vi "BRig_RT_start_v1,13__PortC.vi"() -> ()   [LabVIEW 2014]
uses:
  myRIO_BRig_RT__Case_Exp_stateList.ctl
  myRIO_BRig_RT__Case_NonExp_stateList.ctl
  <vilib>/WebDAVClient/Advanced/SessionHandle.ctl
  <vilib>/Platform/TimedLoop/XDataNode/timing_clust.ctl
  <vilib>/Platform/TimedLoop/XDataNode/nitl_modes.ctl
  <vilib>/Platform/TimedLoop/XDataNode/wakeup.ctl
  <vilib>/myRIO/Common/Instrument Driver Framework/myRIO v1.0/UART/vis/myRIO v1.0 Close UART.vi
  <vilib>/FPGAPlugInAG/myRIO-1900/niLvFpga_Open_myRIO-1900.vi
  <vilib>/rvi/interface/common/dynamic/niFpgaDynamicAddResources.vi
  <vilib>/Utility/error.llb/Error Cluster From Error Code.vi
  <vilib>/rvi/errors/niLvFpgaAdjustHostInterfaceError.vi
  <vilib>/Utility/file.llb/Read From Spreadsheet File (I64).vi
  <vilib>/Utility/file.llb/Write To Spreadsheet File (DBL).vi
  <vilib>/FPGAPlugInAG/Dynamic/niLvFpga_Close_Dynamic.vi
  <vilib>/myRIO/Common/Instrument Driver Framework/Utilities/vis/FPGA Ref Manager.vi
  <vilib>/myRIO/Common/Instrument Driver Framework/myRIO v1.0/myRIO v1.0 Reset FPGA.vi
  <vilib>/myRIO/Common/Instrument Driver Framework/myRIO v1.0/IRQ/vis/myRIO v1.0 IRQ Info FGV.vi
  <vilib>/myRIO/Common/Instrument Driver Framework/myRIO v1.0/IRQ/vis/myRIO v1.0 Timer IRQ Info FGV.vi
  <vilib>/myRIO/Common/Instrument Driver Framework/myRIO v1.0/IRQ/vis/myRIO v1.0 ISR Agent.vi
  <vilib>/rvi/interface/nirviOpenFPGA/nirviOpenFPGA.xnode
  BRig_FPGA_v3,93__PortC__build.lvbitx
  BRig_FPGA_v3,93__PortC.vi
  <vilib>/rvi/interface/nirviReadWriteControl/nirviReadWriteControl.xnode
  <vilib>/Platform/TimedLoop/XDataNode/XDataNode.xnode
  <vilib>/rvi/interface/nirviCloseFPGA/nirviCloseFPGA.xnode
  <vilib>/Platform/TimedLoop/XDataNode/XDNodeRunTimeDep.lvlib
  <vilib>/rvi/interface/Simulation/niFpgaSimulationCallBeginRW.vi
  <vilib>/myRIO/Instrument Drivers/Utilities/Utilities.lvlib
  NiFpgaLv.dll
  <vilib>/WebDAVClient/NI_WebDAV.lvlib
panel:
  out "Solenoid R":bool
  out "Solenoid L":bool
  out "Laser2":bool
  out "Laser1":bool
  out "FreeReward_c_R":u16
  out "FreeReward_c_L":u16
  in  "Laser2_LED":bool
  in  "Laser1_LED":bool
  in  "lick_Rising(F)_or_Falling(T)":bool
  out "T_ExpRun_min":dbl
  out "stop_TimedLoop":bool
  out "BTPR_avg_R":dbl
  out "T2R_avg_R":dbl
  out "BTPR_avg_L":dbl
  out "T2R_avg_L":dbl
  out "BTPR_block":u16
  out "T2R_block":u16
  in  "comm_WebDAV_connect":bool
  in  "I_sendData":bool
  in  "comm_TCP_connect":bool
  out "nRewards_total":u16 caption="# Rewards in Current Block"
  out "BUR_target":u16 caption="Target Trials Per Block"
  in  "input_Threshold_reset":bool
  out "nTrial":u16
  out "allReward_R":bool
  out "allReward_L":bool
  out "Threshold":bool
  out "tLoop":dbl format="%#_2g"
  out "L_Power_l2":dbl
  out "comm_TCP":bool
  in  "get_countPerMS":bool
  out "SolenoidReward":bool
  out "L_Power_l1":dbl caption="LaserPower"
  in  "Recording":bool
  out "FPGA_count2ms":dbl=159.0
  out "error out":errorcluster
  out "cSpout":enum16{"Left", "Right"}(ring) caption="Left or Right Spout"
  out "A4":u32 caption="LickCounter_Right"
  out "A2":u32 caption="LickCounter_Left"
  out "nRewards_Right":u16 caption="# Rewards Total (Right)"
  out "nRewards_Left":u16 caption="# Rewards Total (Left)"
  out "nRewards_cur":u16 caption="# Rewards in Current Block"
  out "TpB_target":u16 caption="Target Trials Per Block"
  out "cState_NonExp":T1 caption="WarmUp State"
  out "iBlock":u16 caption="Current Block"
  out "cState":T2 caption="Experimental State"
  out "iTrial":u16 caption="Current Trial"
  in  "Data Set Prefix":string="Exp1_TM2"
  out "comm_WebDAV":bool
  in  "Host Password":string="sabalab"
  in  "Host UserName":string="Test2"
  in  "STOP_abort":bool caption="Stop LabView\n(Stops myRio and FPGA)"
  in  "STOP_endBlock":bool caption="Stop Experiment\n@ End of Block"
  in  "STOP_endTrial":bool caption="Stop Experiment\n@ End of Trial"
  in  "START":bool caption="Start Experiment"
  # "Experimental Run"
  # "Recording Rig"
  # "FPGA Conversion\n[counts per ms]"
  # "RealTime Cycle\nShould be <5ms"
  # "STOP experiment at"
  # "Exp Run Time"
  # "Reset"
  # "min"
  # "Communication with Host"
  # "Lick Counter"
  # "Give Water?\n(Reward)"
  # "Experimental State"
  # "Left/Right"
  # "Left           Right"
  # "Direction\n(NonSpecific Licking)"
  # "Block Target"
  # "# Blocks"
  # "L          R"
  # "# Trials"
  # "# Rewards"
  # "Bad Trials\nPost Reward"
  # "Trials 2 Reward"
  # "Block"
  # "# Trials"
  # "# Rewards"
  # "Current\nBlock"
  # "WarmUp State"
  # "avg L"
  # "Total"
  # "# Rewards"
  # "# Trials"
  # "avg R"
  # "Laser Power [V]"
  # "Left           Right"
  # "FreeRewards"
  # "Laser1"
  # "Laser2"
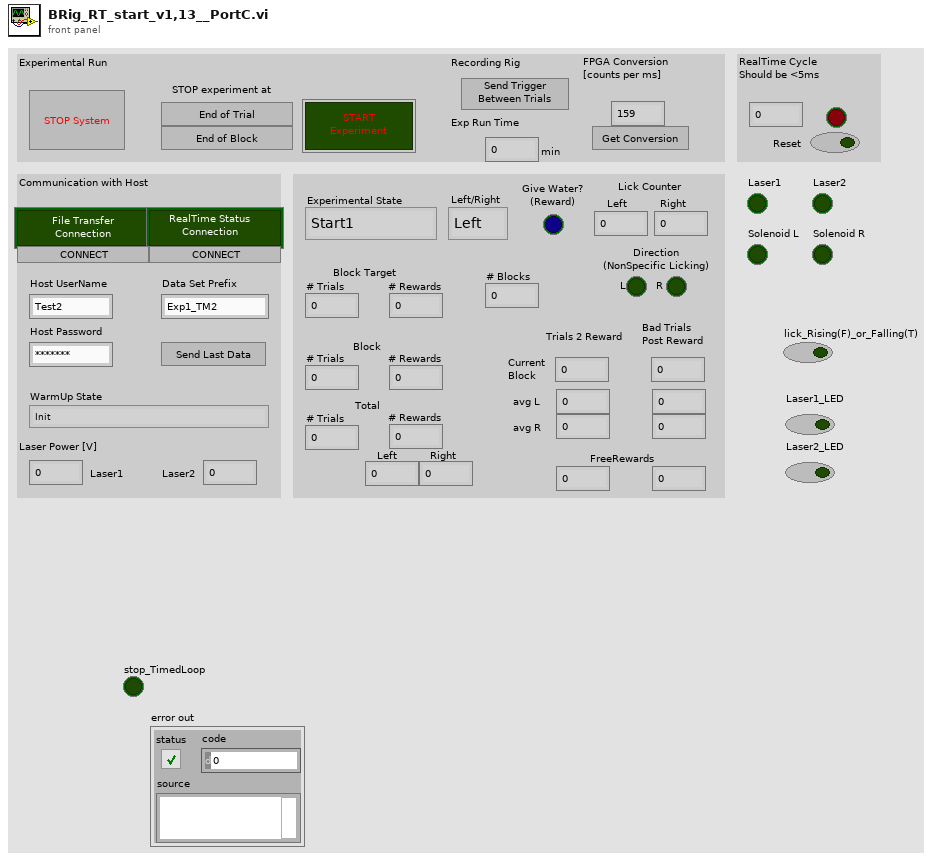
[diagram p1: front panel]
types:
  T1 = typedef "myRIO_BRig_RT__Case_NonExp_stateList.ctl" = enum16{"Init", "UploadSettings_pre", "UploadSettings_Read_dataExp", "UploadSettings_dataExp_1", "UploadSettings_dataExp_2", "UploadSettings_Read_dataLC", "UploadSettings_dataLC_1", "UploadSettings_dataLC_2", "UploadSettings_dataLC_3", "UploadSettings_dataLC_4", "UploadSettings_Read_dataMTrig", "UploadSettings_dataMTrig_1", "UploadSettings_post", "Idle_pre", "IdleEmpty", "IdleEmpty2", "IdleEmpty3", "IdleEmpty4", "Idle", "Idle_2", "Idle_3", "Idle_4", "Idle_5", "Idle_6", "Idle_post", "Cue_pre__pre", "Cue_pre", "Cue", "Cue_LED", "Cue_post", "RewardCalibration_pre", "RewardCalibration", "DispenseWater_pre__pre", "DispenseWater_pre", "DispenseWater", "DispenseWater_post", "TestConnection", "SendData", "Get_FPGA_count_per_ms", "End", "commTCP_connect"}
  T2 = typedef "myRIO_BRig_RT__Case_Exp_stateList.ctl" = enum16{"Start1", "Start2", "Start3", "saveSettings1", "saveSettings2", "saveSettings3", "saveSettings4", "saveSettings_LC_ENL_l1", "saveSettings_LC_ENL_l2", "saveSettings_LC_Cue_l1", "saveSettings_LC_Cue_l2", "saveSettings6_LC_l1_Other", "SaveSettings6_LC_l2_Other", "setSettings_Audio", "setSettings_Laser", "initBlock_pre", "initBlock", "initBlock2", "initBlock_post", "initTrial_pre", "initTrial", "initTrial2", "initTrial3", "initTrial4", "initTrial_LC_ENL1", "initTrial_LC_Cue1", "initTrial_LC_Cue1_2", "initTrial_LC_Sel", "initTrial_post", "ENL1_pre", "ENL1", "ENL1_post", "ENL1Penalty_pre", "ENL1Penalty", "ENL2_pre", "ENL2", "ENL2Penalty_pre", "ENL2Penalty", "Cue1_pre", "Cue1", "Cue1_post", "Cue1Penalty_pre", "Cue1Penalty", "Cue2_pre", "Cue2", "Cue2Penalty_pre", "Cue2Penalty", "Selection_pre", "Selection", "Select_post", "SelectReward_pre", "SelectReward", "SelectRewardPost_pre", "SelectRewardPost", "SelectWrong_pre", "SelectWrong", "SelectWrong_post", "SelectTimeout_pre", "SelectTimeout", "SelectTimeout_post", "endTrial_pre", "endTrial1", "endTrial2", "endTrial3", "endTrial_post", "endBlock_pre", "endBlock", "endBlock_post", "endExp", "commConnect", "commUpload_pre", "commUpload_dataBlock", "commUpload_dataCurrent", "commUpload_dataExp", "commUpload_dataLC", "commUpload_dataTrial", "commUpload_post", "saveData_pre", "saveData_dataBlock", "saveData_dataCurrent", "saveData_dataExp", "saveData_dataLC", "saveData_dataTrial", "saveData_post", "empty_endBlock1", "empty_endBlock2", "empty_endTrial1", "empty_endTrial2", "empty_endTrial3", "empty_endTrial4", "empty_endTrial5", "dummyState", "dummyState_endBlock", "FreeReward_pre", "FreeReward", "FreeRewardPost_pre", "FreeRewardPost"}
  T3 = enum8{"Enabled", "Disabled", "Disabled and Grayed Out"}
  T4 = typedef "NI_WebDAV.lvlib/SessionHandle.ctl" = refnum<k1>
  T5 = typedef "XDNodeRunTimeDep.lvlib/timing_clust.ctl" = cluster{"Expected End [f-1]":u64, "Actual End [f-1]":u64, "Finished Late? [f-1]":bool, "Expected End [i-1]":u64, "Actual End [i-1]":u64, "Finished Late? [i-1]":bool, "Expected Start [i]":u64, "Actual Start [i]":u64, "Expected Start [f]":u64, "Actual Start [f]":u64, "Source Name":string, "Structure Name":string, "Period":i64, "Deadline":i64, "Offset":i64, "Start":i64, "Priority":i32, "Timeout":i32, "Mode":T6, "Wakeup Reason":T7, "Error":errorcluster, "Source Type":string, "Secondary Source Type":string, "Global End Time":u64, "Global Start Time":u64, "Frame Duration":u64, "Iteration Duration":u64, "Assigned CPU":i32, "I/O Scan Engine Mode":u32}
  T6 = typedef "XDNodeRunTimeDep.lvlib/nitl_modes.ctl" = enum32{"No Change", "Process missed periods, maintain original phase", "Discard missed periods, maintain original phase", "Process missed periods, ignore original phase", "Discard missed periods, ignore original phase"}
  T7 = typedef "XDNodeRunTimeDep.lvlib/wakeup.ctl" = enum32{"Normal", "Aborted", "Asynchronous wakeup", "Timing source error", "Timed loop error", "Timeout"}
  T8 = cluster{"read mode":enum16{"polling", "blocking"}, "write mode":enum16{"polling", "blocking"}}
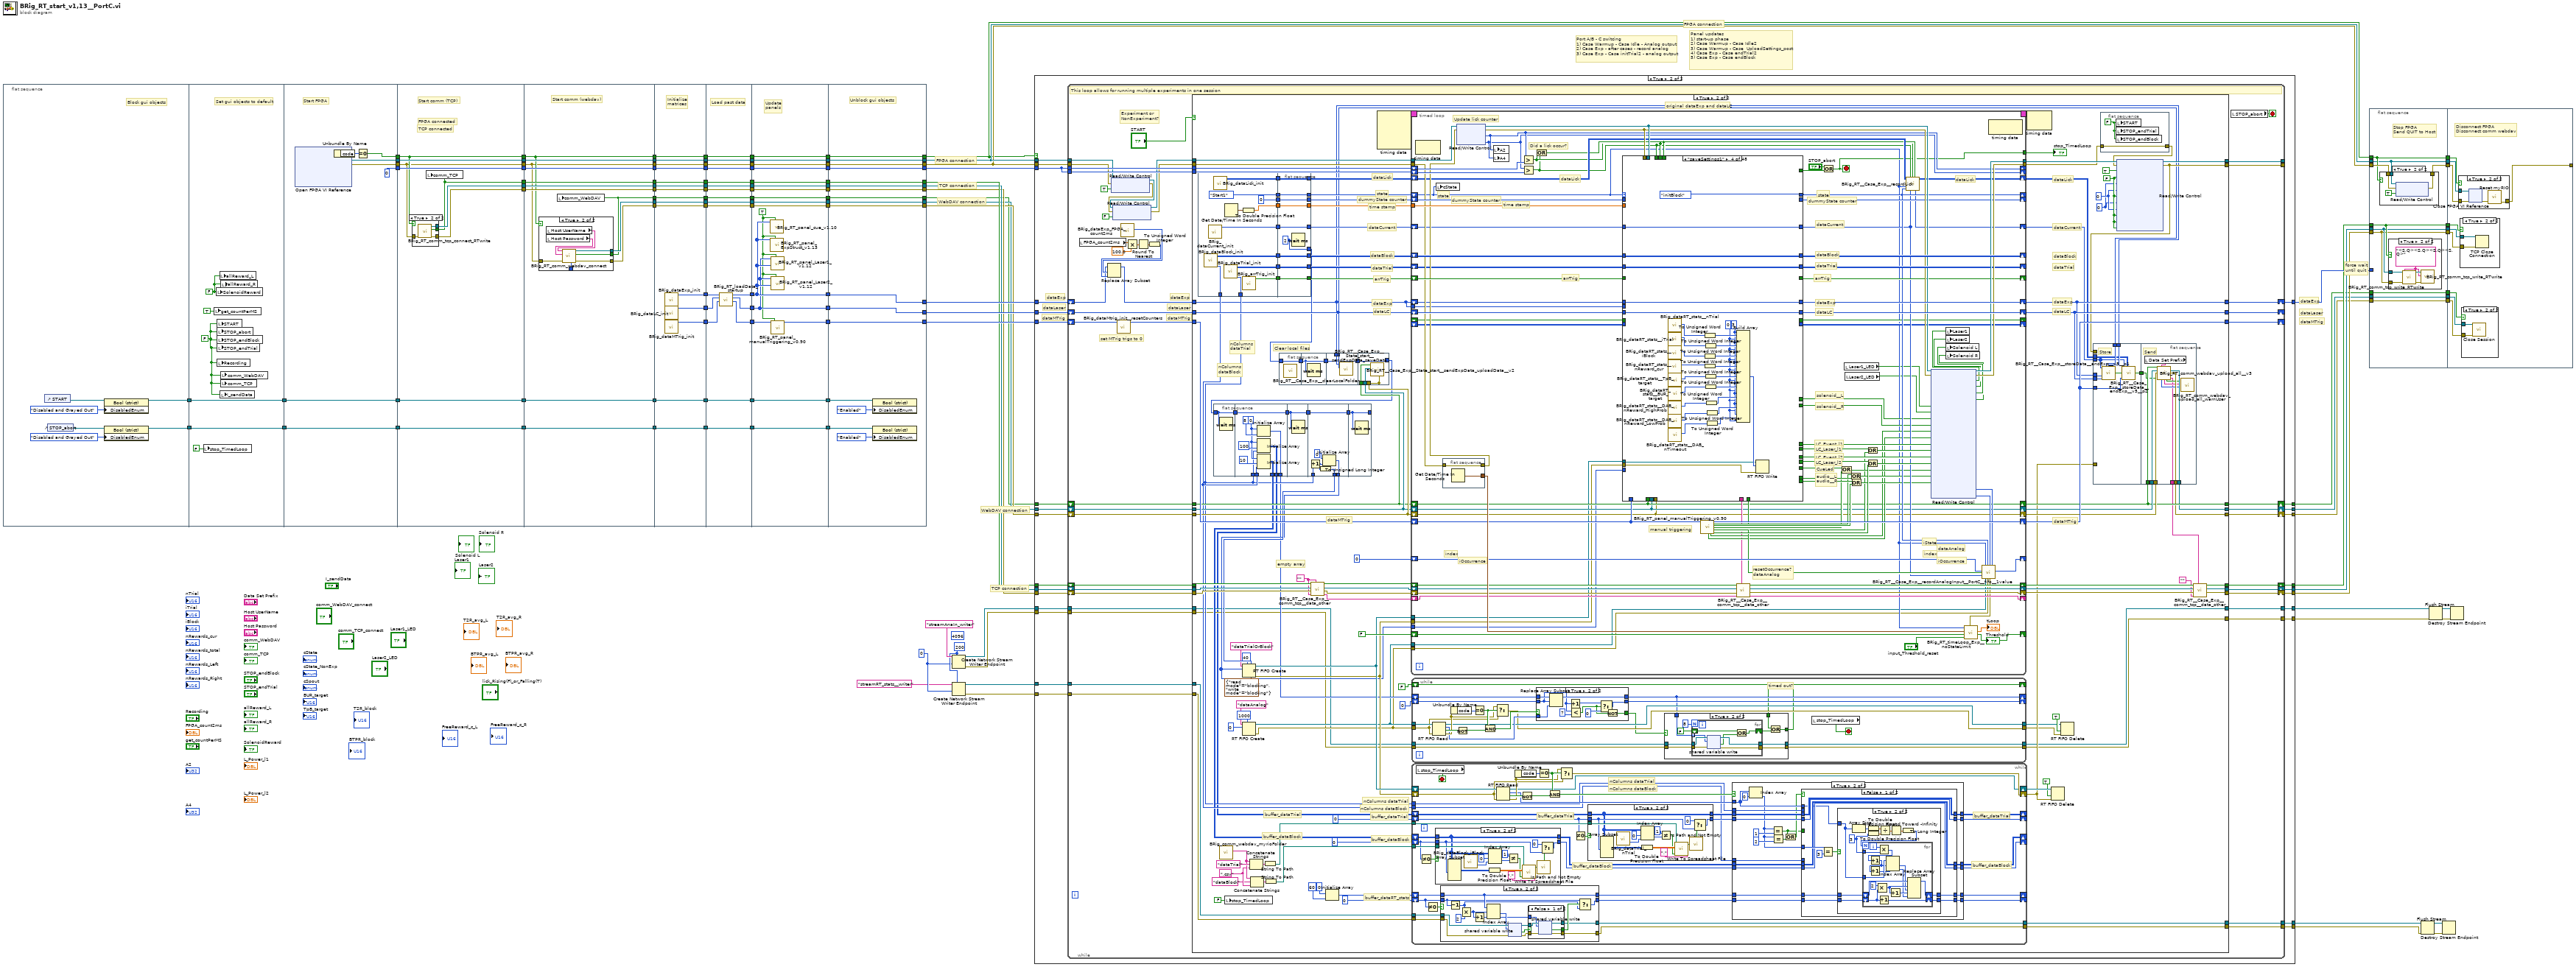
[diagram p0: block diagram]
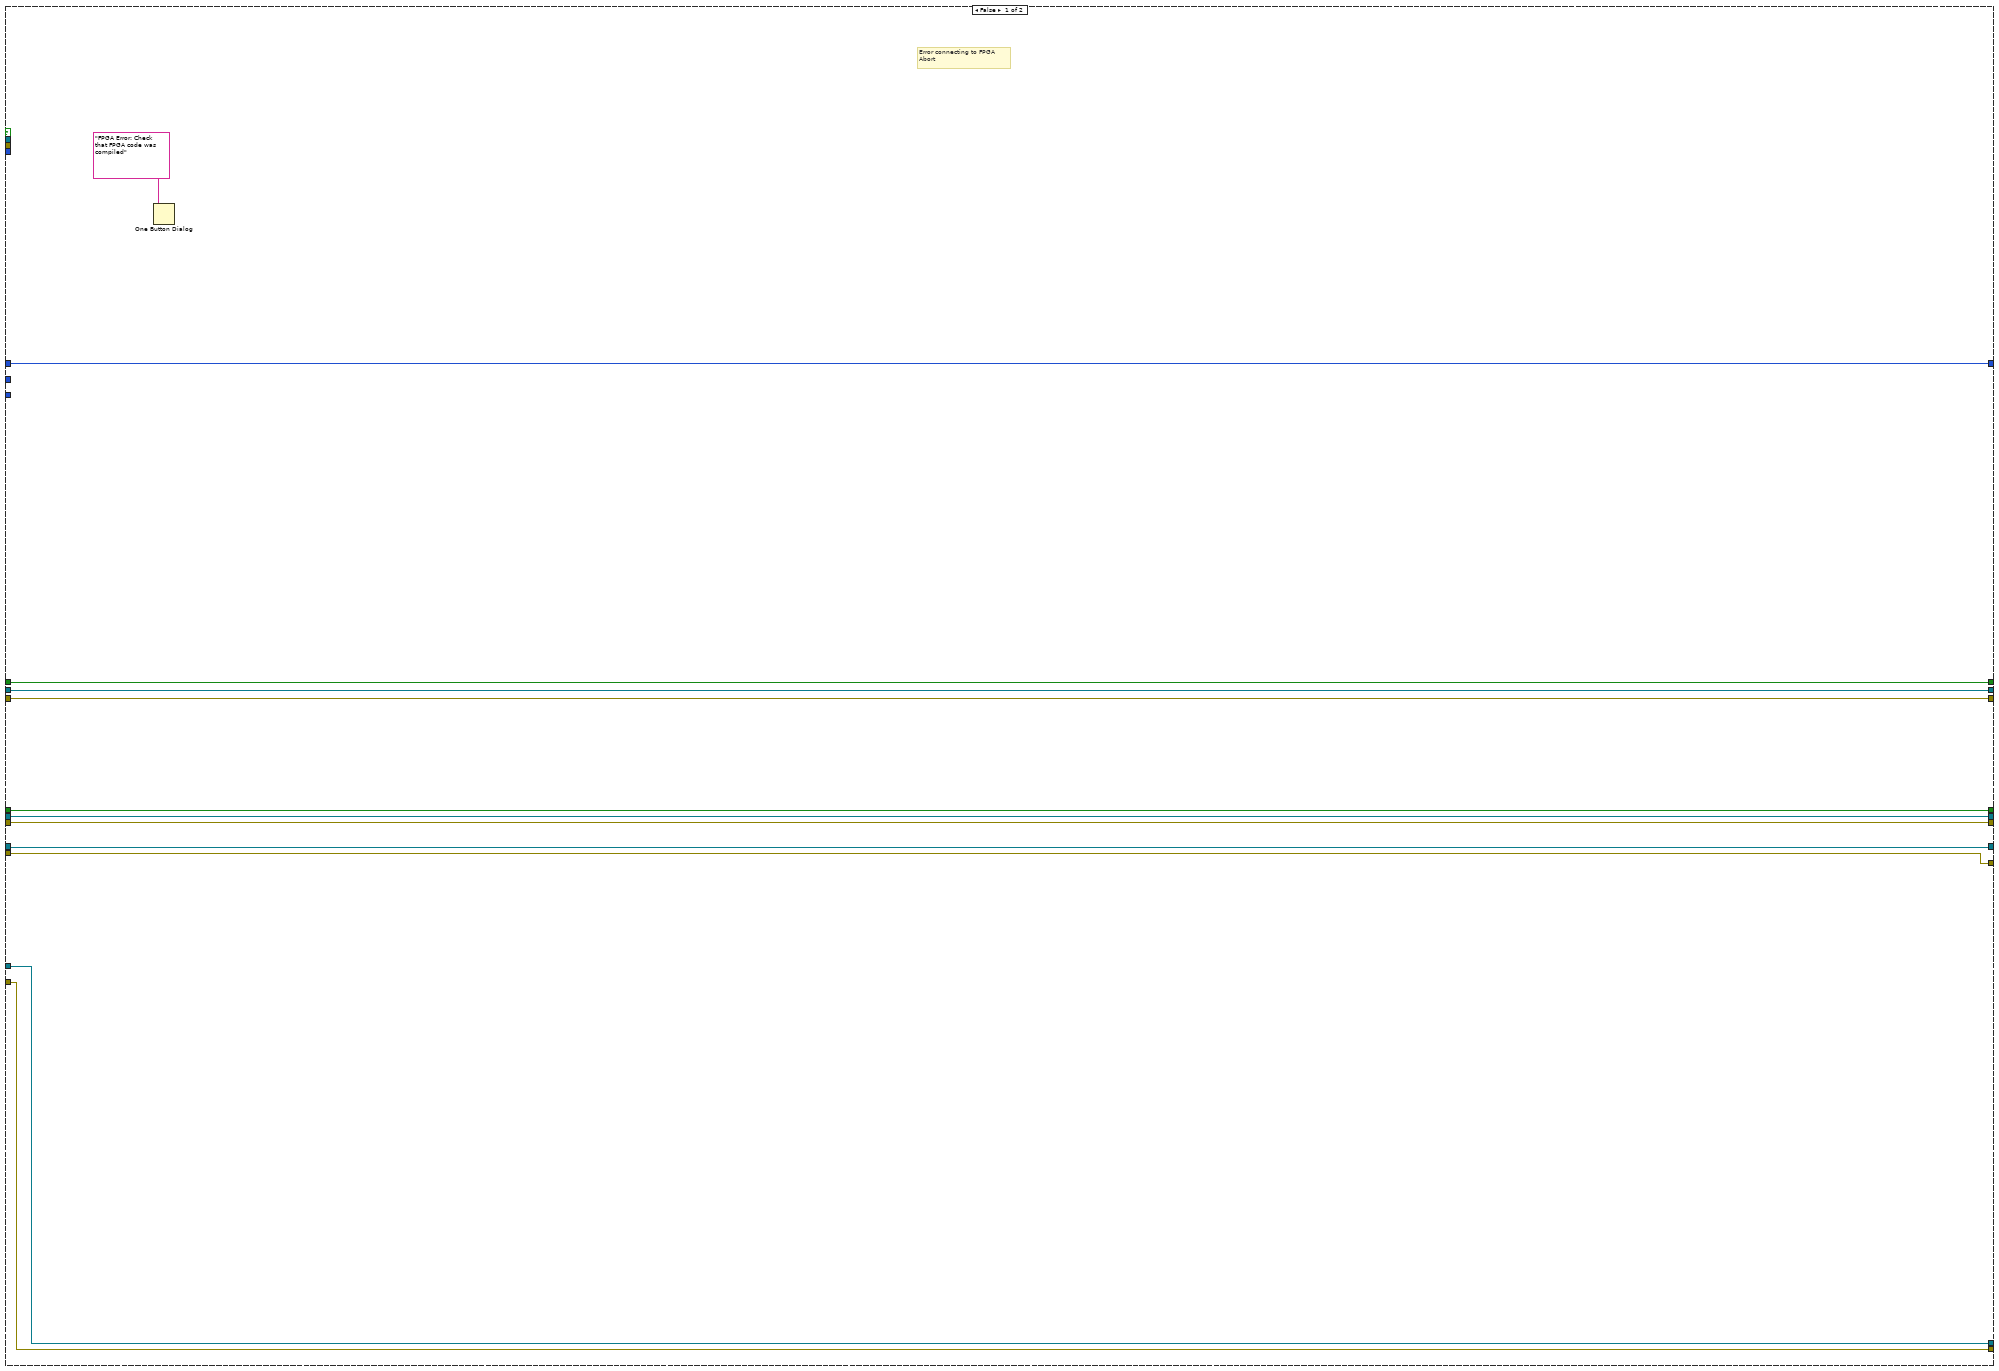
[diagram p2: hidden frame]
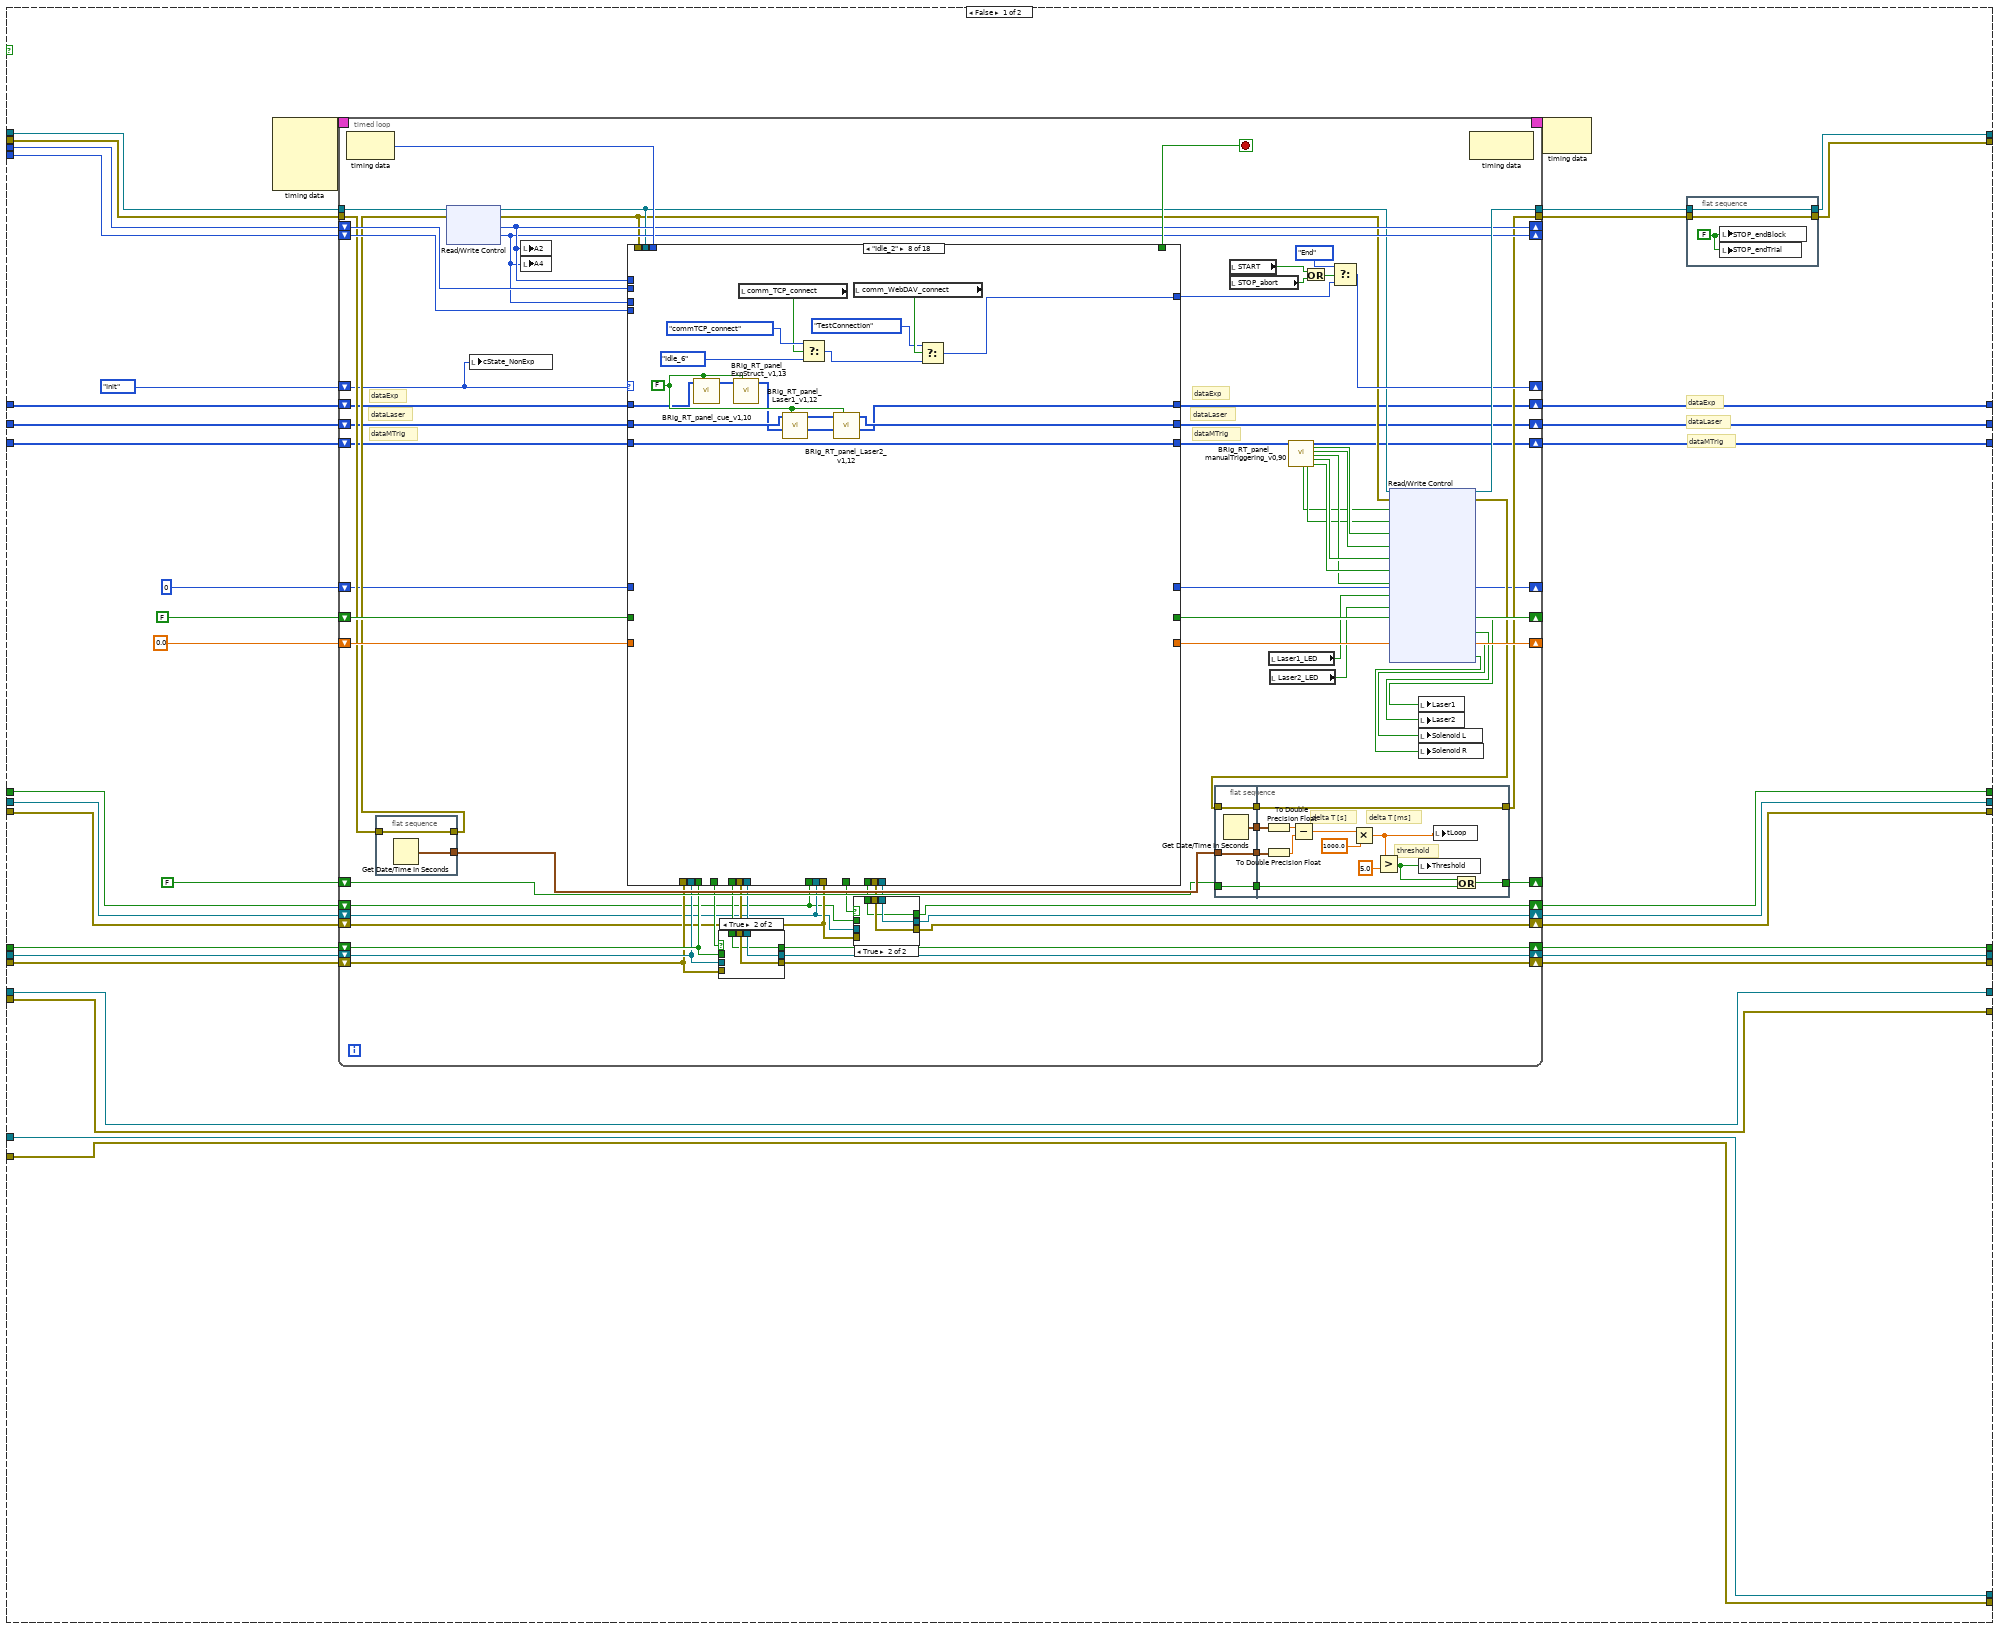
[diagram p3: hidden frame]
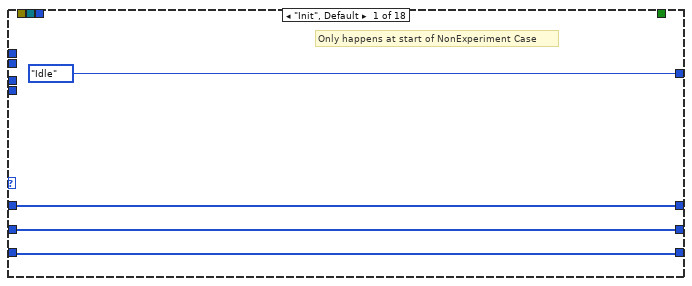
[diagram p6: hidden frame]
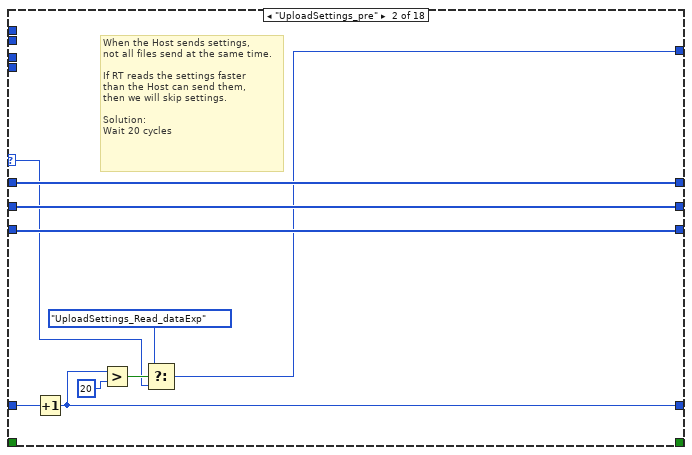
[diagram p7: hidden frame]
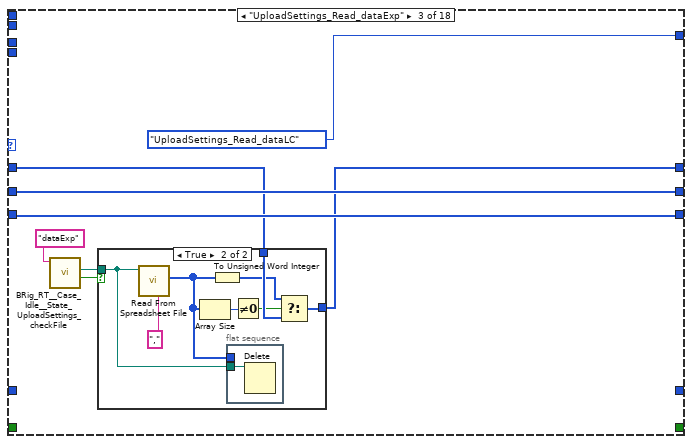
[diagram p8: hidden frame]
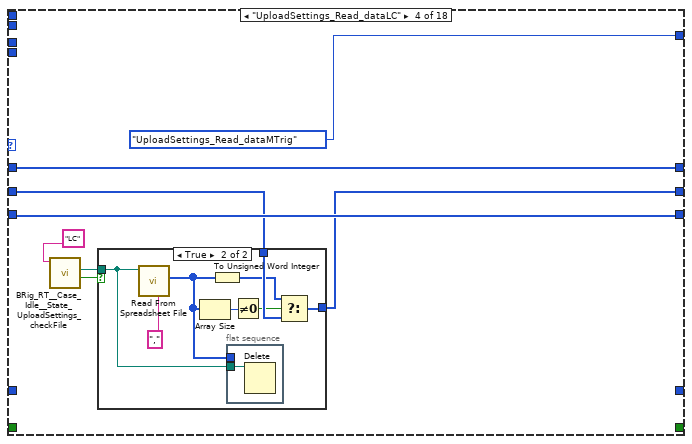
[diagram p10: hidden frame]
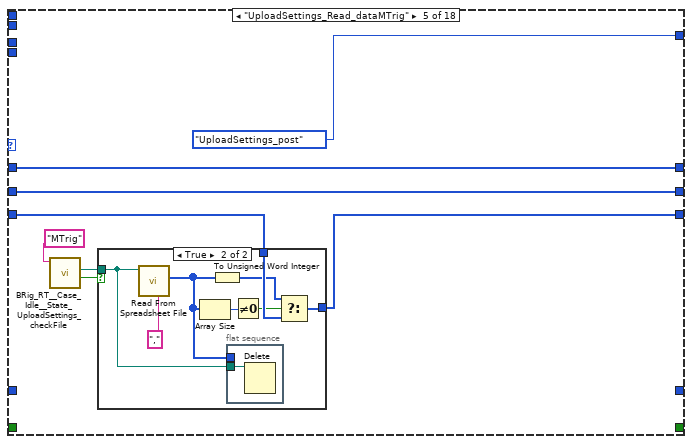
[diagram p12: hidden frame]
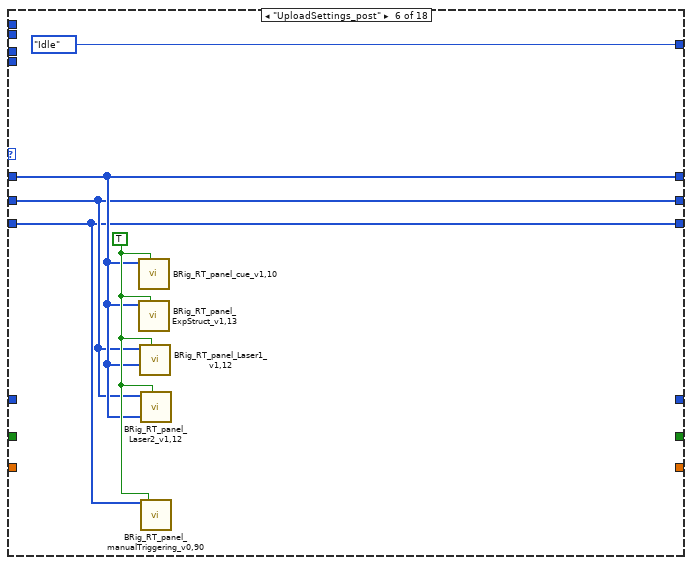
[diagram p14: hidden frame]
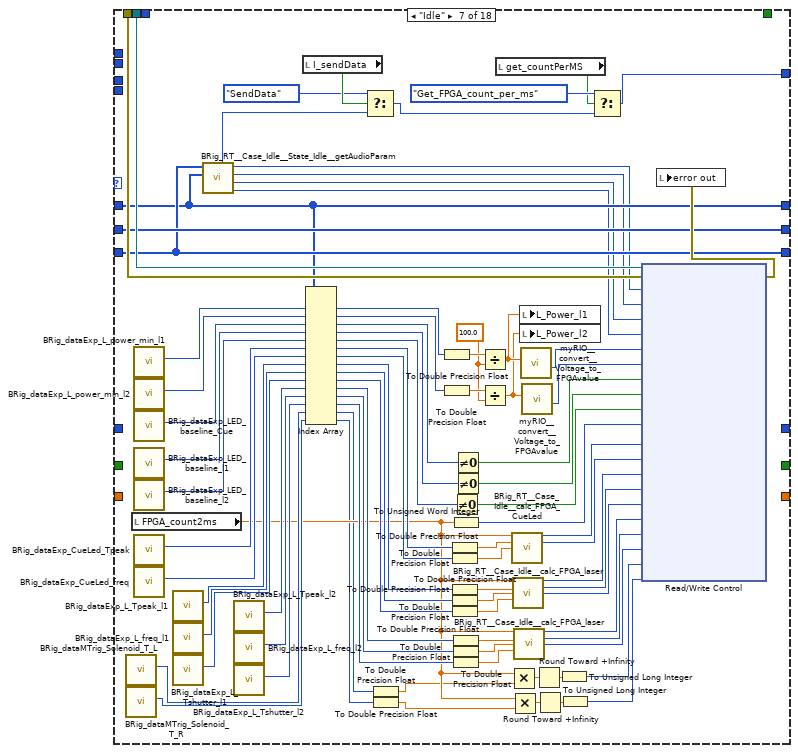
[diagram p15: hidden frame]
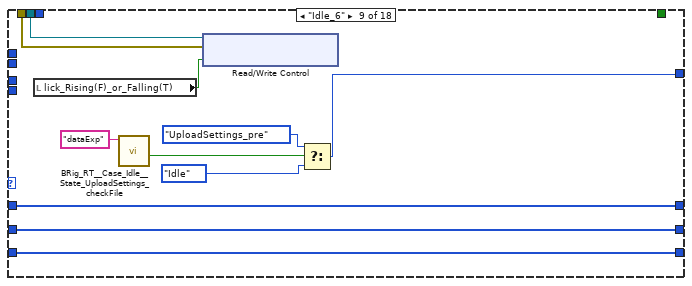
[diagram p16: hidden frame]
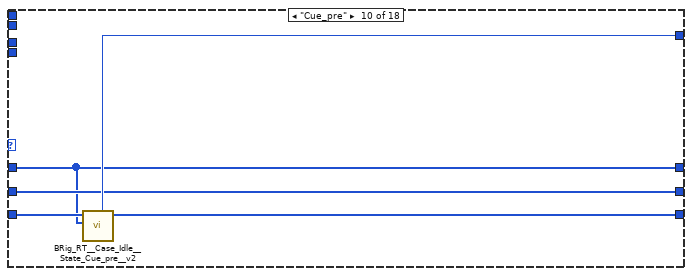
[diagram p17: hidden frame]
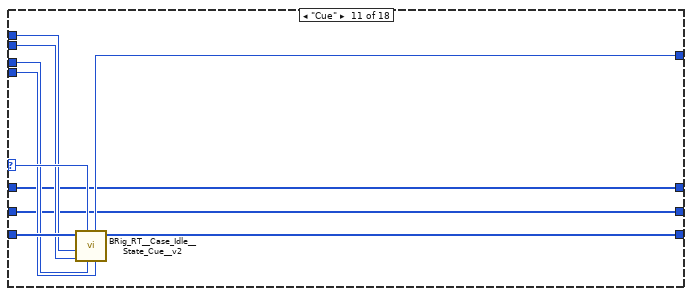
[diagram p18: hidden frame]
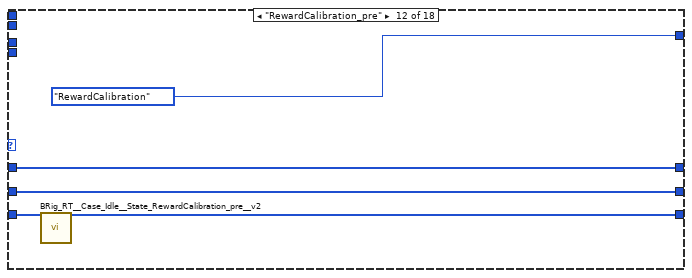
[diagram p19: hidden frame]
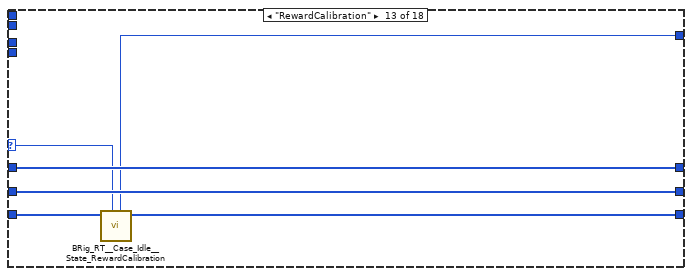
[diagram p20: hidden frame]
diagram:
  w8 = u16 0 ("element")
  (unwired) 4096 ("reader buffer size")
  w9 = 200 ("reader buffer size")
  # "Panel updates\n1) start-up phase\n2) Case Warmup - Case Idle2\n3) Case Warmup - Case  UploadSettings_post\n4) Case Exp - Case endTrial2\n5) Case Exp - Case endBlock"
  # "WebDAV connection"
  # "TCP connection"
  # "WebDAV connection"
  # "TCP connection"
  # "FPGA connection"
  # "FPGA connection"
  # "Port A/B - C switcing\n1) Case Warmup - Case Idle - Analog output\n2) Case Exp - after cases - record analog\n3) Case Exp - Case initTrial2 - analog output"
  # "force wait\nuntil quit"
  # "dataLaser"
  # "dataExp"
  # "dataMTrig"
  n1 = flat-sequence {
    tunnel: [w123] -> w106
    tunnel: [w122] -> w102
    tunnel: [w132] -> w107
    tunnel: w106 -> [w132]
    tunnel: [w131] -> w103
    tunnel: w102 -> [w131]
    tunnel: [w138] -> w120
    tunnel: [w140] -> w119
    tunnel: [u32 0] -> w118
    tunnel: [w136] -> w117
    tunnel: [w135] -> w108
    tunnel: w107 -> [w135]
    tunnel: [w134] -> w104
    tunnel: w103 -> [w134]
    tunnel: w120 -> [w146]
    tunnel: w119 -> [w149]
    tunnel: w118 -> [w148]
    tunnel: w117 -> [w147]
    tunnel: [w146] -> w116
    tunnel: [w149] -> w115
    tunnel: [w148] -> w114
    tunnel: [w147] -> w113
    tunnel: [w141] -> w112
    tunnel: [w145] -> w111
    tunnel: [w144] -> w110
    tunnel: [w143] -> w109
    tunnel: w108 -> [w143]
    tunnel: [w142] -> w105
    tunnel: w104 -> [w142]
    tunnel: w116 -> [w160]
    tunnel: w115 -> [w168]
    tunnel: w114 -> [w167]
    tunnel: w113 -> [w161]
    tunnel: w112 -> [w166]
    tunnel: w111 -> [w165]
    tunnel: w110 -> [w164]
    tunnel: [w160] -> w73
    tunnel: [w168] -> w72
    tunnel: [w167] -> w71
    tunnel: [w161] -> w70
    tunnel: [w166] -> w69
    tunnel: [w165] -> w68
    tunnel: [w164] -> w67
    tunnel: [w163] -> w66
    tunnel: w109 -> [w163]
    tunnel: [w162] -> w65
    tunnel: w105 -> [w162]
    tunnel: [w159] -> w64
    tunnel: [w157] -> w63
    tunnel: [w158] -> w62
    tunnel: w73 -> [w193]
    tunnel: [w193] -> w61
    tunnel: w72 -> [w192]
    tunnel: [w192] -> w60
    tunnel: w71 -> [w191]
    tunnel: [w191] -> w59
    tunnel: w70 -> [w190]
    tunnel: [w190] -> w58
    tunnel: w69 -> [w189]
    tunnel: [w189] -> w57
    tunnel: w68 -> [w188]
    tunnel: [w188] -> w56
    tunnel: w67 -> [w187]
    tunnel: [w187] -> w55
    tunnel: w66 -> [w186]
    tunnel: [w186] -> w54
    tunnel: w65 -> [w185]
    tunnel: [w185] -> w53
    tunnel: w64 -> [w184]
    tunnel: [w184] -> w52
    tunnel: w63 -> [w183]
    tunnel: [w183] -> w51
    tunnel: w62 -> [w182]
    tunnel: [w182] -> w50
    tunnel: [w181] -> w49
    tunnel: [w180] -> w48
    tunnel: [w179] -> w47
    tunnel: w61 -> [w211]
    tunnel: [w211] -> w46
    tunnel: w60 -> [w210]
    tunnel: [w210] -> w44
    tunnel: w59 -> [w209]
    tunnel: [w209] -> w42
    tunnel: w58 -> [w208]
    tunnel: [w208] -> w40
    tunnel: w57 -> [w207]
    tunnel: [w207] -> w38
    tunnel: w56 -> [w206]
    tunnel: [w206] -> w36
    tunnel: w55 -> [w205]
    tunnel: [w205] -> w34
    tunnel: w54 -> [w204]
    tunnel: [w204] -> w32
    tunnel: w53 -> [w203]
    tunnel: [w203] -> w30
    tunnel: w52 -> [w202]
    tunnel: [w202] -> w28
    tunnel: w51 -> [w201]
    tunnel: [w201] -> w26
    tunnel: w50 -> [w200]
    tunnel: [w200] -> w24
    tunnel: w49 -> [w195]
    tunnel: [w194] -> w22
    tunnel: w48 -> [w197]
    tunnel: [w196] -> w20
    tunnel: w47 -> [w199]
    tunnel: [w198] -> w19
    tunnel: w46 -> [w228]
    tunnel: [w228] -> w45
    tunnel: w44 -> [w227]
    tunnel: [w227] -> w43
    tunnel: w42 -> [w226]
    tunnel: [w226] -> w41
    tunnel: w40 -> [w225]
    tunnel: [w225] -> w39
    tunnel: w38 -> [w224]
    tunnel: [w224] -> w37
    tunnel: w36 -> [w223]
    tunnel: [w223] -> w35
    tunnel: w34 -> [w222]
    tunnel: [w222] -> w33
    tunnel: w32 -> [w221]
    tunnel: [w221] -> w31
    tunnel: w30 -> [w220]
    tunnel: [w220] -> w29
    tunnel: w28 -> [w219]
    tunnel: [w219] -> w27
    tunnel: w26 -> [w218]
    tunnel: [w218] -> w25
    tunnel: w24 -> [w217]
    tunnel: [w217] -> w23
    tunnel: w22 -> [w214]
    tunnel: [w213] -> w21
    tunnel: w20 -> [w215]
    tunnel: w19 -> [w216]
    tunnel: [w216] -> w18
    tunnel: [w215] -> w17
    tunnel: [w235] -> w83
    tunnel: [w236] -> w84
    tunnel: [w237] -> w85
    tunnel: [w242] -> w89
    tunnel: [w243] -> w121
    tunnel: [w244] -> w96
    tunnel: [w245] -> w95
    tunnel: w45 -> [w245]
    tunnel: w43 -> [w244]
    tunnel: w41 -> [w243]
    tunnel: w39 -> [w242]
    tunnel: w37 -> [w237]
    tunnel: w35 -> [w236]
    tunnel: w33 -> [w235]
    tunnel: w31 -> [w239]
    tunnel: w29 -> [w238]
    tunnel: w27 -> [w233]
    tunnel: w25 -> [w234]
    tunnel: w23 -> [w232]
    tunnel: [w234] -> w77
    tunnel: [w233] -> w78
    tunnel: [w232] -> w79
    tunnel: [w229] -> w92
    tunnel: [w230] -> w91
    tunnel: [w231] -> w90
    tunnel: w21 -> [w231]
    tunnel: w18 -> [w229]
    tunnel: w17 -> [w230]
    frame #0 {
      # "Block gui objects"
      n2 = control-ref of="START"() -> (w127:refnum<vi>)
      n3 = control-ref of="STOP_abort"() -> (w124:refnum<vi>)
      n4 = property class="Bool (strict)"(reference=w127, "DisabledEnum"=T3."Disabled and Grayed Out" ("Disabled")) -> (reference out=w123:refnum<vi>)  [unwired: 1 in, 1 out]
      n5 = property class="Bool (strict)"(reference=w124, "DisabledEnum"=T3."Disabled and Grayed Out" ("Disabled")) -> (reference out=w122:refnum<vi>)  [unwired: 1 in, 1 out]
    }
    frame #1 {
      w129 = FALSE ("SolenoidReward")
      w130 = FALSE
      # "Set gui objects to default"
      n6 = local write "stop_TimedLoop"(FALSE ("stop_TimedLoop")) -> ()
      n7 = local write "get_countPerMS"(TRUE ("get_countPerMS")) -> ()
      n8 = local write "SolenoidReward"(w129) -> ()
      n9 = local write "START"(w130) -> ()
      n10 = local write "STOP_abort"(w130) -> ()
      n11 = local write "STOP_endBlock"(w130) -> ()
      n12 = local write "STOP_endTrial"(w130) -> ()
      n13 = local write "Recording"(w130) -> ()
      n14 = local write "allReward_L"(w129) -> ()
      n15 = local write "I_sendData"(w130) -> ()
      n16 = local write "comm_WebDAV"(w130) -> ()
      n17 = local write "comm_TCP"(w130) -> ()
      n18 = local write "allReward_R"(w129) -> ()
    }
    frame #2 {
      # "Start FPGA"
      n19 = xnode "Open FPGA VI Reference"() -> ("FPGA VI Reference Out"=w140:refnum<k20>, "error out"=w138:errorcluster)  [unwired: 2 in]
      n20 = Unbundle By Name(w138) -> ("code"=w137:i32)
      n21 = Equal To 0?(x=w137) -> (x = 0?=w136:bool)
    }
    frame #3 {
      # "TCP connected"
      # "Start comm (TCP)"
      # "FPGA connected"
      n22 = case shown="True" w147 {
        selector: w147 -> [w150 _]
        tunnel: w146 -> [w152 w156]
        tunnel: [refnum<k5> refnum ("output_hTCP") w155] -> w145
        tunnel: [w150 w154] -> w141
        tunnel: [w152 w153] -> w144
        frame False {
        }
        frame True {
          n23 = call "BRig_RT_comm_tcp_connect_RTwrite.vi"("input_error"=w156) -> ("output_error"=w153:errorcluster, "output_connected"=w154:bool, "output_hTCP"=w155:refnum<k5>)  [unwired: 8 in]
        }
      }
      n24 = local write "comm_TCP"(w141) -> ()
    }
    frame #4 {
      # "Start comm (webdav)"
      n25 = case shown="True" w161 {
        selector: w161 -> [w170 _]
        tunnel: [w169 w176] -> w159
        tunnel: [w170 w175] -> w157
        tunnel: w160 -> [w171 w174]
        tunnel: [w171 w173] -> w158
        tunnel: [_ w172] -> _
        frame False {
          w169 = T4 refnum items=["Session NI_WebDAV"] ("output_hSession")
        }
        frame True {
          n26 = local read "Host UserName"() -> (w177:string)
          n27 = local read "Host Password"() -> (w178:string)
          n28 = call "BRig_RT_comm_webdav_connect.vi"("input_error"=w174, "input_password"=w178, "input_username"=w177) -> ("output_error"=w173:errorcluster, "output_Iconnected"=w175:bool, "output_hSession"=w176:T4, "output_code"=w172:u8)  [unwired: 5 in]
        }
      }
      n29 = local write "comm_WebDAV"(w157) -> ()
    }
    frame #5 {
      # "Initialize\nmatrices"
      n30 = call "BRig_dataExp_init.vi"() -> ("output_dataExp"=w179:u16[])  [unwired: 11 in]
      n31 = call "BRig_dataLC_init.vi"() -> ("output_dataLC"=w180:u16[])  [unwired: 11 in]
      n32 = call "BRig_dataMTrig_init.vi"() -> ("output_dataMTrig"=w181:u16[])  [unwired: 5 in]
    }
    frame #6 {
      # "Load past data"
      n33 = call "BRig_RT_loadData_startup.vi"("input_dataMTrig"=w195, "input_dataLC"=w197, "input_dataExp"=w199) -> ("output_dataMTrig"=w194:u16[], "output_dataLC"=w196:u16[], "output_dataExp"=w198:u16[])  [unwired: 6 in]
    }
    frame #7 {
      w212 = TRUE ("input_setValues")
      # "Update\npanels"
      n34 = call "BRig_RT_panel_cue_v1,10.vi"("input_setValues"=w212, "input_dataExp"=w216) -> ()  [unwired: 9 in, 1 out]
      n35 = call "BRig_RT_panel_ExpStruct_v1,13.vi"("input_setValues"=w212, "input_dataExp"=w216) -> ()  [unwired: 9 in, 1 out]
      n36 = call "BRig_RT_panel_Laser1_v1,12.vi"("input_setValues"=w212, "input_dataExp"=w216, "input_dataLC"=w215) -> ()  [unwired: 7 in, 2 out]
      n37 = call "BRig_RT_panel_Laser2_v1,12.vi"("input_setValues"=w212, "input_dataExp"=w216, "input_dataLC"=w215) -> ()  [unwired: 7 in, 2 out]
      n38 = call "BRig_RT_panel_manualTriggering_v0,90.vi"("input_dataMTrig"=w214, "input_setValues"=w212) -> ("output_dataMTrig"=w213:u16[])  [unwired: 10 in, 7 out]
    }
    frame #8 {
      # "Unblock gui objects"
      n39 = property class="Bool (strict)"(reference=w239, "DisabledEnum"=T3."Enabled" ("Disabled")) -> ()  [unwired: 1 in, 2 out]
      n40 = property class="Bool (strict)"(reference=w238, "DisabledEnum"=T3."Enabled" ("Disabled")) -> ()  [unwired: 1 in, 2 out]
    }
  }
  n41 = Create Network Stream Writer Endpoint(7:w9, 9:w8, 11:"streamAnaIn_writer" ("reader name")) -> (0:w10:errorcluster, 3:w11:refnum<k21>)  [unwired: 4 in]
  n42 = Create Network Stream Writer Endpoint(7:w9, 9:w8, 11:"streamRT_stats__writer" ("writer name")) -> (0:w5:errorcluster, 3:w6:refnum<k21>)  [unwired: 4 in]
  n43 = case shown="True" w89 {
    tunnel: w121 -> [_ w284]
    tunnel: w96 -> [_ w283]
    tunnel: w95 -> [_ w282]
    tunnel: [w257 w281] -> w93
    tunnel: w92 -> [w257 w280]
    tunnel: w91 -> [_ w279]
    tunnel: w90 -> [_ w278]
    tunnel: w85 -> [w256 w277]
    tunnel: w84 -> [w255 w276]
    tunnel: w83 -> [w254 w275]
    tunnel: [w256 w274] -> w82
    tunnel: [w255 w273] -> w81
    tunnel: [w254 w272] -> w80
    tunnel: w79 -> [w253 w271]
    tunnel: w78 -> [w252 w270]
    tunnel: w77 -> [w251 w269]
    tunnel: [w253 w268] -> w76
    tunnel: [w252 w267] -> w75
    tunnel: [w251 w266] -> w74
    tunnel: [w250 w265] -> w14
    tunnel: [w249 w264] -> w13
    tunnel: w11 -> [w250 w263]
    tunnel: w10 -> [w249 w262]
    tunnel: w6 -> [w247 w261]
    tunnel: w5 -> [w246 w260]
    tunnel: [w247 w259] -> w2
    tunnel: [w246 w258] -> w1
    frame False {
      # "Error connecting to FPGA\nAbort"
      n44 = One Button Dialog(message="FPGA Error: Check that FPGA code was compiled") -> ()  [unwired: 1 in, 1 out]
    }
    frame True {
      # "dataExp"
      # "dataLaser"
      # "dataMTrig"
      n45 = while {
        tunnel: w283 -> [w322]
        tunnel: w282 -> [w327]
        tunnel: w284 -> [w330]
        tunnel: w284 -> [w329]
        tunnel: [w320] -> _
        tunnel: [w319] -> _
        shift-right: [w318] -> _
        shift-left: w278 -> [w315]
        shift-right: [w316] -> _
        shift-left: w279 -> [w317]
        shift-right: [w286] -> w281
        shift-left: w280 -> [w295]
        shift-right: [w310] -> w274
        shift-left: w277 -> [w313]
        shift-right: [w309] -> w273
        shift-left: w276 -> [w312]
        shift-right: [w308] -> w272
        shift-left: w275 -> [w311]
        shift-right: [w304] -> w268
        shift-left: w271 -> [w307]
        shift-right: [w303] -> w267
        shift-left: w270 -> [w306]
        shift-right: [w302] -> w266
        shift-left: w269 -> [w305]
        tunnel: [w294] -> w265
        tunnel: [w293] -> w264
        tunnel: w263 -> [w292]
        tunnel: w262 -> [w291]
        tunnel: w261 -> [w290]
        tunnel: w260 -> [w289]
        tunnel: [w288] -> w259
        tunnel: [w287] -> w258
        stop <- w328 stop-if-true
        # "set MTrig trigs to 0"
        # "dataExp"
        # "dataLaser"
        # "dataMTrig"
        # "Experiment or\nNonExperiment?"
        # "This loop allows for running multiple experiments in one session"
        n46 = local read "FPGA_count2ms"() -> (w299:dbl)
        n47 = xnode "Read/Write Control"("FPGA VI Reference In"=w322, "error in"=w327, "Counts_Reset"=TRUE) -> ("FPGA VI Reference Out"=w324:refnum<k20>, "error out"=w325:errorcluster)
        n48 = xnode "Read/Write Control"("FPGA VI Reference In"=w324, "error in"=w325, "Counts_Reset"=FALSE) -> ("FPGA VI Reference Out"=w321:refnum<k20>, "error out"=w323:errorcluster)
        n49 = call "BRig_dataMtrig_init__resetCounters.vi"("input_dataMTrig"=w315) -> ("output_dataMTrig"=w314:u16[])  [unwired: 10 in]
        n50 = call "BRig_dataExp_FPGA_count2ms.vi"() -> ("output_FPGA_count2ms"=w300:i32)  [unwired: 11 in]
        n51 = Multiply(x=w299, y=100.0) -> (x*y=w297:dbl)
        n52 = Round To Nearest(number=w297) -> (nearest integer value=w296:dbl)
        n53 = To Unsigned Word Integer(number=w296) -> (unsigned 16bit integer=w301:u16)
        n54 = Replace Array Subset(array=w295, new element=w301, index=w300) -> (w285:u16[])
        n55 = case shown="True" "START" {
          tunnel: w330 -> [w366 w941]
          tunnel: w329 -> [w365 w940]
          tunnel: w323 -> [w363 w929]
          tunnel: w321 -> [w364 w930]
          tunnel: [w361 w938] -> w320
          tunnel: [w359 w907] -> w319
          tunnel: w314 -> [w355 w927]
          tunnel: [w354 w913] -> w318
          tunnel: w317 -> [w353 w877]
          tunnel: w285 -> [w333 w830]
          tunnel: [w352 w912] -> w316
          tunnel: [w351 w911] -> w286
          tunnel: w313 -> [w350 w921]
          tunnel: w312 -> [w349 w920]
          tunnel: w311 -> [w348 w919]
          tunnel: [w347 w896] -> w310
          tunnel: [w346 w895] -> w309
          tunnel: [w345 w894] -> w308
          tunnel: w307 -> [w344 w876]
          tunnel: w306 -> [w343 w875]
          tunnel: w305 -> [w342 w874]
          tunnel: [w341 w903] -> w304
          tunnel: [w340 w902] -> w303
          tunnel: [w339 w904] -> w302
          tunnel: w292 -> [w337 w835]
          tunnel: w291 -> [w336 w834]
          tunnel: [w337 w833] -> w294
          tunnel: [w336 w832] -> w293
          tunnel: w290 -> [w335 w826]
          tunnel: w289 -> [w334 w827]
          tunnel: [w335 w821] -> w288
          tunnel: [w334 w820] -> w287
          frame False {
            # "dataExp"
            # "dataLaser"
            # "dataMTrig"
            n56 = node-c288() -> (w369:T5)  [unwired: 4 in]
            n57 = timed-loop {
              timing: w369 -> [_]
              timing-out: [_] -> w368
              shift-right: [w437] -> _
              shift-left: myRIO_BRig_RT__Case_NonExp_stateList."Init" ("Enum") -> [w406]
              shift-right: [w435] -> _
              shift-left: w366 -> [w436]
              shift-right: [w433] -> _
              shift-left: w365 -> [w434]
              tunnel: [w443] -> w362
              tunnel: [w419] -> w360
              tunnel: w363 -> [w426]
              tunnel: w364 -> [w444]
              shift-right: [w429] -> _
              shift-left: FALSE -> [w430]
              shift-right: [w427] -> _
              shift-left: 0.0 -> [w428]
              shift-right: [w416] -> _
              shift-left: FALSE -> [w417]
              shift-right: [w415] -> w354
              shift-left: w355 -> [w407]
              shift-right: [w401] -> w351
              shift-left: w333 -> [w404]
              shift-right: [w402] -> w352
              shift-left: w353 -> [w403]
              shift-right: [w400] -> w347
              shift-left: w350 -> [w396]
              shift-right: [w399] -> w346
              shift-left: w349 -> [w395]
              shift-right: [w398] -> w345
              shift-left: w348 -> [w394]
              shift-right: [w384] -> w341
              shift-left: w344 -> [w390]
              shift-right: [w385] -> w340
              shift-left: w343 -> [w389]
              shift-right: [w386] -> w339
              shift-left: w342 -> [w388]
              shift-right: [w379] -> _
              shift-left: u16 0 ("y") -> [w380]
              stop <- w446 stop-if-true
              # "dataExp"
              # "dataLaser"
              # "dataExp"
              # "dataLaser"
              # "dataMTrig"
              # "dataMTrig"
              n58 = node-c288() -> (w445:i64)  [unwired: 1 in]
              n59 = flat-sequence {
                tunnel: w426 -> [w475]
                tunnel: [w476] -> w418
                tunnel: [w475] -> w425
                frame #0 {
                  n60 = Get Date/Time In Seconds() -> (seconds since 1Jan1904=w476:timestamp)
                }
              }
              n61 = xnode "Read/Write Control"("FPGA VI Reference In"=w444, "error in"=w425) -> ("FPGA VI Reference Out"=w432:refnum<k20>, "error out"=w431:errorcluster, "A2_LickL"=w435:u32, "A4_LickR"=w433:u32)
              n62 = local write "cState_NonExp"(w406) -> ()
              n63 = local write "A2"(w435) -> ()
              n64 = local write "A4"(w433) -> ()
              n65 = case shown="\"Idle_2\"" w406 {
                selector: w406 -> [_ w483 _ _ _ _ _ _ _ _ w674 _ w682 _ _ w726 w769 w775]
                tunnel: [myRIO_BRig_RT__Case_NonExp_stateList."Idle" ("Enum") w484 myRIO_BRig_RT__Case_NonExp_stateList."UploadSettings_Read_dataLC" ("t") myRIO_BRig_RT__Case_NonExp_stateList."UploadSettings_Read_dataMTrig" ("t") myRIO_BRig_RT__Case_NonExp_stateList."UploadSettings_post" ("t") myRIO_BRig_RT__Case_NonExp_stateList."Idle" ("t") w565 w637 w657 w663 w672 myRIO_BRig_RT__Case_NonExp_stateList."RewardCalibration" ("Enum") w681 myRIO_BRig_RT__Case_NonExp_stateList."Idle" ("Enum") myRIO_BRig_RT__Case_NonExp_stateList."Idle" ("Enum") w725 w769 w776] -> w438
                tunnel: [w479 w490 w498 w516 w530 w545 w577 w649 w655 w664 w673 w676 w683 w697 w709 w735 w767 w784] -> w405
                tunnel: [_ _ _ _ _ _ _ _ _ _ _ _ _ _ _ _ TRUE _] -> w446
                tunnel: w407 -> [w479 w490 w498 w516 w527 w545 w577 w649 w655 w665 w675 w677 w684 w697 w709 w735 w767 w784]
                tunnel: w445 -> [_ _ _ _ _ _ _ _ _ _ _ _ _ _ _ _ _ _]
                tunnel: w436 -> [_ _ _ _ _ _ _ _ _ _ w670 _ _ _ _ _ _ _]
                tunnel: w435 -> [_ _ _ _ _ _ _ _ _ _ w671 _ _ _ _ _ _ _]
                tunnel: w434 -> [_ _ _ _ _ _ _ _ _ _ w668 _ _ _ _ _ _ _]
                tunnel: w433 -> [_ _ _ _ _ _ _ _ _ _ w669 _ _ _ _ _ _ _]
                tunnel: w432 -> [_ _ _ _ _ _ w632 _ w652 _ _ _ _ _ _ w730 _ _]
                tunnel: w431 -> [_ _ _ _ _ _ w631 _ w651 _ _ _ _ _ _ w729 _ _]
                tunnel: w430 -> [_ _ _ _ _ _ _ _ _ _ _ _ _ _ _ w734 _ _]
                tunnel: [_ _ _ _ _ _ _ _ _ _ _ _ _ _ _ TRUE _ _] -> w429
                tunnel: w428 -> [_ _ _ _ _ _ _ _ _ _ _ _ _ _ _ w732 _ _]
                tunnel: [_ _ _ _ _ _ _ _ _ _ _ _ _ _ _ w731 _ _] -> w427
                tunnel: w404 -> [w477 w488 w493 w515 w534 w547 w576 w636 w653 w661 w666 w679 w685 w694 w706 w722 w765 w782]
                tunnel: w403 -> [w478 w489 w497 w509 w531 w546 w578 w648 w654 w662 w667 w678 w686 w695 w707 w723 w766 w783]
                tunnel: [w478 w489 w497 w512 w531 w546 w578 w644 w654 w662 w667 w678 w686 w695 w707 w723 w766 w783] -> w402
                tunnel: [w477 w488 w492 w515 w534 w547 w576 w633 w653 w661 w666 w679 w685 w694 w706 w722 w765 w782] -> w401
                tunnel: [_ _ _ _ _ _ _ _ _ _ _ _ _ _ _ _ _ TRUE] -> w397
                tunnel: w396 -> [_ _ _ _ _ _ _ _ _ _ _ _ _ _ w700 _ _ w781]
                tunnel: w395 -> [_ _ _ _ _ _ _ _ _ _ _ _ _ _ w702 _ _ w777]
                tunnel: w394 -> [_ _ _ _ _ _ _ _ _ _ _ _ _ _ w701 _ _ w780]
                tunnel: [_ _ _ _ _ _ _ _ _ _ _ _ _ _ _ _ _ w779] -> w393
                tunnel: [_ _ _ _ _ _ _ _ _ _ _ _ _ _ _ _ _ w778] -> w392
                tunnel: [_ _ _ _ _ _ _ _ _ _ _ _ _ _ _ _ _ w770] -> w391
                tunnel: w388 -> [_ _ _ _ _ _ _ _ _ _ _ _ _ _ w699 _ _ _]
                tunnel: w389 -> [_ _ _ _ _ _ _ _ _ _ _ _ _ _ w705 _ _ _]
                tunnel: w390 -> [_ _ _ _ _ _ _ _ _ _ _ _ _ w687 w704 _ _ _]
                tunnel: [_ _ _ _ _ _ _ _ _ _ _ _ _ TRUE _ _ _ _] -> w387
                tunnel: [_ _ _ _ _ _ _ _ _ _ _ _ _ w689 _ _ _ _] -> w383
                tunnel: [_ _ _ _ _ _ _ _ _ _ _ _ _ w687 _ _ _ _] -> w382
                tunnel: [_ _ _ _ _ _ _ _ _ _ _ _ _ w688 _ _ _ _] -> w381
                tunnel: w380 -> [_ w482 _ _ _ _ _ _ _ _ _ _ _ _ _ _ _ _]
                tunnel: [_ w481 _ _ _ _ _ _ _ _ _ _ _ _ _ _ _ _] -> w379
                frame "Init", Default {
                  # "Only happens at start of NonExperiment Case"
                }
                frame "UploadSettings_pre" {
                  # "When the Host sends settings,\nnot all files send at the same time.\n\nIf RT reads the settings faster\nthan the Host can send them,\nthen we will skip settings.\n\nSolution:\nWait 20 cycles"
                  n66 = Increment(x=w482) -> (x+1=w481:u16)
                  n67 = Greater?(x=w481, y=u16 20) -> (0:w486:bool)
                  n68 = Select(t=myRIO_BRig_RT__Case_NonExp_stateList."UploadSettings_Read_dataExp", s=w486, f=w483) -> (s? t:f=w484:T1)
                }
                frame "UploadSettings_Read_dataExp" {
                  n69 = call "BRig_RT__Case_Idle__State_UploadSettings_checkFile.vi"("input_dataName"="dataExp") -> ("output_Iexist"=w495:bool, "output_dataPath"=w494:path)  [unwired: 9 in]
                  n70 = case shown="True" w495 {
                    tunnel: w494 -> [_ w501]
                    tunnel: w493 -> [w499 w505]
                    tunnel: [w499 w503] -> w492
                    frame False {
                    }
                    frame True {
                      n71 = call-poly <vilib>:"Read From Spreadsheet File.vi"("delimiter (\\t)"="," ("delimiter (\\t)"), "file path (dialog if empty)"=w501) -> ("first row"=w500:i64[])  [unwired: 5 in, 4 out]
                      n72 = Array Size(array=w500) -> (size(s)=w506:i32)
                      n73 = To Unsigned Word Integer(number=w500) -> (unsigned 16bit integer=w504:u16[])
                      n74 = flat-sequence {
                        tunnel: w501 -> [w508]
                        tunnel: w500 -> [_]
                        frame #0 {
                          n75 = Delete(path (use dialog)=w508) -> ()  [unwired: 4 in, 3 out]
                        }
                      }
                      n76 = Not Equal To 0?(x=w506) -> (x != 0?=w502:bool)
                      n77 = Select(t=w504, s=w502, f=w505) -> (s? t:f=w503:u16[])
                    }
                  }
                }
                frame "UploadSettings_Read_dataLC" {
                  n78 = call "BRig_RT__Case_Idle__State_UploadSettings_checkFile.vi"("input_dataName"="LC") -> ("output_Iexist"=w510:bool, "output_dataPath"=w511:path)  [unwired: 9 in]
                  n79 = case shown="True" w510 {
                    tunnel: w511 -> [_ w519]
                    tunnel: w509 -> [w517 w523]
                    tunnel: [w517 w521] -> w512
                    frame False {
                    }
                    frame True {
                      n80 = call-poly <vilib>:"Read From Spreadsheet File.vi"("delimiter (\\t)"="," ("delimiter (\\t)"), "file path (dialog if empty)"=w519) -> ("first row"=w518:i64[])  [unwired: 5 in, 4 out]
                      n81 = Array Size(array=w518) -> (size(s)=w524:i32)
                      n82 = To Unsigned Word Integer(number=w518) -> (unsigned 16bit integer=w522:u16[])
                      n83 = flat-sequence {
                        tunnel: w519 -> [w526]
                        tunnel: w518 -> [_]
                        frame #0 {
                          n84 = Delete(path (use dialog)=w526) -> ()  [unwired: 4 in, 3 out]
                        }
                      }
                      n85 = Not Equal To 0?(x=w524) -> (x != 0?=w520:bool)
                      n86 = Select(t=w522, s=w520, f=w523) -> (s? t:f=w521:u16[])
                    }
                  }
                }
                frame "UploadSettings_Read_dataMTrig" {
                  n87 = call "BRig_RT__Case_Idle__State_UploadSettings_checkFile.vi"("input_dataName"="MTrig") -> ("output_Iexist"=w528:bool, "output_dataPath"=w529:path)  [unwired: 9 in]
                  n88 = case shown="True" w528 {
                    tunnel: w529 -> [_ w537]
                    tunnel: w527 -> [w535 w541]
                    tunnel: [w535 w539] -> w530
                    frame False {
                    }
                    frame True {
                      n89 = call-poly <vilib>:"Read From Spreadsheet File.vi"("delimiter (\\t)"="," ("delimiter (\\t)"), "file path (dialog if empty)"=w537) -> ("first row"=w536:i64[])  [unwired: 5 in, 4 out]
                      n90 = Array Size(array=w536) -> (size(s)=w542:i32)
                      n91 = To Unsigned Word Integer(number=w536) -> (unsigned 16bit integer=w540:u16[])
                      n92 = flat-sequence {
                        tunnel: w537 -> [w544]
                        tunnel: w536 -> [_]
                        frame #0 {
                          n93 = Delete(path (use dialog)=w544) -> ()  [unwired: 4 in, 3 out]
                        }
                      }
                      n94 = Not Equal To 0?(x=w542) -> (x != 0?=w538:bool)
                      n95 = Select(t=w540, s=w538, f=w541) -> (s? t:f=w539:u16[])
                    }
                  }
                }
                frame "UploadSettings_post" {
                  w548 = TRUE ("input_setValues")
                  n96 = call "BRig_RT_panel_cue_v1,10.vi"("input_setValues"=w548, "input_dataExp"=w547) -> ()  [unwired: 9 in, 1 out]
                  n97 = call "BRig_RT_panel_ExpStruct_v1,13.vi"("input_setValues"=w548, "input_dataExp"=w547) -> ()  [unwired: 9 in, 1 out]
                  n98 = call "BRig_RT_panel_Laser1_v1,12.vi"("input_setValues"=w548, "input_dataExp"=w547, "input_dataLC"=w546) -> ()  [unwired: 7 in, 2 out]
                  n99 = call "BRig_RT_panel_Laser2_v1,12.vi"("input_setValues"=w548, "input_dataExp"=w547, "input_dataLC"=w546) -> ()  [unwired: 7 in, 2 out]
                  n100 = call "BRig_RT_panel_manualTriggering_v0,90.vi"("input_dataMTrig"=w545, "input_setValues"=w548) -> ()  [unwired: 10 in, 8 out]
                }
                frame "Idle" {
                  w622 = 100.0 ("y")
                  n101 = call "BRig_dataMTrig_Solenoid_T_L.vi"() -> ("output_Solenoid_T_L"=w560:i32)  [unwired: 11 in]
                  n102 = call "BRig_dataMTrig_Solenoid_T_R.vi"() -> ("output_Solenoid_T_R"=w559:i32)  [unwired: 11 in]
                  n103 = local read "FPGA_count2ms"() -> (w558:dbl)
                  n104 = call "BRig_dataExp_L_power_min_l1.vi"() -> ("output_L_power_min_l1"=w627:i32)  [unwired: 11 in]
                  n105 = call "BRig_dataExp_L_power_min_l2.vi"() -> ("output_L_power_min_l2"=w626:i32)  [unwired: 11 in]
                  n106 = call "BRig_dataExp_LED_baseline_Cue.vi"() -> ("output_LED_baseline_Cue"=w620:i32)  [unwired: 11 in]
                  n107 = call "BRig_dataExp_LED_baseline_l1.vi"() -> ("output_LED_baseline_l1"=w619:i32)  [unwired: 11 in]
                  n108 = call "BRig_dataExp_LED_baseline_l2.vi"() -> ("output_LED_baseline_l2"=w618:i32)  [unwired: 11 in]
                  n109 = call "BRig_dataExp_CueLed_Tpeak.vi"() -> ("output_CueLed_Tpeak"=w610:i32)  [unwired: 11 in]
                  n110 = call "BRig_dataExp_CueLed_freq.vi"() -> ("output_CueLed_Freq"=w609:i32)  [unwired: 11 in]
                  n111 = call "BRig_dataExp_L_Tpeak_l1.vi"() -> ("output_L_Tpeak_l1"=w602:i32)  [unwired: 11 in]
                  n112 = call "BRig_dataExp_L_freq_l1.vi"() -> ("output_L_freq_l1"=w601:i32)  [unwired: 11 in]
                  n113 = call "BRig_dataExp_L_Tshutter_l1.vi"() -> ("output_L_Tshutter_l1"=w600:i32)  [unwired: 11 in]
                  n114 = call "BRig_RT__Case_Idle__State_Idle__getAudioParam.vi"("input_dataExp"=w576, "input_dataMTrig"=w577) -> ("output_Audio_freq_R"=w572:u8, "output_Audio_amp_R"=w573:u16, "output_Audio_freq_L"=w574:u8, "output_Audio_amp_L"=w575:u16, "output_state"=w571:T1)  [unwired: 5 in]
                  n115 = call "BRig_dataExp_L_Tpeak_l2.vi"() -> ("output_L_Tpeak_l2"=w584:i32)  [unwired: 11 in]
                  n116 = call "BRig_dataExp_L_freq_l2.vi"() -> ("output_L_freq_l2"=w583:i32)  [unwired: 11 in]
                  n117 = call "BRig_dataExp_L_Tshutter_l2.vi"() -> ("output_L_Tshutter_l2"=w582:i32)  [unwired: 11 in]
                  n118 = local read "I_sendData"() -> (w570:bool)
                  n119 = Index Array(array=w576, index #1=w627, index #2=w626, index #3=w620, index #4=w619, index #5=w618, index #6=w610, index #7=w609, index #8=w602, index #9=w601, index #10=w600, index #11=w584, index #12=w583, index #13=w582, index #14=w560, index #15=w559) -> (element #1=w625:u16, element #2=w621:u16, element #3=w617:u16, element #4=w616:u16, element #5=w615:u16, element #6=w606:u16, element #7=w605:u16, element #8=w599:u16, element #9=w598:u16, element #10=w597:u16, element #11=w587:u16, element #12=w586:u16, element #13=w585:u16, element #14=w557:u16, element #15=w556:u16)
                  n120 = Select(t=myRIO_BRig_RT__Case_NonExp_stateList."SendData" ("Enum"), s=w570, f=w571) -> (s? t:f=w567:T1)
                  n121 = To Double Precision Float(number=w557) -> (double precision float=w555:dbl)
                  n122 = To Double Precision Float(number=w556) -> (double precision float=w554:dbl)
                  n123 = To Double Precision Float(number=w625) -> (double precision float=w624:dbl)
                  n124 = To Double Precision Float(number=w621) -> (double precision float=w623:dbl)
                  n125 = To Double Precision Float(number=w606) -> (double precision float=w608:dbl)
                  n126 = To Double Precision Float(number=w605) -> (double precision float=w607:dbl)
                  n127 = To Double Precision Float(number=w599) -> (double precision float=w596:dbl)
                  n128 = To Double Precision Float(number=w598) -> (double precision float=w595:dbl)
                  n129 = To Double Precision Float(number=w597) -> (double precision float=w594:dbl)
                  n130 = To Unsigned Word Integer(number=w558) -> (unsigned 16bit integer=w611:u16)
                  n131 = To Double Precision Float(number=w587) -> (double precision float=w588:dbl)
                  n132 = To Double Precision Float(number=w586) -> (double precision float=w589:dbl)
                  n133 = To Double Precision Float(number=w585) -> (double precision float=w590:dbl)
                  n134 = Not Equal To 0?(x=w615) -> (x != 0?=w612:bool)
                  n135 = Not Equal To 0?(x=w617) -> (x != 0?=w614:bool)
                  n136 = Not Equal To 0?(x=w616) -> (x != 0?=w613:bool)
                  n137 = Divide(x=w624, y=w622) -> (x/y=w551:dbl)
                  n138 = Divide(x=w623, y=w622) -> (x/y=w550:dbl)
                  n139 = local read "get_countPerMS"() -> (w566:bool)
                  n140 = Multiply(x=w558, y=w555) -> (x*y=w564:dbl)
                  n141 = Multiply(x=w558, y=w554) -> (x*y=w562:dbl)
                  n142 = call "BRig_RT__Case_Idle__calc_FPGA_CueLed.vi"("input_FPGA_ms2count"=w558, "input_Tpeak"=w608, "input_Freq"=w607) -> ("output_laser_Npeak"=w604:u32, "output_laser_Nvalley"=w603:u32)  [unwired: 11 in]
                  n143 = call "BRig_RT__Case_Idle__calc_FPGA_laser.vi"("input_FPGA_ms2count"=w558, "input_Tpeak"=w596, "input_Freq"=w595, "input_Tshutter"=w594) -> ("output_laser_Npeak"=w593:u32, "output_laser_Nvalley"=w592:u32, "output_laser_Nshutter"=w591:u32)  [unwired: 9 in]
                  n144 = call "BRig_RT__Case_Idle__calc_FPGA_laser.vi"("input_FPGA_ms2count"=w558, "input_Tpeak"=w588, "input_Freq"=w589, "input_Tshutter"=w590) -> ("output_laser_Npeak"=w581:u32, "output_laser_Nvalley"=w580:u32, "output_laser_Nshutter"=w579:u32)  [unwired: 9 in]
                  n145 = local write "L_Power_l1"(w551) -> ()
                  n146 = local write "L_Power_l2"(w550) -> ()
                  n147 = call "myRIO__convert__Voltage_to_FPGAvalue.vi"("input_voltage"=w551) -> ("output_PortC"=w628:i16)  [unwired: 9 in, 1 out]
                  n148 = call "myRIO__convert__Voltage_to_FPGAvalue.vi"("input_voltage"=w550) -> ("output_PortC"=w629:i16)  [unwired: 9 in, 1 out]
                  n149 = Round Toward +Infinity(x=w564) -> (ceil(x): smallest int >= x=w563:dbl)
                  n150 = Round Toward +Infinity(x=w562) -> (ceil(x): smallest int >= x=w561:dbl)
                  n151 = To Unsigned Long Integer(number=w563) -> (unsigned 32bit integer=w553:u32)
                  n152 = To Unsigned Long Integer(number=w561) -> (unsigned 32bit integer=w552:u32)
                  n153 = Select(t=myRIO_BRig_RT__Case_NonExp_stateList."Get_FPGA_count_per_ms" ("Enum"), s=w566, f=w567) -> (s? t:f=w565:T1)
                  n154 = xnode "Read/Write Control"("FPGA VI Reference In"=w632, "error in"=w631, "audioAmp_L"=w575, "audioFreq_L_kHz"=w574, "audioAmp_R"=w573, "audioFreq_R_kHz"=w572, "AnaOut_0"=w628, "AnaOut_1"=w629, "CueLed_Baseline"=w614, "L1Led_Baseline"=w613, "L2Led_Baseline"=w612, "k1__counter_per_ms"=w611, "CueLed_nPeak"=w604, "CueLed_nValley"=w603, "LC_nPeak_l1"=w593, "LC_nValley_l1"=w592, "LC_nShutter_l1"=w591, "LC_nPeak_l2"=w581, "LC_nValley_l2"=w580, "LC_nShutter_l2"=w579, "Solenoid_nTotal_L"=w553, "Solenoid_nTotal_R"=w552) -> ("error out"=w630:errorcluster)  [unwired: 1 out]
                  n155 = local write "error out"(w630) -> ()
                }
                frame "Idle_2" {
                  w642 = FALSE
                  n156 = call "BRig_RT_panel_cue_v1,10.vi"("input_setValues"=w642, "input_dataExp"=w636) -> ("output_dataExp"=w635:u16[])  [unwired: 9 in]
                  n157 = call "BRig_RT_panel_ExpStruct_v1,13.vi"("input_setValues"=w642, "input_dataExp"=w635) -> ("output_dataExp"=w634:u16[])  [unwired: 9 in]
                  n158 = local read "comm_TCP_connect"() -> (w641:bool)
                  n159 = call "BRig_RT_panel_Laser1_v1,12.vi"("input_setValues"=w642, "input_dataExp"=w634, "input_dataLC"=w648) -> ("output_dataExp"=w643:u16[], "output_dataLC"=w645:u16[])  [unwired: 7 in]
                  n160 = Select(t=myRIO_BRig_RT__Case_NonExp_stateList."commTCP_connect" ("Enum"), s=w641, f=myRIO_BRig_RT__Case_NonExp_stateList."Idle_6" ("Enum")) -> (s? t:f=w639:T1)
                  n161 = call "BRig_RT_panel_Laser2_v1,12.vi"("input_setValues"=w642, "input_dataExp"=w643, "input_dataLC"=w645) -> ("output_dataExp"=w633:u16[], "output_dataLC"=w644:u16[])  [unwired: 7 in]
                  n162 = local read "comm_WebDAV_connect"() -> (w640:bool)
                  n163 = Select(t=myRIO_BRig_RT__Case_NonExp_stateList."TestConnection" ("Enum"), s=w640, f=w639) -> (s? t:f=w637:T1)
                }
                frame "Idle_6" {
                  n164 = local read "lick_Rising(F)_or_Falling(T)"() -> (w650:bool)
                  n165 = call "BRig_RT__Case_Idle__State_UploadSettings_checkFile.vi"("input_dataName"="dataExp") -> ("output_Iexist"=w659:bool)  [unwired: 9 in, 1 out]
                  n166 = xnode "Read/Write Control"("FPGA VI Reference In"=w652, "error in"=w651, "Rising(F)_or_Falling(T)"=w650) -> ()  [unwired: 2 out]
                  n167 = Select(t=myRIO_BRig_RT__Case_NonExp_stateList."UploadSettings_pre" ("Enum"), s=w659, f=myRIO_BRig_RT__Case_NonExp_stateList."Idle") -> (s? t:f=w657:T1)
                }
                frame "Cue_pre" {
                  n168 = call "BRig_RT__Case_Idle__State_Cue_pre__v2.vi"("input_dataExp"=w661, "input_dataMTrig"=w665) -> ("output_dataMTrig"=w664:u16[], "output_state"=w663:T1)  [unwired: 8 in]
                }
                frame "Cue" {
                  n169 = call "BRig_RT__Case_Idle__State_Cue__v2.vi"("input_cLick_R_prev"=w668, "input_cLick_R"=w669, "input_state"=w674, "input_cLick_L_prev"=w670, "input_cLick_L"=w671, "input_dataMTrig"=w675) -> ("output_dataMTrig"=w673:u16[], "output_state"=w672:T1)  [unwired: 4 in]
                }
                frame "RewardCalibration_pre" {
                  n170 = call "BRig_RT__Case_Idle__State_RewardCalibration_pre__v2.vi"("input_dataMTrig"=w677) -> ("output_dataMTrig"=w676:u16[])  [unwired: 26 in]
                }
                frame "RewardCalibration" {
                  n171 = call "BRig_RT__Case_Idle__State_RewardCalibration.vi"("input_state"=w682, "input_dataMTrig"=w684) -> ("output_dataMtrig"=w683:u16[], "output_state"=w681:T1)  [unwired: 8 in]
                }
                frame "TestConnection" {
                  n172 = local read "Host Password"() -> (w690:string)
                  n173 = local read "Host UserName"() -> (w691:string)
                  n174 = call "BRig_RT_comm_webdav_connect.vi"("input_password"=w690, "input_username"=w691) -> ("output_Iconnected"=w689:bool, "output_hSession"=w688:T4)  [unwired: 6 in, 2 out]
                  n175 = local write "comm_WebDAV_connect"(FALSE ("comm_WebDAV_connect")) -> ()
                  n176 = local write "comm_WebDAV"(w689) -> ()
                }
                frame "SendData" {
                  n177 = And(x=w700, y=w699) -> (x .and. y?=w698:bool)
                  n178 = case shown="True" w698 {
                    tunnel: w699 -> [_ w717]
                    tunnel: w705 -> [_ w716]
                    tunnel: w704 -> [_ w715]
                    tunnel: w702 -> [_ w713]
                    tunnel: w701 -> [_ w712]
                    frame False {
                      n179 = One Button Dialog(message="Unable to send data:\n Missing one or more\n connections") -> ()  [unwired: 1 in, 1 out]
                    }
                    frame True {
                      n180 = local read "Data Set Prefix"() -> (w718:string)
                      n181 = call "BRig_RT_comm_webdav_upload_all__v3.vi"("input_I_connected_webdav"=w717, "input_fileName_prefix"=w718, "input_hSession"=w716, "input_error"=w715, "input_True"=TRUE) -> ("output_nFilenames"=w719:i32, "output_arrFilenames"=w720:string[], "output_uploaded"=w721:bool[], "output_strCmd"=w714:string)  [unwired: 5 in, 2 out]
                      n182 = call "BRig_RT_comm_tcp_write_RTwrite.vi"("input_error"=w712, "input_packet"=w714, "input_hTCP"=w713) -> ()  [unwired: 5 in, 4 out]
                      n183 = call "BRig_RT_comm_webdav_upload_all_warnUser.vi"("input_n"=w719, "input_arrFilenames"=w720, "input_arrUploaded"=w721) -> ()  [unwired: 9 in]
                    }
                  }
                  n184 = local write "I_sendData"(FALSE ("I_sendData")) -> ()
                }
                frame "Get_FPGA_count_per_ms" {
                  # "Used to automatically determine how many FPGA cycles in 1 ms"
                  n185 = case shown="True" w734 {
                    selector: w734 -> [w736 _]
                    tunnel: w732 -> [_ w749]
                    tunnel: [w740 w749] -> w731
                    tunnel: w730 -> [w739 w747]
                    tunnel: w729 -> [w738 w746]
                    tunnel: [w737 w744] -> w724
                    tunnel: [w736 w743] -> w728
                    frame False {
                      n186 = Get Date/Time In Seconds() -> (seconds since 1Jan1904=w741:timestamp)
                      n187 = To Double Precision Float(number=w741) -> (double precision float=w740:dbl)
                      n188 = xnode "Read/Write Control"("FPGA VI Reference In"=w739, "error in"=w738, "timeTrial_trig"=TRUE ("timeTrial")) -> ("error out"=w737:errorcluster)  [unwired: 1 out]
                      n189 = local write "get_countPerMS"(w736) -> ()
                    }
                    frame True {
                      w745 = 1.0
                      n190 = Get Date/Time In Seconds() -> (seconds since 1Jan1904=w750:timestamp)
                      n191 = To Double Precision Float(number=w750) -> (double precision float=w751:dbl)
                      n192 = Subtract(x=w751, y=w749) -> (x-y=w748:dbl)
                      n193 = Less Or Equal?(x=w745, y=w748) -> (x <= y?=w743:bool)
                      n194 = case shown="True" w743 {
                        tunnel: w747 -> [_ w764]
                        tunnel: w746 -> [w752 w763]
                        tunnel: w745 -> [_ w754]
                        tunnel: [w752 w753] -> w744
                        frame False {
                        }
                        frame True {
                          n195 = xnode "Read/Write Control"("FPGA VI Reference In"=w764, "error in"=w763) -> ("FPGA VI Reference Out"=w761:refnum<k20>, "error out"=w760:errorcluster, "timeTrial_count"=w755:u32)
                          n196 = Multiply(x=w754, y=1000.0) -> (x*y=w758:dbl)
                          n197 = To Double Precision Float(number=w755) -> (double precision float=w757:dbl)
                          n198 = Divide(x=w757, y=w758) -> (x/y=w759:dbl)
                          n199 = local write "FPGA_count2ms"(w759) -> ()
                          n200 = xnode "Read/Write Control"("FPGA VI Reference In"=w761, "error in"=w760, "timeTrial_trig"=FALSE ("timeTrial")) -> ("error out"=w753:errorcluster)  [unwired: 1 out]
                        }
                      }
                    }
                  }
                  n201 = Select(t=myRIO_BRig_RT__Case_NonExp_stateList."Idle" ("Enum"), s=w728, f=w726) -> (s? t:f=w725:T1)
                  n202 = local write "error out"(w724) -> ()
                }
                frame "End" {
                }
                frame "commTCP_connect" {
                  n203 = local read "comm_TCP_connect"() -> (w774:bool)
                  n204 = case shown="True" w781 {
                    tunnel: w780 -> [w791 w800]
                    tunnel: [w790 w796] -> w778
                    tunnel: [w789 w793] -> w770
                    tunnel: [w788 w794] -> w779
                    tunnel: w777 -> [_ w801]
                    frame False {
                      n205 = call "BRig_RT_comm_tcp_connect_RTwrite.vi"("input_error"=w791) -> ("output_error"=w788:errorcluster, "output_connected"=w789:bool, "output_hTCP"=w790:refnum<k5>)  [unwired: 8 in]
                    }
                    frame True {
                      n206 = call "BRig_RT_comm_tcp_write_RTwrite.vi"("input_error"=w800, "input_packet"="<test>", "input_hTCP"=w801) -> ("output_error"=w795:errorcluster, "output_I_NotDisconnected"=w792:bool, "output_I_write"=w798:bool, "output_hTCP"=w797:refnum<k5>)  [unwired: 5 in]
                      n207 = case shown="False" w798 {
                        selector: w798 -> [_ w812]
                        tunnel: w797 -> [w807 w814]
                        tunnel: [w802 w814] -> w796
                        tunnel: w795 -> [w806 w813]
                        tunnel: [w804 w813] -> w794
                        tunnel: [w803 w812] -> w793
                        tunnel: w792 -> [w808 _]
                        frame False {
                          n208 = case shown="True" w808 {
                            tunnel: w807 -> [_ w811]
                            tunnel: w806 -> [w809 w810]
                            tunnel: [w809 w810] -> w805
                            frame False {
                            }
                            frame True {
                              n209 = TCP Close Connection(connection ID=w811, error in (no error)=w810) -> ()  [unwired: 1 in, 2 out]
                            }
                          }
                          n210 = call "BRig_RT_comm_tcp_connect_RTwrite.vi"("input_error"=w805) -> ("output_error"=w804:errorcluster, "output_connected"=w803:bool, "output_hTCP"=w802:refnum<k5>)  [unwired: 8 in]
                        }
                        frame True {
                        }
                      }
                    }
                  }
                  n211 = Not(x=w774) -> (.not. x?=w773:bool)
                  n212 = Or(x=w773, y=w770) -> (x .or. y?=w772:bool)
                  n213 = case shown="True" w772 {
                    tunnel: [w785 myRIO_BRig_RT__Case_NonExp_stateList."Idle" ("Enum")] -> w776
                    tunnel: w775 -> [w785 _]
                    frame False {
                    }
                    frame True {
                      n214 = local write "comm_TCP_connect"(FALSE) -> ()
                    }
                  }
                  n215 = local write "comm_TCP"(w770) -> ()
                }
              }
              n216 = case shown="True" w397 {
                tunnel: [w455 w456] -> w400
                tunnel: [w454 w457] -> w399
                tunnel: [w453 w458] -> w398
                tunnel: w396 -> [w455 _]
                tunnel: w395 -> [w454 _]
                tunnel: w394 -> [w453 _]
                tunnel: w393 -> [_ w458]
                tunnel: w392 -> [_ w457]
                tunnel: w391 -> [_ w456]
                frame False {
                }
                frame True {
                }
              }
              n217 = case shown="True" w387 {
                tunnel: [w449 w450] -> w386
                tunnel: [w448 w451] -> w385
                tunnel: [w447 w452] -> w384
                tunnel: w388 -> [w449 _]
                tunnel: w389 -> [w448 _]
                tunnel: w390 -> [w447 _]
                tunnel: w382 -> [_ w452]
                tunnel: w381 -> [_ w451]
                tunnel: w383 -> [_ w450]
                frame False {
                }
                frame True {
                }
              }
              n218 = flat-sequence {
                tunnel: w420 -> [w462]
                tunnel: w418 -> [w460]
                tunnel: [w462] -> w424
                tunnel: [w461] -> w423
                tunnel: [w460] -> w422
                tunnel: [w459] -> w421
                tunnel: w417 -> [w459]
                tunnel: [w474] -> w419
                tunnel: w424 -> [w474]
                tunnel: w423 -> [w473]
                tunnel: w422 -> [w471]
                tunnel: w421 -> [w466]
                tunnel: [w465] -> w416
                frame #0 {
                  n219 = Get Date/Time In Seconds() -> (seconds since 1Jan1904=w461:timestamp)
                }
                frame #1 {
                  # "threshold"
                  # "delta T [ms]"
                  # "delta T [s]"
                  n220 = To Double Precision Float(number=w473) -> (double precision float=w472:dbl)
                  n221 = To Double Precision Float(number=w471) -> (double precision float=w470:dbl)
                  n222 = Subtract(x=w472, y=w470) -> (x-y=w469:dbl)
                  n223 = Multiply(x=w469, y=1000.0) -> (x*y=w464:dbl)
                  n224 = Greater?(x=w464, y=5.0) -> (0:w463:bool)
                  n225 = local write "Threshold"(w463) -> ()
                  n226 = local write "tLoop"(w464) -> ()
                  n227 = Or(x=w463, y=w466) -> (x .or. y?=w465:bool)
                }
              }
              n228 = local read "START"() -> (w441:bool)
              n229 = local read "STOP_abort"() -> (w440:bool)
              n230 = local read "Laser1_LED"() -> (w378:bool)
              n231 = local read "Laser2_LED"() -> (w377:bool)
              n232 = call "BRig_RT_panel_manualTriggering_v0,90.vi"("input_dataMTrig"=w405) -> ("output_Solenoid_R"=w408:bool, "output_Solenoid_L"=w409:bool, "output_dataMTrig"=w415:u16[], "output_Audio_L"=w410:bool, "output_Audio_R"=w411:bool, "output_CueLed"=w412:bool, "output_Laser_l1"=w413:bool, "output_Laser_l2"=w414:bool)  [unwired: 11 in]
              n233 = Or(x=w441, y=w440) -> (x .or. y?=w439:bool)
              n234 = Select(t=myRIO_BRig_RT__Case_NonExp_stateList."End" ("Enum"), s=w439, f=w438) -> (s? t:f=w437:T1)
              n235 = xnode "Read/Write Control"("FPGA VI Reference In"=w432, "error in"=w431, "A1_SR"=w408, "A3_SL"=w409, "audioTrigger_L"=w410, "audioTrigger_R"=w411, "LC_Laser_l1"=w413, "LC_Laser_l2"=w414, "CueLed_Event"=w412, "L1Led_ON"=w378, "L2Led_ON"=w377) -> ("FPGA VI Reference Out"=w443:refnum<k20>, "error out"=w420:errorcluster, "fpga_laser1"=w373:bool, "fpga_laser2"=w374:bool, "fpga_solenoid_L"=w375:bool, "fpga_solenoid_R"=w376:bool)
              n236 = local write "Laser1"(w373) -> ()
              n237 = local write "Laser2"(w374) -> ()
              n238 = local write "Solenoid L"(w375) -> ()
              n239 = local write "Solenoid R"(w376) -> ()
              n240 = node-c288() -> ()  [unwired: 1 in, 1 out]
            }
            n241 = node-c288(w368) -> ()  [unwired: 1 out]
            n242 = flat-sequence {
              tunnel: w362 -> [w372]
              tunnel: [w372] -> w361
              tunnel: w360 -> [w371]
              tunnel: [w371] -> w359
              frame #0 {
                w370 = FALSE
                n243 = local write "STOP_endBlock"(w370) -> ()
                n244 = local write "STOP_endTrial"(w370) -> ()
              }
            }
          }
          frame True {
            w884 = ".csv" ("string")
            w914 = ""
            w923 = u8 0
            w924 = u16 0 ("AudioLeft_phase_inc")
            w925 = FALSE
            # "buffer_dataRT_stats"
            # "Clear local files"
            # "empty array"
            # "buffer_dataBlock"
            # "buffer_dataTrial"
            # "nColumns dataBlock"
            # "nColumns dataTrial"
            # "buffer_dataBlock"
            # "buffer_dataTrial"
            # "nColumns\ndataBlock"
            # "nColumns\ndataTrial"
            # "original dataExp and dataLC"
            # "dataLick"
            # "dataTrial"
            # "dataBlock"
            # "dataCurrent"
            # "arrTrig"
            # "time stamp"
            # "dummyState counter"
            # "dataTrial"
            # "dataLick"
            # "dataLC"
            # "dataLC"
            # "dataBlock"
            # "dataMTrig"
            # "dataMTrig"
            # "dataExp"
            # "dataExp"
            # "dataCurrent"
            # "state"
            n245 = flat-sequence {
              tunnel: [w1021] -> w854
              tunnel: [w1020] -> w858
              tunnel: [w1029] -> w872
              tunnel: [w1028] -> w871
              tunnel: [myRIO_BRig_RT__Case_Exp_stateList."Start1" ("Enum")] -> w870
              tunnel: [w1026] -> w869
              tunnel: [u16 0] -> w868
              tunnel: [w1024] -> w867
              tunnel: [w1023] -> w866
              tunnel: [w1022] -> w865
              tunnel: [w1031] -> w880
              tunnel: [w1032] -> w881
              tunnel: [w1033] -> w931
              tunnel: [w1034] -> w933
              tunnel: [w1035] -> w934
              tunnel: [w1036] -> w935
              tunnel: [w1037] -> w936
              tunnel: [w1038] -> w937
              tunnel: w872 -> [w1038]
              tunnel: w871 -> [w1037]
              tunnel: w870 -> [w1036]
              tunnel: w869 -> [w1035]
              tunnel: w868 -> [w1034]
              tunnel: w867 -> [w1033]
              tunnel: w866 -> [w1032]
              tunnel: w865 -> [w1031]
              tunnel: [w1030] -> w863
              frame #0 {
                n246 = call "BRig_dataBlock_init.vi"() -> ("output_nCol"=w1020:i32, "output_dataBlock"=w1022:u16[][])  [unwired: 10 in]
                n247 = call "BRig_dataCurrent_init.vi"() -> ("output_dataCurrent"=w1029:u16[])  [unwired: 11 in]
                n248 = call "BRig_dataLick_init.vi"() -> ("output_dataLick"=w1028:u16[][])  [unwired: 11 in]
                n249 = call "BRig_dataTrial_init.vi"() -> ("output_nCol"=w1021:i32, "output_dataTrial"=w1023:u16[][])  [unwired: 10 in]
                n250 = Get Date/Time In Seconds() -> (seconds since 1Jan1904=w1019:timestamp)
                n251 = To Double Precision Float(number=w1019) -> (double precision float=w1026:dbl)
                n252 = call "BRig_arrTrig_init.vi"() -> ("output_arrTrig"=w1024:bool[])  [unwired: 11 in]
              }
              frame #1 {
                w1030 = u32 2 ("milliseconds to wait")
                n253 = Wait (ms)(milliseconds to wait=w1030) -> ()  [unwired: 1 out]
              }
            }
            n254 = flat-sequence {
              tunnel: w860 -> [w1000]
              tunnel: [w1000] -> w859
              tunnel: w859 -> [w1009]
              tunnel: [w1007] -> w842
              tunnel: [w1006] -> w829
              tunnel: [w1003] -> w857
              tunnel: w858 -> [w1002]
              tunnel: w854 -> [w1001]
              tunnel: [w1009] -> w856
              tunnel: w856 -> [w1011]
              tunnel: [w1011] -> w855
              tunnel: w855 -> [w1017]
              tunnel: w854 -> [w1016]
              tunnel: [w1014] -> w849
              tunnel: [w1012] -> w852
              tunnel: [w1017] -> w853
              tunnel: [w1018] -> _
              tunnel: w853 -> [w1018]
              frame #0 {
                n255 = Wait (ms)(milliseconds to wait=w1000) -> ()  [unwired: 1 out]
              }
              frame #1 {
                w1004 = u16 0 ("element")
                n256 = Initialize Array(w1004, 8 ("dimension size")) -> (w1007:u16[])
                n257 = Initialize Array(w1004, 100 ("dimension size"), w1001) -> (w1006:u16[][])
                n258 = Initialize Array(w1004, 10 ("dimension size"), w1002) -> (w1003:u16[][])
              }
              frame #2 {
                n259 = Wait (ms)(milliseconds to wait=w1011) -> ()  [unwired: 1 out]
              }
              frame #3 {
                n260 = Increment(x=w1016) -> (x+1=w1013:i32)
                n261 = To Unsigned Long Integer(number=w1013) -> (unsigned 32bit integer=w1012:u32)
                n262 = Initialize Array(u16 0 ("element"), w1013) -> (w1014:u16[])
              }
              frame #4 {
                n263 = Wait (ms)(milliseconds to wait=w1018) -> ()  [unwired: 1 out]
              }
            }
            n264 = call "BRig_comm_webdav_myrioFolder.vi"() -> ("output_myrioFolder"=w885:string)  [unwired: 11 in]
            n265 = local write "stop_TimedLoop"(FALSE ("stop_TimedLoop")) -> ()
            n266 = RT FIFO Create(0:"dataTrialOrBlock" ("name (unnamed)"), 1:w849, 4:u32 40 ("size (10)"), 6:w852, 7:T8 {"read mode"=enum."blocking", "write mode"=enum."blocking"} ("r/w modes (polling,polling)")) -> (8:w851:refnum<k33>, 11:w850:errorcluster)  [unwired: 3 in, 1 out]
            n267 = RT FIFO Create(0:"dataAnalog" ("name (unnamed)"), 1:u16 0 ("element"), 4:u32 1000 ("size (10)")) -> (8:w837:refnum<k33>, 11:w836:errorcluster)  [unwired: 5 in, 1 out]
            n268 = Concatenate Strings(w885, "dataTrial" ("input_filename"), w884) -> (w886:string)
            n269 = Concatenate Strings(w885, "dataBlock" ("input_filename"), w884) -> (w887:string)
            n270 = String To Path(string=w886) -> (path=w890:path)
            n271 = String To Path(string=w887) -> (path=w882:path)
            n272 = flat-sequence {
              tunnel: [w1039] -> w864
              tunnel: w863 -> [w1039]
              tunnel: w864 -> [w1040]
              tunnel: [w1040] -> w861
              tunnel: w877 -> [w1043]
              tunnel: w830 -> [w1042]
              tunnel: [w1041] -> w862
              tunnel: w861 -> [w1041]
              tunnel: [w1047] -> _
              tunnel: w876 -> [w1047]
              tunnel: w875 -> [w1046]
              tunnel: w874 -> [w1045]
              tunnel: [w1044] -> w860
              tunnel: w862 -> [w1044]
              frame #0 {
                n273 = call "BRig_RT__Case_Exp__clearLocalFolder.vi"() -> ()  [unwired: 12 in]
              }
              frame #1 {
                n274 = Wait (ms)(milliseconds to wait=w1040) -> ()  [unwired: 1 out]
              }
              frame #2 {
                n275 = call "BRig_RT__Case_Exp__State_start__sendExpData_saveData.vi"("input_dataLC"=w1043, "input_dataExp"=w1042) -> ()  [unwired: 10 in]
              }
              frame #3 {
                n276 = call "BRig_RT__Case_Exp__State_start__sendExpData_uploadData__v2.vi"("input_error"=w1047, "input_hSession"=w1046, "input_connected"=w1045) -> ()  [unwired: 8 in, 1 out]
              }
            }
            n277 = call "BRig_RT__Case_Exp__comm_tcp__data_other.vi"("input_strState"=w914, "input_strAccum"=w914, "input_error"=w919, "input_hTCP"=w920, "input_I_connected_TCP"=w921) -> ("output_strAccum"=w915:string, "output_error"=w916:errorcluster, "output_hTCP"=w917:refnum<k5>, "output_I_connect_TCP"=w918:bool)  [unwired: 3 in]
            n278 = Initialize Array(u16 0 ("element"), 60 ("dimension size")) -> (w824:u16[])
            n279 = node-c288() -> (w943:T5)  [unwired: 4 in]
            n280 = timed-loop {
              timing: w943 -> [_]
              timing-out: [_] -> w942
              shift-right: [w1333] -> _
              shift-left: w935 -> [w1288]
              tunnel: w930 -> [w1377]
              tunnel: w929 -> [w1357]
              shift-right: [w1321] -> _
              shift-left: w941 -> [w1376]
              shift-right: [w1320] -> _
              shift-left: w940 -> [w1375]
              tunnel: [w1368] -> w922
              tunnel: [w1369] -> w939
              shift-right: [w1331] -> w910
              shift-left: w937 -> [w1305]
              shift-right: [w1374] -> w911
              shift-left: w830 -> [w1307]
              shift-right: [w1351] -> w913
              shift-left: w927 -> [w1308]
              shift-right: [w1372] -> _
              shift-left: w880 -> [w1373]
              shift-right: [w1370] -> w912
              shift-left: w877 -> [w1371]
              shift-right: [w1327] -> w909
              shift-left: w936 -> [w1334]
              shift-right: [w1367] -> _
              shift-left: w881 -> [w1306]
              tunnel: w934 -> [w1366]
              shift-right: [w1340] -> _
              shift-left: u16 0 -> [w1339]
              shift-right: [w1360] -> _
              shift-left: w933 -> [w1361]
              shift-right: [w1358] -> _
              shift-left: w931 -> [w1359]
              shift-right: [w1352] -> _
              shift-left: FALSE -> [w1354]
              shift-right: [w1296] -> w901
              shift-left: w918 -> [w1315]
              shift-right: [w1295] -> w900
              shift-left: w917 -> [w1314]
              shift-right: [w1293] -> w899
              shift-left: w916 -> [w1313]
              shift-right: [w1294] -> _
              shift-left: w915 -> [w1312]
              shift-right: [w1302] -> w906
              shift-left: w876 -> [w1302]
              shift-right: [w1304] -> w904
              shift-left: w874 -> [w1304]
              shift-right: [w1303] -> w905
              shift-left: w875 -> [w1303]
              shift-right: [w1301] -> _
              shift-left: _ -> [w1299]
              shift-right: [w1300] -> _
              shift-left: _ -> [w1298]
              tunnel: [w1297] -> w893
              tunnel: w851 -> [w1291]
              tunnel: w850 -> [w1290]
              tunnel: w849 -> [w1289]
              tunnel: w837 -> [w1287]
              tunnel: w836 -> [w1286]
              tunnel: w830 -> [w1285]
              stop <- w1297 stop-if-true
              # "iOccurrence"
              # "index"
              # "resetOccurrence?\ndataAnalog"
              # "dataLick"
              # "dataLick"
              # "dummyState counter"
              # "dummyState counter"
              # "iOccurrence"
              # "arrTrig"
              # "arrTrig"
              # "CueLed"
              # "LC_Laser_l2"
              # "LC_Event_l2"
              # "LC_Laser_l1"
              # "LC_Event_l1"
              # "iState"
              # "dataAnalog"
              # "index"
              # "manual triggering"
              # "dataTrial"
              # "dataBlock"
              # "dataExp"
              # "dataCurrent"
              # "time stamp"
              # "audio__L\naudio__R"
              # "dataLC"
              # "solenoid__R"
              # "solenoid__L"
              # "Did a lick occur?"
              # "Update lick counter"
              # "state"
              # "state"
              n281 = node-c288() -> ()  [unwired: 1 in, 1 out]
              n282 = local write "cState"(w1288) -> ()
              n283 = flat-sequence {
                tunnel: w1357 -> [w1378]
                tunnel: [w1379] -> w1355
                tunnel: [w1378] -> w1356
                frame #0 {
                  n284 = Get Date/Time In Seconds() -> (seconds since 1Jan1904=w1379:timestamp)
                }
              }
              n285 = xnode "Read/Write Control"("FPGA VI Reference In"=w1377, "error in"=w1356) -> ("FPGA VI Reference Out"=w1363:refnum<k20>, "error out"=w1362:errorcluster, "A2_LickL"=w1321:u32, "A4_LickR"=w1320:u32)
              n286 = local write "A2"(w1321) -> ()
              n287 = local write "A4"(w1320) -> ()
              n288 = Greater?(x=w1321, y=w1376) -> (0:w1329:bool)
              n289 = Greater?(x=w1320, y=w1375) -> (0:w1328:bool)
              n290 = Or(x=w1329, y=w1328) -> (x .or. y?=w1330:bool)
              n291 = case shown="\"saveSettings1\"" w1288 {
                selector: w1288 -> [_ _ _ _ _ _ _ _ _ _ _ _ _ _ w1683 w1699 _ w1728 _ _ w1775 w1802 _ w1828 _ w1872 _ w1954 _ w1974 _ _ w2126 w2136 _ _ _ _ w2254 _ w2278 w2309 w2330 w2355 _ w2420 w2430 _]
                tunnel: [myRIO_BRig_RT__Case_Exp_stateList."Start2" ("Enum") myRIO_BRig_RT__Case_Exp_stateList."Start3" ("Enum") myRIO_BRig_RT__Case_Exp_stateList."saveSettings1" ("Enum") myRIO_BRig_RT__Case_Exp_stateList."initBlock" ("Enum") myRIO_BRig_RT__Case_Exp_stateList."initTrial_LC_ENL1" ("Enum") myRIO_BRig_RT__Case_Exp_stateList."initTrial" ("Enum") myRIO_BRig_RT__Case_Exp_stateList."initTrial2" ("Enum") myRIO_BRig_RT__Case_Exp_stateList."setSettings_Laser" ("Enum") myRIO_BRig_RT__Case_Exp_stateList."ENL1_pre" ("Enum") myRIO_BRig_RT__Case_Exp_stateList."initTrial_LC_Cue1" ("Enum") myRIO_BRig_RT__Case_Exp_stateList."initTrial_LC_Sel" ("Enum") myRIO_BRig_RT__Case_Exp_stateList."initTrial4" ("Enum") w1661 w1673 w1681 w1697 myRIO_BRig_RT__Case_Exp_stateList."ENL1Penalty" ("Enum") w1726 w1741 w1753 w1774 w1801 myRIO_BRig_RT__Case_Exp_stateList."Cue1Penalty" ("Enum") w1829 w1845 w1867 myRIO_BRig_RT__Case_Exp_stateList."SelectReward" ("Enum") w1953 myRIO_BRig_RT__Case_Exp_stateList."SelectRewardPost" ("Enum") w1973 myRIO_BRig_RT__Case_Exp_stateList."SelectWrong" ("Enum") myRIO_BRig_RT__Case_Exp_stateList."SelectTimeout" ("Enum") w2125 w2135 myRIO_BRig_RT__Case_Exp_stateList."saveData_dataTrial" ("Enum") w2170 w2205 w2243 w2254 myRIO_BRig_RT__Case_Exp_stateList."initBlock" ("Enum") w2276 w2310 w2329 w2354 myRIO_BRig_RT__Case_Exp_stateList."FreeReward" ("Enum") w2418 w2428 myRIO_BRig_RT__Case_Exp_stateList."FreeRewardPost" ("Enum")] -> w1333
                tunnel: w1330 -> [_ _ _ _ _ _ _ _ _ _ _ _ w1662 w1674 w1682 w1698 _ _ w1742 w1754 w1776 w1803 _ _ _ _ _ _ _ _ _ _ _ _ _ _ _ _ _ _ _ _ _ _ _ _ _ _]
                tunnel: w1329 -> [_ _ _ _ _ _ _ _ _ _ _ _ _ _ _ _ _ _ _ _ _ _ _ _ w1838 w1868 _ _ _ _ _ _ _ _ _ _ _ _ _ _ _ _ _ _ _ _ _ _]
                tunnel: w1328 -> [_ _ _ _ _ _ _ _ _ _ _ _ _ _ _ _ _ _ _ _ _ _ _ _ w1837 w1869 _ _ _ _ _ _ _ _ _ _ _ _ _ _ _ _ _ _ _ _ _ _]
                tunnel: w1305 -> [w1389 w1395 w1437 w1464 w1485 w1539 w1553 w1566 w1596 w1621 w1631 w1648 w1660 w1672 w1690 w1706 w1717 w1725 w1743 w1755 w1777 w1804 w1821 w1827 w1848 w1865 w1906 w1950 w1962 w1972 w2001 w2072 w2124 w2134 w2150 w2176 w2214 w2233 w2253 w2260 w2279 w2312 w2328 w2345 w2390 w2416 w2427 w2438]
                tunnel: w1307 -> [w1380 w1394 w1427 w1462 w1473 w1538 w1541 w1565 w1590 w1620 w1630 w1640 w1654 w1668 w1693 w1709 w1716 w1733 w1740 w1752 w1780 w1807 w1814 w1835 w1836 w1864 w1888 w1952 w1960 w1979 w1984 w2055 w2131 w2141 w2142 w2168 w2212 w2216 w2244 w2257 w2281 w2314 w2340 w2360 w2373 w2421 w2431 w2437]
                tunnel: [w1389 w1395 w1437 w1464 w1485 w1537 w1552 w1568 w1596 w1624 w1638 w1647 w1663 w1675 w1689 w1705 w1718 w1724 w1737 w1749 w1760 w1787 w1820 w1826 w1844 w1866 w1903 w1955 w1961 w1970 w1995 w2066 w2122 w2133 w2152 w2176 w2214 w2233 w2253 w2260 w2279 w2312 w2328 w2345 w2396 w2417 w2426 w2436] -> w1332
                tunnel: [w1380 w1394 w1426 w1462 w1473 w1538 w1541 w1565 w1590 w1620 w1630 w1640 w1654 w1668 w1693 w1709 w1716 w1733 w1740 w1752 w1780 w1807 w1814 w1835 w1836 w1864 w1888 w1952 w1960 w1979 w1984 w2055 w2131 w2141 w2142 w2165 w2212 w2219 w2244 w2257 w2281 w2314 w2340 w2360 w2374 w2421 w2431 w2437] -> w1374
                tunnel: [_ _ _ _ _ _ _ _ _ _ _ _ _ _ _ _ _ _ _ _ _ _ _ _ _ _ _ w1944 _ _ _ _ _ _ _ _ _ _ _ _ _ _ _ _ _ w2410 _ _] -> w1317
                tunnel: [_ _ _ _ _ _ _ _ _ _ _ _ _ _ _ _ _ _ _ _ _ _ _ _ _ _ _ w1943 _ _ _ _ _ _ _ _ _ _ _ _ _ _ _ _ _ w2411 _ _] -> w1316
                tunnel: w1373 -> [w1388 w1392 w1435 w1466 w1498 w1535 w1557 w1582 w1607 w1626 w1637 w1645 w1665 w1677 w1692 w1708 w1713 w1731 w1745 w1757 w1779 w1806 w1819 w1832 w1854 w1876 w1905 w1957 w1966 w1977 w1999 w2070 w2129 w2140 w2146 w2177 w2203 w2235 w2251 w2259 w2261 w2315 w2338 w2358 w2399 w2423 w2433 w2445]
                tunnel: [w1388 w1392 w1435 w1466 w1498 w1534 w1556 w1582 w1607 w1626 w1637 w1645 w1665 w1677 w1692 w1708 w1713 w1731 w1745 w1757 w1779 w1806 w1819 w1832 w1854 w1876 w1904 w1957 w1966 w1977 w1998 w2069 w2129 w2140 w2146 w2177 w2203 w2235 w2251 w2259 w2261 w2315 w2338 w2358 w2399 w2423 w2433 w2445] -> w1372
                tunnel: w1371 -> [w1381 w1393 w1436 w1465 w1493 w1540 w1564 w1583 w1608 w1625 w1632 w1646 w1664 w1676 w1691 w1707 w1714 w1732 w1744 w1756 w1778 w1805 w1818 w1834 w1853 w1877 w1907 w1956 w1969 w1978 w2003 w2074 w2130 w2139 w2159 w2167 w2215 w2237 w2252 w2256 w2280 w2313 w2339 w2359 w2400 w2424 w2434 w2446]
                tunnel: [w1381 w1393 w1436 w1465 w1493 w1540 w1564 w1583 w1608 w1625 w1632 w1646 w1664 w1676 w1691 w1707 w1714 w1732 w1744 w1756 w1778 w1805 w1818 w1834 w1853 w1877 w1907 w1956 w1969 w1978 w2003 w2074 w2130 w2139 w2159 w2166 w2215 w2237 w2252 w2256 w2280 w2313 w2339 w2359 w2400 w2424 w2434 w2446] -> w1370
                tunnel: [_ _ _ _ _ _ _ _ _ _ _ _ _ _ _ _ _ _ _ _ _ _ _ _ _ _ _ _ _ _ _ _ _ _ _ _ _ _ TRUE _ _ _ _ _ _ _ _ _] -> w1335
                tunnel: [_ _ _ _ _ _ _ _ _ _ _ _ _ _ _ _ _ _ _ _ w1762 w1789 _ _ _ _ _ _ _ _ _ _ _ _ _ _ _ _ _ _ _ _ _ _ _ _ _ _] -> w1365
                tunnel: [_ _ _ _ _ _ _ _ _ _ _ _ _ _ _ _ _ _ _ _ w1761 w1788 _ _ _ _ _ _ _ _ _ _ _ _ _ _ _ _ _ _ _ _ _ _ _ _ _ _] -> w1364
                tunnel: w1306 -> [w1386 w1391 w1433 w1463 w1497 w1533 w1560 w1584 w1600 w1627 w1636 w1644 w1659 w1671 w1680 w1696 w1710 w1730 w1739 w1751 w1765 w1792 w1816 w1831 w1852 w1856 w1900 w1951 w1967 w1976 w1997 w2068 w2128 w2138 w2158 w2175 w2213 w2234 w2249 w2258 w2265 w2292 w2337 w2357 w2394 w2422 w2432 w2444]
                tunnel: [w1386 w1391 w1433 w1463 w1497 w1532 w1555 w1567 w1594 w1623 w1635 w1643 w1658 w1670 w1679 w1695 w1710 w1730 w1738 w1750 w1764 w1791 w1816 w1831 w1852 w1855 w1899 w1951 w1967 w1976 w1994 w2065 w2128 w2138 w2157 w2175 w2213 w2234 w2249 w2258 w2265 w2292 w2337 w2357 w2394 w2422 w2432 w2444] -> w1367
                tunnel: w1366 -> [_ _ _ _ _ _ _ _ _ _ _ _ _ _ _ _ _ _ _ _ _ _ _ _ _ _ _ _ _ _ _ _ _ _ w2151 _ _ _ _ _ _ _ _ _ _ _ _ _]
                tunnel: w1363 -> [w1385 _ _ _ w1494 w1527 w1563 w1588 w1605 _ _ w1651 _ _ _ _ _ _ _ _ w1766 w1793 _ _ w1850 w1875 w1898 _ _ _ _ _ _ _ w2154 _ _ _ w2247 _ _ _ _ _ w2380 _ _ _]
                tunnel: w1362 -> [w1384 _ _ _ w1495 w1526 w1554 w1587 w1604 _ _ w1650 _ _ _ _ _ _ _ _ w1767 w1794 _ _ w1851 w1874 w1897 _ _ _ _ _ _ _ w2153 _ _ _ w2246 _ _ _ _ _ w2379 _ _ _]
                tunnel: [_ _ _ _ _ _ _ _ _ _ _ _ _ _ w1688 w1704 _ _ _ _ w1772 w1799 _ _ w1843 w1862 _ _ _ _ _ _ _ _ _ _ _ _ _ _ _ _ _ _ _ _ _ _] -> w1341
                tunnel: [_ _ _ _ _ _ _ _ _ _ _ _ _ _ w1687 w1703 _ _ _ _ w1771 w1798 _ _ w1842 w1861 _ _ _ _ _ _ _ _ _ _ _ _ _ _ _ _ _ _ _ _ _ _] -> w1322
                tunnel: [_ _ _ _ _ _ _ _ TRUE ("Recording") _ _ _ _ _ _ _ _ _ _ _ _ _ _ _ _ _ _ _ _ _ _ _ _ _ _ _ _ _ _ _ _ _ _ _ _ _ _ _] -> w1338
                tunnel: w1361 -> [_ _ _ _ _ _ _ _ _ _ _ _ _ _ _ _ _ _ _ _ _ _ _ _ _ _ _ _ _ _ _ _ _ _ _ _ _ _ _ _ w2277 w2308 w2335 w2342 _ _ _ _]
                tunnel: [_ _ _ _ _ _ _ _ _ _ _ _ _ _ _ _ _ _ _ _ _ _ _ _ _ _ _ _ _ _ _ _ _ _ _ _ _ _ _ _ w2275 w2307 w2333 w2343 _ _ _ _] -> w1360
                tunnel: w1359 -> [_ _ _ _ w1467 _ _ _ w1601 w1628 w1634 w1642 w1656 w1667 w1684 w1700 w1711 w1729 w1736 w1748 w1773 w1800 w1815 w1830 w1839 w1863 _ _ _ _ _ _ _ _ _ _ _ _ _ _ _ _ _ _ _ _ _ _]
                tunnel: [_ _ _ _ w1467 _ _ w1569 w1601 w1622 w1633 w1641 w1655 w1666 w1684 w1700 w1711 w1729 w1735 w1747 w1773 w1800 w1815 w1830 w1839 w1863 _ _ _ _ _ _ _ _ _ _ _ _ _ _ _ _ _ _ _ _ _ _] -> w1358
                tunnel: [_ _ _ _ _ _ _ _ _ _ _ _ _ _ w1686 w1702 _ _ _ _ w1770 w1797 _ _ w1841 w1860 _ _ _ _ _ _ _ _ _ _ _ _ _ _ _ _ _ _ _ _ _ _] -> w1345
                tunnel: [_ _ _ _ _ _ _ _ _ _ _ _ _ _ w1685 w1701 _ _ _ _ w1769 w1796 _ _ w1840 w1859 _ _ _ _ _ _ _ _ _ _ _ _ _ _ _ _ _ _ _ _ _ _] -> w1346
                tunnel: [_ _ _ _ _ _ _ _ _ _ _ _ _ _ _ _ _ _ _ _ w1763 w1790 _ _ _ _ _ _ _ _ _ _ _ _ _ _ _ _ _ _ _ _ _ _ _ _ _ _] -> w1348
                tunnel: [_ _ "<S,S>" ("string") _ _ _ _ _ w1595 _ _ _ _ _ _ _ _ _ _ _ _ _ _ _ _ _ w1901 _ _ _ w1986 w2057 _ _ w2149 _ _ w2229 _ _ _ _ _ _ _ _ _ _] -> w1311
                tunnel: w1308 -> [_ _ _ _ _ _ _ _ _ _ _ _ _ _ _ _ _ _ _ _ _ _ _ _ _ _ _ _ _ _ _ _ _ _ _ _ _ _ _ _ _ _ _ _ w2385 _ _ _]
                tunnel: w1304 -> [_ _ _ _ _ _ _ _ _ _ _ _ _ _ _ _ _ _ _ _ _ _ _ _ _ _ _ _ _ _ _ _ _ _ _ _ _ w2228 _ _ _ _ _ _ _ _ _ _]
                tunnel: w1303 -> [_ _ _ _ _ _ _ _ _ _ _ _ _ _ _ _ _ _ _ _ _ _ _ _ _ _ _ _ _ _ _ _ _ _ _ _ _ _ _ _ _ _ _ _ _ _ _ _]
                tunnel: w1302 -> [_ _ _ _ _ _ _ _ _ _ _ _ _ _ _ _ _ _ _ _ _ _ _ _ _ _ _ _ _ _ _ _ _ _ _ _ _ _ _ _ _ _ _ _ _ _ _ _]
                tunnel: [_ _ _ _ _ _ _ _ _ _ _ _ _ _ _ _ _ _ _ _ _ _ _ _ _ _ _ _ _ _ _ _ _ _ _ w2169 _ _ _ _ _ _ _ _ _ _ _ _] -> w1301
                tunnel: [_ _ _ _ _ _ _ _ _ _ _ _ _ _ _ _ _ _ _ _ _ _ _ _ _ _ _ _ _ _ _ _ _ _ _ w2174 _ _ _ _ _ _ _ _ _ _ _ _] -> w1300
                tunnel: w1299 -> [_ _ _ _ _ _ _ _ _ _ _ _ _ _ _ _ _ _ _ _ _ _ _ _ _ _ _ _ _ _ _ _ _ _ _ w2173 _ _ _ _ _ _ _ _ _ _ _ _]
                tunnel: w1298 -> [_ _ _ _ _ _ _ _ _ _ _ _ _ _ _ _ _ _ _ _ _ _ _ _ _ _ _ _ _ _ _ _ _ _ _ w2164 _ _ _ _ _ _ _ _ _ _ _ _]
                tunnel: w1291 -> [_ _ w1410 w1448 _ w1516 w1548 _ _ _ _ _ _ _ _ _ _ _ _ _ _ _ _ _ _ _ w1886 _ _ _ w1989 w2060 _ _ _ _ _ _ _ _ w2272 w2295 _ _ w2365 _ _ _]
                tunnel: w1290 -> [_ _ w1409 w1447 _ w1517 w1547 _ _ _ _ _ _ _ _ _ _ _ _ _ _ _ _ _ _ _ w1885 _ _ _ w1987 w2058 _ _ _ _ _ _ _ _ w2271 w2294 _ _ w2364 _ _ _]
                tunnel: w1289 -> [_ _ _ _ _ _ _ _ _ _ _ _ _ _ _ _ _ _ _ _ _ _ _ _ _ _ _ _ _ _ _ _ _ _ _ _ _ _ _ _ w2269 w2293 _ _ _ _ _ _]
                tunnel: w1285 -> [_ _ _ _ _ _ _ _ _ _ _ _ _ _ _ _ _ _ _ _ w1759 w1786 _ _ _ _ _ _ _ _ _ _ _ _ _ _ _ _ _ _ _ _ _ _ _ _ _ _]
                frame "Start1", Default {
                  w1383 = FALSE ("SelectionState")
                  n292 = xnode "Read/Write Control"("FPGA VI Reference In"=w1385, "error in"=w1384, "SelectionState"=w1383, "LR_reward_Laser_l1"=w1383, "LR_wrong_Laser_l1"=w1383, "LR_reward_Event_l1"=w1383, "LR_wrong_Event_l1"=w1383, "Left(F)_or_Right(T)"=w1383, "SelectionState"=w1383, "LR_reward_Laser_l2"=w1383, "LR_wrong_laser_l2"=w1383, "LR_reward_Event_l2"=w1383, "LR_wrong_Event_l2"=w1383, "LC_Event_l1"=w1383, "LC_Laser_l1"=w1383, "LC_Laser_l2"=w1383, "LC_Event_l2"=w1383, "CueLed_Event"=w1383) -> ("error out"=w1382:errorcluster)  [unwired: 1 out]
                  n293 = local write "error out"(w1382) -> ()
                }
                frame "Start2" {
                }
                frame "Start3" {
                  w1398 = u16 3 ("element")
                  w1396 = u16 0 ("element")
                  w1423 = u16 0 ("new element/subarray")
                  w1428 = 0.0 ("BTPR_avg_L")
                  w1431 = FALSE ("SolenoidReward")
                  w1429 = u16 0 ("BTPR_block")
                  w1432 = u16 0 ("nRewards_cur")
                  # "Goal:\nPrepare dataCurrent"
                  n294 = call "BRig_dataExp_FreeReward_c_L.vi"() -> ("output_FreeReward_c_L"=w1425:i32)  [unwired: 11 in]
                  n295 = call "BRig_dataExp_FreeReward_c_R.vi"() -> ("output_FreeReward_c_R"=w1424:i32)  [unwired: 11 in]
                  n296 = local write "nRewards_cur"(w1432) -> ()
                  n297 = local write "nRewards_total"(w1432) -> ()
                  n298 = local write "nRewards_Left"(w1432) -> ()
                  n299 = local write "nRewards_Right"(w1432) -> ()
                  n300 = local write "BUR_target"(w1432) -> ()
                  n301 = local write "TpB_target"(w1432) -> ()
                  n302 = local write "iBlock"(w1432) -> ()
                  n303 = local write "iTrial"(w1432) -> ()
                  n304 = local write "nTrial"(w1432) -> ()
                  n305 = local write "SolenoidReward"(w1431) -> ()
                  n306 = local write "allReward_L"(w1431) -> ()
                  n307 = local write "allReward_R"(w1431) -> ()
                  n308 = local write "BTPR_avg_L"(w1428) -> ()
                  n309 = local write "BTPR_avg_R"(w1428) -> ()
                  n310 = local write "T2R_avg_L"(w1428) -> ()
                  n311 = local write "T2R_avg_R"(w1428) -> ()
                  n312 = Replace Array Subset(array=w1427, new element #1=w1423, index #1=w1425, new element #2=w1423, index #2=w1424) -> (w1426:u16[])
                  n313 = call "BRig_dataRT_stats__T2R_cur.vi"() -> ("output_T2R_cur"=w1422:i32)  [unwired: 11 in]
                  n314 = call "BRig_dataRT_stats__BTPR_cur.vi"() -> ("output_BTPR_cur"=w1421:i32)  [unwired: 11 in]
                  n315 = call "BRig_dataRT_stats__T2R_avg_L.vi"() -> ("output_T2R_avg_L__x100"=w1416:i32)  [unwired: 11 in]
                  n316 = call "BRig_dataRT_stats__T2R_avg_R.vi"() -> ("output_T2R_avg_R__x100"=w1415:i32)  [unwired: 11 in]
                  n317 = call "BRig_dataRT_stats__BTPR_avg_L.vi"() -> ("output_BTPR_avg_L__x100"=w1420:i32)  [unwired: 11 in]
                  n318 = call "BRig_dataRT_stats__BTPR_avg_R.vi"() -> ("output_BTPR_avg_R__x100"=w1412:i32)  [unwired: 11 in]
                  n319 = call "BRig_dataRT_stats__nReward.vi"() -> ("output_nReward"=w1407:i32)  [unwired: 11 in]
                  n320 = call "BRig_dataRT_stats__nReward_left.vi"() -> ("output_nReward_left"=w1406:i32)  [unwired: 11 in]
                  n321 = call "BRig_dataRT_stats__nReward_right.vi"() -> ("output_nReward_right"=w1405:i32)  [unwired: 11 in]
                  n322 = local write "FreeReward_c_L"(w1423) -> ()
                  n323 = local write "FreeReward_c_R"(w1423) -> ()
                  n324 = local write "BTPR_block"(w1429) -> ()
                  n325 = local write "T2R_block"(w1429) -> ()
                  n326 = call "BRig_dataRT_stats__FreeReward_c_L.vi"() -> ("output_FreeReward_c_L"=w1401:i32)  [unwired: 11 in]
                  n327 = call "BRig_dataRT_stats__FreeReward_c_R.vi"() -> ("output_FreeReward_c_R"=w1400:i32)  [unwired: 11 in]
                  n328 = To Unsigned Word Integer(number=w1416) -> (unsigned 16bit integer=w1417:u16)
                  n329 = To Unsigned Word Integer(number=w1422) -> (unsigned 16bit integer=w1419:u16)
                  n330 = To Unsigned Word Integer(number=w1415) -> (unsigned 16bit integer=w1414:u16)
                  n331 = To Unsigned Word Integer(number=w1421) -> (unsigned 16bit integer=w1418:u16)
                  n332 = To Unsigned Word Integer(number=w1420) -> (unsigned 16bit integer=w1413:u16)
                  n333 = To Unsigned Word Integer(number=w1412) -> (unsigned 16bit integer=w1411:u16)
                  n334 = To Unsigned Word Integer(number=w1407) -> (unsigned 16bit integer=w1404:u16)
                  n335 = To Unsigned Word Integer(number=w1406) -> (unsigned 16bit integer=w1403:u16)
                  n336 = To Unsigned Word Integer(number=w1405) -> (unsigned 16bit integer=w1402:u16)
                  n337 = To Unsigned Word Integer(number=w1401) -> (unsigned 16bit integer=w1399:u16)
                  n338 = To Unsigned Word Integer(number=w1400) -> (unsigned 16bit integer=w1397:u16)
                  n339 = Build Array(w1398, w1419, w1396, w1398, w1418, w1396, w1398, w1417, w1396, w1398, w1414, w1396, w1398, w1413, w1396, w1398, w1411, w1396, w1398, w1404, w1396, w1398, w1403, w1396, w1398, w1402, w1396, w1398, w1399, w1396, w1398, w1397, w1396) -> (w1408:u16[])
                  n340 = RT FIFO Write(0:w1410, 1:w1408, 3:w1409) -> ()  [unwired: 2 in, 4 out]
                }
                frame "saveSettings1" {
                  w1450 = u16 3 ("element")
                  w1449 = u16 0 ("element")
                  n341 = call "BRig_dataRT_stats__nTrial.vi"() -> ("output_nTrial"=w1446:i32)  [unwired: 11 in]
                  n342 = call "BRig_dataRT_stats__iTrial.vi"() -> ("output_iTrial"=w1445:i32)  [unwired: 11 in]
                  n343 = call "BRig_dataRT_stats__iBlock.vi"() -> ("output_iBlock"=w1444:i32)  [unwired: 11 in]
                  n344 = call "BRig_dataRT_stats__nReward_cur.vi"() -> ("output_nReward_cur"=w1443:i32)  [unwired: 11 in]
                  n345 = call "BRig_dataRT_stats__TpB_target.vi"() -> ("output_TpB_target"=w1442:i32)  [unwired: 11 in]
                  n346 = call "BRig_dataRT_stats__BUR_target.vi"() -> ("output_BUR_target"=w1441:i32)  [unwired: 11 in]
                  n347 = call "BRig_dataRT_stats__DAB_nReward_HighProb.vi"() -> ("output_DAB_nReward_HighProb"=w1440:i32)  [unwired: 11 in]
                  n348 = call "BRig_dataRT_stats__DAB_nReward_LowProb.vi"() -> ("output_DAB_nReward_LowProb"=w1439:i32)  [unwired: 11 in]
                  n349 = call "BRig_dataRT_stats__DAB_nTimeout.vi"() -> ("output_DAB_nTimeout"=w1438:i32)  [unwired: 11 in]
                  n350 = To Unsigned Word Integer(number=w1444) -> (unsigned 16bit integer=w1458:u16)
                  n351 = To Unsigned Word Integer(number=w1446) -> (unsigned 16bit integer=w1460:u16)
                  n352 = To Unsigned Word Integer(number=w1443) -> (unsigned 16bit integer=w1457:u16)
                  n353 = To Unsigned Word Integer(number=w1445) -> (unsigned 16bit integer=w1459:u16)
                  n354 = To Unsigned Word Integer(number=w1442) -> (unsigned 16bit integer=w1456:u16)
                  n355 = To Unsigned Word Integer(number=w1441) -> (unsigned 16bit integer=w1455:u16)
                  n356 = To Unsigned Word Integer(number=w1440) -> (unsigned 16bit integer=w1453:u16)
                  n357 = To Unsigned Word Integer(number=w1439) -> (unsigned 16bit integer=w1452:u16)
                  n358 = To Unsigned Word Integer(number=w1438) -> (unsigned 16bit integer=w1451:u16)
                  n359 = Build Array(w1450, w1460, w1449, w1450, w1459, w1449, w1450, w1458, w1449, w1450, w1457, w1449, w1450, w1456, w1449, w1450, w1455, w1449, w1450, w1453, w1449, w1450, w1452, w1449, w1450, w1451, w1449) -> (w1454:u16[])
                  n360 = RT FIFO Write(0:w1448, 1:w1454, 3:w1447) -> ()  [unwired: 2 in, 4 out]
                }
                frame "setSettings_Laser" {
                  n361 = call "BRig_dataExp_LED_baseline_Cue.vi"() -> ("output_LED_baseline_Cue"=w1482:i32)  [unwired: 11 in]
                  n362 = call "BRig_dataExp_LED_baseline_l1.vi"() -> ("output_LED_baseline_l1"=w1483:i32)  [unwired: 11 in]
                  n363 = call "BRig_dataExp_LED_baseline_l2.vi"() -> ("output_LED_baseline_l2"=w1481:i32)  [unwired: 11 in]
                  n364 = call "BRig_dataExp_I_anySelect.vi"() -> ("output_I_anySelect"=w1475:i32)  [unwired: 11 in]
                  n365 = call "BRig_dataExp_I_trialUntilReward.vi"() -> ("output_I_trialUntilReward"=w1474:i32)  [unwired: 11 in]
                  n366 = local read "FPGA_count2ms"() -> (w1492:dbl)
                  n367 = call "BRig_RT__Case_Exp__State_setLaserSettings.vi"("input_FPGA_count2ms"=w1492, "input_dataExp"=w1473, "input_dataLC"=w1493) -> ("output_LR_nTotal_l1"=w1491:u32, "output_LR_nTotal_l2"=w1490:u32, "output_LR_reward_nDelay_l1"=w1489:u32, "output_LR_wrong_nDelay_l1"=w1488:u32, "output_LR_reward_nDelay_l2"=w1487:u32, "output_LR_wrong_nDelay_l2"=w1486:u32)  [unwired: 11 in]
                  n368 = Index Array(array=w1473, index #1=w1482, index #2=w1483, index #3=w1481, index #4=w1475, index #5=w1474) -> (element #1=w1480:u16, element #2=w1479:u16, element #3=w1478:u16, element #4=w1477:u16, element #5=w1476:u16)
                  n369 = Not Equal To 0?(x=w1479) -> (x != 0?=w1471:bool)
                  n370 = Not Equal To 0?(x=w1477) -> (x != 0?=w1469:bool)
                  n371 = Not Equal To 0?(x=w1480) -> (x != 0?=w1472:bool)
                  n372 = Not Equal To 0?(x=w1478) -> (x != 0?=w1470:bool)
                  n373 = Not Equal To 0?(x=w1476) -> (x != 0?=w1468:bool)
                  n374 = xnode "Read/Write Control"("FPGA VI Reference In"=w1494, "error in"=w1495, "LR_reward_nTotal_l1"=w1491, "LR_wrong_nTotal_l1"=w1491, "LR_reward_nTotal_l2"=w1490, "LR_wrong_nTotal_l2"=w1490, "LR_reward_nDelay_l1"=w1489, "LR_wrong_nDelay_l1"=w1488, "LR_reward_nDelay_l2"=w1487, "LR_wrong_nDelay_l2"=w1486, "CueLed_Baseline"=w1472, "L1Led_Baseline"=w1471, "L2Led_Baseline"=w1470, "I_allReward"=w1469, "ignoreWrong"=w1468) -> ("error out"=→"error out":errorcluster)  [unwired: 1 out]
                }
                frame "initBlock" {
                  w1499 = u16 0 ("element")
                  w1502 = u16 3
                  w1519 = u16 0 ("BTPR_block")
                  n375 = local write "nRewards_cur"(u16 0 ("nRewards_cur")) -> ()
                  n376 = local write "BTPR_block"(w1519) -> ()
                  n377 = local write "T2R_block"(w1519) -> ()
                  n378 = call "BRig_RT__Case_Exp__State_initBlock__v10.vi"("input_dataCurrent"=w1539, "input_dataExp"=w1538, "input_dataBlock"=w1535, "input_dataTrial"=w1533) -> ("output_iSpout"=w1524:u16, "output_speaker_amp_R"=w1528:u16, "output_iBlock"=w1508:u16, "output_speaker_freq_R"=w1529:u8, "output_BUR_target"=w1509:u16, "output_speaker_amp_L"=w1530:u16, "output_TpB_target"=w1510:u16, "output_speaker_freq_L"=w1531:u8, "output_dataCurrent"=w1537:u16[], "output_dataBlock"=w1534:u16[][], "output_dataTrial"=w1532:u16[][])  [unwired: 5 in]
                  n379 = Type Cast(type=enum16{"Left", "Right"}."Left", x=w1524) -> (*(type *) &x=w1521:enum16{"Left", "Right"})
                  n380 = Not Equal To 0?(x=w1524) -> (x != 0?=w1520:bool)
                  n381 = call "BRig_dataRT_stats__TpB_target.vi"() -> ("output_TpB_target"=w1511:i32)  [unwired: 11 in]
                  n382 = call "BRig_dataRT_stats__BUR_target.vi"() -> ("output_BUR_target"=w1512:i32)  [unwired: 11 in]
                  n383 = call "BRig_dataRT_stats__iBlock.vi"() -> ("output_iBlock"=w1513:i32)  [unwired: 11 in]
                  n384 = call "BRig_dataRT_stats__T2R_cur.vi"() -> ("output_T2R_cur"=w1506:i32)  [unwired: 11 in]
                  n385 = call "BRig_dataRT_stats__BTPR_cur.vi"() -> ("output_BTPR_cur"=w1505:i32)  [unwired: 11 in]
                  n386 = call "BRig_dataRT_stats__nReward_cur.vi"() -> ("output_nReward_cur"=w1501:i32)  [unwired: 11 in]
                  n387 = local write "cSpout"(w1521) -> ()
                  n388 = xnode "Read/Write Control"("FPGA VI Reference In"=w1527, "error in"=w1526, "Left(F)_or_Right(T)"=w1520, "audioFreq_L_kHz"=w1531, "audioAmp_L"=w1530, "audioFreq_R_kHz"=w1529, "audioAmp_R"=w1528) -> ("error out"=w1525:errorcluster)  [unwired: 1 out]
                  n389 = To Unsigned Word Integer(number=w1506) -> (unsigned 16bit integer=w1504:u16)
                  n390 = To Unsigned Word Integer(number=w1501) -> (unsigned 16bit integer=w1500:u16)
                  n391 = To Unsigned Word Integer(number=w1511) -> (unsigned 16bit integer=w1518:u16)
                  n392 = To Unsigned Word Integer(number=w1512) -> (unsigned 16bit integer=w1515:u16)
                  n393 = To Unsigned Word Integer(number=w1513) -> (unsigned 16bit integer=w1514:u16)
                  n394 = To Unsigned Word Integer(number=w1505) -> (unsigned 16bit integer=w1503:u16)
                  n395 = local write "error out"(w1525) -> ()
                  n396 = local write "iBlock"(w1508) -> ()
                  n397 = local write "BUR_target"(w1509) -> ()
                  n398 = local write "TpB_target"(w1510) -> ()
                  n399 = Build Array(w1502, w1518, w1510, w1502, w1515, w1509, w1502, w1514, w1508, w1502, w1504, w1499, w1502, w1503, w1499, w1502, w1500, w1499) -> (w1507:u16[])
                  n400 = RT FIFO Write(0:w1516, 1:w1507, 3:w1517) -> ()  [unwired: 2 in, 4 out]
                }
                frame "initTrial" {
                  w1544 = u16 3
                  n401 = xnode "Read/Write Control"("FPGA VI Reference In"=w1563, "error in"=w1554, "SelectionState"=FALSE) -> ("error out"=w1562:errorcluster)  [unwired: 1 out]
                  n402 = call "BRig_RT__Case_Exp__State_initTrial__v10.vi"("input_dataCurrent"=w1553, "input_dataBlock"=w1557, "input_dataTrial"=w1560, "input_dataExp"=w1541) -> ("output_iTrial"=w1542:u16, "output_nTrial"=w1543:u16, "output_SolenoidReward"=w1559:bool, "output_dataCurrent"=w1552:u16[], "output_dataBlock"=w1556:u16[][], "output_dataTrial"=w1555:u16[][])  [unwired: 6 in]
                  n403 = call "BRig_dataRT_stats__nTrial.vi"() -> ("output_nTrial"=w1546:i32)  [unwired: 11 in]
                  n404 = call "BRig_dataRT_stats__iTrial.vi"() -> ("output_iTrial"=w1545:i32)  [unwired: 11 in]
                  n405 = local write "iTrial"(w1542) -> ()
                  n406 = local write "nTrial"(w1543) -> ()
                  n407 = local write "SolenoidReward"(w1559) -> ()
                  n408 = To Unsigned Word Integer(number=w1546) -> (unsigned 16bit integer=w1551:u16)
                  n409 = To Unsigned Word Integer(number=w1545) -> (unsigned 16bit integer=w1549:u16)
                  n410 = local write "error out"(w1562) -> ()
                  n411 = Build Array(w1544, w1551, w1543, w1544, w1549, w1542) -> (w1550:u16[])
                  n412 = RT FIFO Write(0:w1548, 1:w1550, 3:w1547) -> ()  [unwired: 2 in, 4 out]
                }
                frame "initTrial2" {
                  n413 = call "BRig_RT__Case_Exp__State_initTrial2__v10.vi"("input_dataCurrent"=w1566, "input_dataTrial"=w1584, "input_dataExp"=w1565, "input_dataBlock"=w1582, "input_dataLC"=w1583) -> ("output_L_Wrong_Laser_l2"=w1574:bool, "output_L_Wrong_Event_l2"=w1575:bool, "output_L_Power_l1"=w1573:dbl, "output_L_Reward_Laser_l2"=w1576:bool, "output_L_Power_l2"=w1572:dbl, "output_L_Reward_Event_l2"=w1577:bool, "output_dataCurrent"=w1568:u16[], "output_dataTrial"=w1567:u16[][], "output_L_Reward_Event_l1"=w1581:bool, "output_L_Reward_Laser_l1"=w1580:bool, "output_L_Wrong_Event_l1"=w1579:bool, "output_L_Wrong_Laser_l1"=w1578:bool)  [unwired: 3 in]
                  n414 = local write "L_Power_l1"(w1573) -> ()
                  n415 = call "myRIO__convert__Voltage_to_FPGAvalue.vi"("input_voltage"=w1573) -> ("output_PortC"=w1570:i16)  [unwired: 9 in, 1 out]
                  n416 = local write "L_Power_l2"(w1572) -> ()
                  n417 = call "myRIO__convert__Voltage_to_FPGAvalue.vi"("input_voltage"=w1572) -> ("output_PortC"=w1571:i16)  [unwired: 9 in, 1 out]
                  n418 = xnode "Read/Write Control"("FPGA VI Reference In"=w1588, "error in"=w1587, "AnaOut_0"=w1570, "AnaOut_1"=w1571, "LR_reward_Event_l1"=w1581, "LR_reward_Laser_l1"=w1580, "LR_wrong_Event_l1"=w1579, "LR_wrong_Laser_l1"=w1578, "LR_reward_Event_l2"=w1577, "LR_reward_Laser_l2"=w1576, "LR_wrong_Event_l2"=w1575, "LR_wrong_laser_l2"=w1574) -> ("error out"=w1585:errorcluster)  [unwired: 1 out]
                  n419 = local write "error out"(w1585) -> ()
                  n420 = call "BRig_arrTrig_init.vi"() -> ("output_arrTrig"=w1569:bool[])  [unwired: 11 in]
                }
                frame "initTrial4" {
                  # "Dual Armed Bandit?"
                  # "resetOccurrence?\ndataAnalog"
                  n421 = local read "FPGA_count2ms"() -> (w1597:dbl)
                  n422 = local read "lick_Rising(F)_or_Falling(T)"() -> (w1593:bool)
                  n423 = call "BRig_dataExp_I_anySelect.vi"() -> ("output_I_anySelect"=w1592:i32)  [unwired: 11 in]
                  n424 = Index Array(array=w1590, index=w1592) -> (element=w1591:u16)
                  n425 = local read "Recording"() -> (w1599:bool)
                  n426 = call "BRig_RT_comm_tcp_write_RTwrite__RunState_Trial_start.vi"("input_dataCurrent"=w1596) -> ("output_strCmd"=w1595:string)  [unwired: 10 in]
                  n427 = Not Equal To 0?(x=w1591) -> (x != 0?=w1589:bool)
                  n428 = call "BRig_RT__Case_Exp__State_initTrial4.vi"("input_Recording"=w1599, "input_FPGA_count2ms"=w1597, "input_dataTrial"=w1600) -> ("output_Solenoid_nTotal"=w1598:u32, "output_dataTrial"=w1594:u16[][])  [unwired: 7 in]
                  n429 = case shown="False" w1589 {
                    tunnel: w1605 -> [w1614 w1619]
                    tunnel: w1604 -> [w1613 w1618]
                    tunnel: [w1612 w1617] -> w1603
                    tunnel: w1599 -> [w1611 w1616]
                    tunnel: w1598 -> [w1610 _]
                    tunnel: w1593 -> [w1609 w1615]
                    frame False {
                      n430 = xnode "Read/Write Control"("FPGA VI Reference In"=w1614, "error in"=w1613, "Solenoid_nTotal_L"=w1610, "Solenoid_nTotal_R"=w1610, "A6_Act"=w1611, "Rising(F)_or_Falling(T)"=w1609) -> ("error out"=w1612:errorcluster)  [unwired: 1 out]
                    }
                    frame True {
                      n431 = xnode "Read/Write Control"("FPGA VI Reference In"=w1619, "error in"=w1618, "A6_Act"=w1616, "Rising(F)_or_Falling(T)"=w1615) -> ("error out"=w1617:errorcluster)  [unwired: 1 out]
                    }
                  }
                  n432 = local write "error out"(w1603) -> ()
                }
                frame "initTrial_LC_ENL1" {
                  n433 = call "BRig_RT__Case_Exp__State_initTrial__LC_ENL__v10.vi"("input_arrTrig"=w1628, "input_dataTrial"=w1627, "input_dataExp"=w1620, "input_dataLC"=w1625, "input_dataCurrent"=w1621) -> ("output_dataTrial"=w1623:u16[][], "output_dataCurrent"=w1624:u16[], "output_arrTrig"=w1622:bool[])  [unwired: 4 in]
                }
                frame "initTrial_LC_Cue1" {
                  n434 = call "BRig_RT__Case_Exp__State_initTrial__LC_Cue__v10.vi"("input_arrTrig"=w1634, "input_dataTrial"=w1636, "input_dataExp"=w1630, "input_dataLC"=w1632, "input_dataCurrent"=w1631) -> ("output_dataTrial"=w1635:u16[][], "output_dataCurrent"=w1638:u16[], "output_arrTrig"=w1633:bool[])  [unwired: 4 in]
                }
                frame "initTrial_LC_Sel" {
                  n435 = call "BRig_RT__Case_Exp__State_initTrial__LC_Select__v10.vi"("input_arrTrig"=w1642, "input_dataTrial"=w1644, "input_dataExp"=w1640, "input_dataLC"=w1646, "input_dataCurrent"=w1648) -> ("output_dataTrial"=w1643:u16[][], "output_dataCurrent"=w1647:u16[], "output_arrTrig"=w1641:bool[])  [unwired: 4 in]
                  n436 = xnode "Read/Write Control"("FPGA VI Reference In"=w1651, "error in"=w1650, "A6_Act"=FALSE) -> ("error out"=w1652:errorcluster)  [unwired: 1 out]
                  n437 = local write "error out"(w1652) -> ()
                }
                frame "ENL1_pre" {
                  n438 = call "BRig_RT__Case_Exp__State_ENLPre__v4.vi"("input_arrTrig"=w1656, "input_ENL2"=FALSE, "input_I_lick"=w1662, "input_dataExp"=w1654, "input_dataTrial"=w1659, "input_dataCurrent"=w1660) -> ("output_arrTrig"=w1655:bool[], "output_dataTrial"=w1658:u16[][], "output_dataCurrent"=w1663:u16[], "output_state"=w1661:T2)  [unwired: 2 in]
                }
                frame "ENL2_pre" {
                  n439 = call "BRig_RT__Case_Exp__State_ENLPre__v4.vi"("input_arrTrig"=w1667, "input_ENL2"=TRUE, "input_I_lick"=w1674, "input_dataExp"=w1668, "input_dataTrial"=w1671, "input_dataCurrent"=w1672) -> ("output_arrTrig"=w1666:bool[], "output_dataTrial"=w1670:u16[][], "output_dataCurrent"=w1675:u16[], "output_state"=w1673:T2)  [unwired: 2 in]
                }
                frame "ENL1" {
                  n440 = call "BRig_RT__Case_Exp__State_ENL__v3.vi"("input_dataCurrent"=w1690, "input_dataTrial"=w1680, "input_ENL2"=FALSE, "input_arrTrig"=w1684, "input_state"=w1683, "I_lick"=w1682) -> ("output_l2_laserOn"=w1685:bool, "output_l2_laserEvent"=w1686:bool, "output_l1_laserOn"=w1687:bool, "output_state"=w1681:T2, "output_l1_laserEvent"=w1688:bool, "output_dataCurrent"=w1689:u16[], "output_dataTrial"=w1679:u16[][])  [unwired: 7 in]
                }
                frame "ENL2" {
                  n441 = call "BRig_RT__Case_Exp__State_ENL__v3.vi"("input_dataCurrent"=w1706, "input_dataTrial"=w1696, "input_ENL2"=TRUE, "input_arrTrig"=w1700, "input_state"=w1699, "I_lick"=w1698) -> ("output_l2_laserOn"=w1701:bool, "output_l2_laserEvent"=w1702:bool, "output_l1_laserOn"=w1703:bool, "output_state"=w1697:T2, "output_l1_laserEvent"=w1704:bool, "output_dataCurrent"=w1705:u16[], "output_dataTrial"=w1695:u16[][])  [unwired: 7 in]
                }
                frame "ENL1Penalty_pre" {
                  n442 = call "BRig_dataCurrent_c_generic.vi"() -> ("output_count_generic"=w1722:i32)  [unwired: 11 in]
                  n443 = call "BRig_dataCurrent_T_generic.vi"() -> ("output_T_generic"=w1720:i32)  [unwired: 11 in]
                  n444 = call "BRig_dataExp_T_ENLPenalty.vi"() -> ("output_ENL_penalty"=w1715:i32)  [unwired: 11 in]
                  n445 = Index Array(array=w1716, index=w1715) -> (element=w1719:u16)
                  n446 = Replace Array Subset(array=w1717, new element #1=u16 0 ("new element/subarray"), index #1=w1722, new element #2=w1719, index #2=w1720) -> (w1718:u16[])
                }
                frame "ENL1Penalty" {
                  n447 = call "BRig_RT__Case_Exp__generic__incrementCountTilThreshold.vi"("input_dataCurrent"=w1725) -> ("output_dataCurrent"=w1724:u16[], "output_underThreshold"=w1723:bool)  [unwired: 9 in]
                  n448 = Select(t=w1728, s=w1723, f=myRIO_BRig_RT__Case_Exp_stateList."ENL1_pre" ("Enum")) -> (s? t:f=w1726:T2)
                }
                frame "Cue1_pre" {
                  n449 = call "BRig_RT__Case_Exp__State_CuePre__v3.vi"("input_dataCurrent"=w1743, "input_dataTrial"=w1739, "input_Cue2"=FALSE ("input_ENL2"), "input_I_lick"=w1742, "input_dataExp"=w1740, "input_arrTrig"=w1736) -> ("output_state"=w1741:T2, "output_arrTrig"=w1735:bool[], "output_dataCurrent"=w1737:u16[], "output_dataTrial"=w1738:u16[][])  [unwired: 10 in]
                }
                frame "Cue2_pre" {
                  n450 = call "BRig_RT__Case_Exp__State_CuePre__v3.vi"("input_dataCurrent"=w1755, "input_dataTrial"=w1751, "input_Cue2"=TRUE ("input_ENL2"), "input_I_lick"=w1754, "input_dataExp"=w1752, "input_arrTrig"=w1748) -> ("output_state"=w1753:T2, "output_arrTrig"=w1747:bool[], "output_dataCurrent"=w1749:u16[], "output_dataTrial"=w1750:u16[][])  [unwired: 10 in]
                }
                frame "Cue1" {
                  n451 = call "BRig_RT__Case_Exp__State_Cue__v3.vi"("input_dataCurrent"=w1777, "input_dataTrial"=w1765, "input_dataExp"=w1759, "input_Cue2"=FALSE, "input_arrTrig"=w1773, "input_state"=w1775, "I_lick"=w1776) -> ("output_l2_laserOn"=w1769:bool, "output_l2_laserEvent"=w1770:bool, "output_SelectionState"=w1768:bool, "output_l1_laserOn"=w1771:bool, "output_state"=w1774:T2, "output_l1_laserEvent"=w1772:bool, "output_dataCurrent"=w1760:u16[], "output_dataTrial"=w1764:u16[][], "output_CueLed"=w1763:bool, "output_Audio_L"=w1762:bool, "output_Audio_R"=w1761:bool)  [unwired: 2 in]
                  n452 = case shown="True" w1768 {
                    selector: w1768 -> [_ w1783]
                    tunnel: w1767 -> [_ w1782]
                    tunnel: w1766 -> [_ w1781]
                    frame False {
                    }
                    frame True {
                      n453 = xnode "Read/Write Control"("FPGA VI Reference In"=w1781, "error in"=w1782, "SelectionState"=w1783) -> ("error out"=w1784:errorcluster)  [unwired: 1 out]
                      n454 = local write "error out"(w1784) -> ()
                    }
                  }
                }
                frame "Cue2" {
                  n455 = call "BRig_RT__Case_Exp__State_Cue__v3.vi"("input_dataCurrent"=w1804, "input_dataTrial"=w1792, "input_dataExp"=w1786, "input_Cue2"=TRUE, "input_arrTrig"=w1800, "input_state"=w1802, "I_lick"=w1803) -> ("output_l2_laserOn"=w1796:bool, "output_l2_laserEvent"=w1797:bool, "output_SelectionState"=w1795:bool, "output_l1_laserOn"=w1798:bool, "output_state"=w1801:T2, "output_l1_laserEvent"=w1799:bool, "output_dataCurrent"=w1787:u16[], "output_dataTrial"=w1791:u16[][], "output_CueLed"=w1790:bool, "output_Audio_L"=w1789:bool, "output_Audio_R"=w1788:bool)  [unwired: 2 in]
                  n456 = case shown="True" w1795 {
                    selector: w1795 -> [_ w1810]
                    tunnel: w1794 -> [_ w1809]
                    tunnel: w1793 -> [_ w1808]
                    frame False {
                    }
                    frame True {
                      n457 = xnode "Read/Write Control"("FPGA VI Reference In"=w1808, "error in"=w1809, "SelectionState"=w1810) -> ("error out"=w1811:errorcluster)  [unwired: 1 out]
                      n458 = local write "error out"(w1811) -> ()
                    }
                  }
                }
                frame "Cue1Penalty_pre" {
                  n459 = call "BRig_dataCurrent_c_generic.vi"() -> ("output_count_generic"=w1824:i32)  [unwired: 11 in]
                  n460 = call "BRig_dataCurrent_T_generic.vi"() -> ("output_T_generic"=w1822:i32)  [unwired: 11 in]
                  n461 = call "BRig_dataExp_T_CuePenalty.vi"() -> ("output_T_CuePenalty"=w1813:i32)  [unwired: 11 in]
                  n462 = Index Array(array=w1814, index=w1813) -> (element=w1812:u16)
                  n463 = Replace Array Subset(array=w1821, new element #1=u16 0 ("new element/subarray"), index #1=w1824, new element #2=w1812, index #2=w1822) -> (w1820:u16[])
                }
                frame "Cue1Penalty" {
                  n464 = call "BRig_RT__Case_Exp__generic__incrementCountTilThreshold.vi"("input_dataCurrent"=w1827) -> ("output_dataCurrent"=w1826:u16[], "output_underThreshold"=w1825:bool)  [unwired: 9 in]
                  n465 = Select(t=w1828, s=w1825, f=myRIO_BRig_RT__Case_Exp_stateList."ENL1_pre" ("Enum")) -> (s? t:f=w1829:T2)
                }
                frame "Selection_pre" {
                  n466 = xnode "Read/Write Control"("FPGA VI Reference In"=w1850, "error in"=w1851) -> ("error out"=w1849:errorcluster, "SelectReward"=w1846:bool, "SelectWrong"=w1847:bool)  [unwired: 1 out]
                  n467 = call "BRig_RT__Case_Exp__State_SelectPre.vi"("input_dataCurrent"=w1848, "input_SelectWrong"=w1847, "input_SelectReward"=w1846, "input_dataExp"=w1836, "input_LickL"=w1838, "input_LickR"=w1837, "input_arrTrig"=w1839) -> ("output_state"=w1845:T2, "output_dataCurrent"=w1844:u16[], "output_l1_laserEvent"=w1843:bool, "output_l1_laserOn"=w1842:bool, "output_l2_laserOn"=w1840:bool, "output_l2_laserEvent"=w1841:bool)  [unwired: 3 in]
                  n468 = local write "error out"(w1849) -> ()
                }
                frame "Selection" {
                  n469 = xnode "Read/Write Control"("FPGA VI Reference In"=w1875, "error in"=w1874) -> ("error out"=w1873:errorcluster, "SelectReward"=w1870:bool, "SelectWrong"=w1871:bool)  [unwired: 1 out]
                  n470 = call "BRig_RT__Case_Exp__State_Selection.vi"("input_state"=w1872, "input_dataCurrent"=w1865, "input_dataTrial"=w1856, "input_dataExp"=w1864, "input_arrTrig"=w1863, "input_FPGA_SelectWrong"=w1871, "input_FPGA_SelectReward"=w1870, "input_LickR"=w1869, "input_LickL"=w1868) -> ("output_LC_Laser_l2"=w1859:bool, "output_LC_Event_l2"=w1860:bool, "output_LC_Laser_l1"=w1861:bool, "output_LC_Event_l1"=w1862:bool, "output_state"=w1867:T2, "output_dataCurrent"=w1866:u16[], "output_dataTrial"=w1855:u16[][], "output_anySelect_L"=w1857:bool, "output_anySelect_R"=w1858:bool)  [unwired: 2 in]
                  n471 = local write "allReward_L"(w1857) -> ()
                  n472 = local write "allReward_R"(w1858) -> ()
                  n473 = local write "error out"(w1873) -> ()
                }
                frame "SelectReward_pre" {
                  # "Dual Armed\nBandit?"
                  n474 = call "BRig_dataExp_I_anySelect.vi"() -> ("output_I_anySelect"=w1890:i32)  [unwired: 11 in]
                  n475 = Index Array(array=w1888, index=w1890) -> (element=w1889:u16)
                  n476 = call "BRig_RT__Case_Exp__State_RewardPre__v10.vi"("input_dataCurrent"=w1906, "input_dataExp"=w1888, "input_dataBlock"=w1905, "input_dataTrial"=w1900) -> ("output_T_Reward"=w1896:u16, "output_c_nReward_total_R"=w1881:u16, "output_c_nReward_total_L"=w1880:u16, "output_dataCurrent"=w1903:u16[], "output_DAB_L=L"=w1878:bool, "output_DAB_R=HighPorb"=w1879:bool, "output_dataBlock"=w1904:u16[][], "output_c_nReward_total"=w1883:u16, "output_nReward"=w1882:u16, "output_dataTrial"=w1899:u16[][])  [unwired: 2 in]
                  n477 = local read "FPGA_count2ms"() -> (w1895:dbl)
                  n478 = Not Equal To 0?(x=w1889) -> (x != 0?=w1887:bool)
                  n479 = case shown="True" w1887 {
                    tunnel: [w1913 w1935] -> w1884
                    tunnel: w1883 -> [w1912 w1932]
                    tunnel: w1882 -> [w1911 w1931]
                    tunnel: w1881 -> [w1910 w1934]
                    tunnel: w1880 -> [w1909 w1933]
                    tunnel: w1879 -> [_ w1925]
                    tunnel: w1878 -> [_ w1926]
                    frame False {
                      w1917 = u16 3
                      n480 = call "BRig_dataRT_stats__nReward_left.vi"() -> ("output_nReward_left"=w1914:i32)  [unwired: 11 in]
                      n481 = call "BRig_dataRT_stats__nReward_right.vi"() -> ("output_nReward_right"=w1915:i32)  [unwired: 11 in]
                      n482 = call "BRig_dataRT_stats__nReward_cur.vi"() -> ("output_nReward_cur"=w1916:i32)  [unwired: 11 in]
                      n483 = call "BRig_dataRT_stats__nReward.vi"() -> ("output_nReward"=w1919:i32)  [unwired: 11 in]
                      n484 = To Unsigned Word Integer(number=w1914) -> (unsigned 16bit integer=w1922:u16)
                      n485 = To Unsigned Word Integer(number=w1915) -> (unsigned 16bit integer=w1921:u16)
                      n486 = To Unsigned Word Integer(number=w1916) -> (unsigned 16bit integer=w1920:u16)
                      n487 = To Unsigned Word Integer(number=w1919) -> (unsigned 16bit integer=w1918:u16)
                      n488 = local write "nRewards_Right"(w1910) -> ()
                      n489 = local write "nRewards_Left"(w1909) -> ()
                      n490 = local write "nRewards_cur"(w1911) -> ()
                      n491 = local write "nRewards_total"(w1912) -> ()
                      n492 = Build Array(w1917, w1922, w1909, w1917, w1921, w1910, w1917, w1920, w1911, w1917, w1918, w1912) -> (w1913:u16[])
                    }
                    frame True {
                      w1937 = u16 3
                      n493 = call "BRig_dataRT_stats__nReward_left.vi"() -> ("output_nReward_left"=w1930:i32)  [unwired: 11 in]
                      n494 = call "BRig_dataRT_stats__nReward_right.vi"() -> ("output_nReward_right"=w1929:i32)  [unwired: 11 in]
                      n495 = call "BRig_dataRT_stats__DAB_nReward_HighProb.vi"() -> ("output_DAB_nReward_HighProb"=w1928:i32)  [unwired: 11 in]
                      n496 = call "BRig_dataRT_stats__DAB_nReward_LowProb.vi"() -> ("output_DAB_nReward_LowProb"=w1927:i32)  [unwired: 11 in]
                      n497 = call "BRig_dataRT_stats__nReward_cur.vi"() -> ("output_nReward_cur"=w1936:i32)  [unwired: 11 in]
                      n498 = call "BRig_dataRT_stats__nReward.vi"() -> ("output_nReward"=w1939:i32)  [unwired: 11 in]
                      n499 = Select(t=w1930, s=w1926, f=w1929) -> (s? t:f=w1923:i32)
                      n500 = Select(t=w1928, s=w1925, f=w1927) -> (s? t:f=w1924:i32)
                      n501 = To Unsigned Word Integer(number=w1923) -> (unsigned 16bit integer=w1942:u16)
                      n502 = To Unsigned Word Integer(number=w1924) -> (unsigned 16bit integer=w1941:u16)
                      n503 = To Unsigned Word Integer(number=w1936) -> (unsigned 16bit integer=w1940:u16)
                      n504 = To Unsigned Word Integer(number=w1939) -> (unsigned 16bit integer=w1938:u16)
                      n505 = local write "nRewards_cur"(w1931) -> ()
                      n506 = local write "nRewards_total"(w1932) -> ()
                      n507 = Build Array(w1937, w1942, w1933, w1937, w1941, w1934, w1937, w1940, w1931, w1937, w1938, w1932) -> (w1935:u16[])
                    }
                  }
                  n508 = To Double Precision Float(number=w1896) -> (double precision float=w1894:dbl)
                  n509 = Multiply(x=w1895, y=w1894) -> (x*y=w1892:dbl)
                  n510 = Round Toward +Infinity(x=w1892) -> (ceil(x): smallest int >= x=w1893:dbl)
                  n511 = To Unsigned Long Integer(number=w1893) -> (unsigned 32bit integer=w1891:u32)
                  n512 = RT FIFO Write(0:w1886, 1:w1884, 3:w1885) -> ()  [unwired: 2 in, 4 out]
                  n513 = call "BRig_RT_comm_tcp_write_RTwrite__RunState_Trial_selResult__v2.vi"("input_dataTrial"=w1899, "iReward_or_iError"=TRUE, "input_dataCurrent"=w1903) -> ("output_strCmd"=w1901:string)  [unwired: 8 in]
                  n514 = xnode "Read/Write Control"("FPGA VI Reference In"=w1898, "error in"=w1897, "Solenoid_nTotal_L"=w1891, "Solenoid_nTotal_R"=w1891) -> ()  [unwired: 2 out]
                }
                frame "SelectReward" {
                  n515 = call "BRig_dataCurrent_c_generic.vi"() -> ("output_count_generic"=w1949:i32)  [unwired: 11 in]
                  n516 = call "BRig_RT__Case_Exp__State_Reward.vi"("input_dataCurrent"=w1950, "input_state"=w1954, "input_dataExp"=w1952) -> ("output_state"=w1953:T2, "output_dataCurrent"=w1955:u16[], "output__L"=w1947:bool, "output__R"=w1946:bool)  [unwired: 9 in]
                  n517 = Index Array(array=w1950, index=w1949) -> (element=w1948:u16)
                  n518 = Equal To 0?(x=w1948) -> (x = 0?=w1945:bool)
                  n519 = And(x=w1947, y=w1945) -> (x .and. y?=w1944:bool)
                  n520 = And(x=w1946, y=w1945) -> (x .and. y?=w1943:bool)
                }
                frame "SelectRewardPost_pre" {
                  n521 = call "BRig_dataExp_T_RewardPost.vi"() -> ("output_T_RewardPost"=w1959:i32)  [unwired: 11 in]
                  n522 = call "BRig_dataCurrent_c_generic.vi"() -> ("output_count_generic"=w1965:i32)  [unwired: 11 in]
                  n523 = call "BRig_dataCurrent_T_generic.vi"() -> ("output_T_generic"=w1964:i32)  [unwired: 11 in]
                  n524 = Index Array(array=w1960, index=w1959) -> (element=w1958:u16)
                  n525 = Replace Array Subset(array=w1962, new element #1=u16 0 ("new element/subarray"), index #1=w1965, new element #2=w1958, index #2=w1964) -> (w1961:u16[])
                }
                frame "SelectRewardPost" {
                  n526 = call "BRig_RT__Case_Exp__generic__incrementCountTilThreshold.vi"("input_dataCurrent"=w1972) -> ("output_dataCurrent"=w1970:u16[], "output_underThreshold"=w1971:bool)  [unwired: 9 in]
                  n527 = Select(t=w1974, s=w1971, f=myRIO_BRig_RT__Case_Exp_stateList."endTrial1" ("Enum")) -> (s? t:f=w1973:T2)
                }
                frame "SelectWrong_pre" {
                  # "Dual Armed\nBandit?"
                  n528 = call "BRig_dataExp_I_anySelect.vi"() -> ("output_I_anySelect"=w1983:i32)  [unwired: 11 in]
                  n529 = Index Array(array=w1984, index=w1983) -> (element=w1985:u16)
                  n530 = call "BRig_RT__Case_Exp__State_WrongOrTimeout_Pre__v10.vi"("input_dataCurrent"=w2001, "input_WorTO"=FALSE, "input_dataBlock"=w1999, "input_dataTrial"=w1997, "input_dataExp"=w1984) -> ("output_T2R"=w1980:bool, "output_T2R_or_BTPR"=w1981:u16, "output_dataCurrent"=w1995:u16[], "output_dataBlock"=w1998:u16[][], "output_dataTrial"=w1994:u16[][], "output_BTPRavg"=w1990:dbl, "output_T2Ravg"=w1991:dbl, "output_R(F)_or_L(T)"=w1992:bool, "output_haveNewAvg"=w1993:bool)  [unwired: 1 in, 1 out]
                  n531 = Not Equal To 0?(x=w1985) -> (x != 0?=w1982:bool)
                  n532 = case shown="False" w1982 {
                    tunnel: w1993 -> [_ w2018]
                    tunnel: w1992 -> [_ w2017]
                    tunnel: w1991 -> [_ w2016]
                    tunnel: w1990 -> [_ w2015]
                    tunnel: [w2007 w2013] -> w1988
                    tunnel: w1981 -> [w2005 w2009]
                    tunnel: w1980 -> [_ w2011]
                    frame True {
                      n533 = call "BRig_dataRT_stats__DAB_nTimeout.vi"() -> ("output_DAB_nTimeout"=w2004:i32)  [unwired: 11 in]
                      n534 = To Unsigned Word Integer(number=w2004) -> (unsigned 16bit integer=w2006:u16)
                      n535 = Build Array(u16 3, w2006, w2005) -> (w2007:u16[])
                    }
                    frame False {
                      n536 = case shown="False" w2011 {
                        tunnel: w2009 -> [w2020 w2022]
                        tunnel: [w2019 w2021] -> w2012
                        frame False {
                          n537 = call "BRig_dataRT_stats__BTPR_cur.vi"() -> ("output_BTPR_cur"=w2019:i32)  [unwired: 11 in]
                          n538 = local write "BTPR_block"(w2020) -> ()
                        }
                        frame True {
                          n539 = call "BRig_dataRT_stats__T2R_cur.vi"() -> ("output_T2R_cur"=w2021:i32)  [unwired: 11 in]
                          n540 = local write "T2R_block"(w2022) -> ()
                        }
                      }
                      n541 = To Unsigned Word Integer(number=w2012) -> (unsigned 16bit integer=w2010:u16)
                      n542 = case shown="True" w2018 {
                        tunnel: w2017 -> [_ w2042]
                        tunnel: w2016 -> [_ w2032]
                        tunnel: w2015 -> [_ w2028]
                        tunnel: u16 3 -> [w2026 w2035]
                        tunnel: w2010 -> [w2025 w2031]
                        tunnel: w2009 -> [w2024 w2034]
                        tunnel: [w2023 w2033] -> w2013
                        frame False {
                          n543 = Build Array(w2026, w2025, w2024) -> (w2023:u16[])
                        }
                        frame True {
                          w2027 = 100.0 ("y")
                          n544 = case shown="False" w2042 {
                            tunnel: w2032 -> [w2045 w2050]
                            tunnel: w2028 -> [w2046 w2049]
                            tunnel: [w2043 w2048] -> w2041
                            tunnel: [w2044 w2047] -> w2040
                            frame False {
                              n545 = local write "BTPR_avg_R"(w2046) -> ()
                              n546 = call "BRig_dataRT_stats__BTPR_avg_R.vi"() -> ("output_BTPR_avg_R__x100"=w2044:i32)  [unwired: 11 in]
                              n547 = local write "T2R_avg_R"(w2045) -> ()
                              n548 = call "BRig_dataRT_stats__T2R_avg_R.vi"() -> ("output_T2R_avg_R__x100"=w2043:i32)  [unwired: 11 in]
                            }
                            frame True {
                              n549 = call "BRig_dataRT_stats__BTPR_avg_L.vi"() -> ("output_BTPR_avg_L__x100"=w2047:i32)  [unwired: 11 in]
                              n550 = local write "BTPR_avg_L"(w2049) -> ()
                              n551 = local write "T2R_avg_L"(w2050) -> ()
                              n552 = call "BRig_dataRT_stats__T2R_avg_L.vi"() -> ("output_T2R_avg_L__x100"=w2048:i32)  [unwired: 11 in]
                            }
                          }
                          n553 = Multiply(x=w2032, y=w2027) -> (x*y=w2029:dbl)
                          n554 = Multiply(x=w2028, y=w2027) -> (x*y=w2030:dbl)
                          n555 = To Unsigned Word Integer(number=w2029) -> (unsigned 16bit integer=w2036:u16)
                          n556 = To Unsigned Word Integer(number=w2030) -> (unsigned 16bit integer=w2037:u16)
                          n557 = To Unsigned Word Integer(number=w2040) -> (unsigned 16bit integer=w2038:u16)
                          n558 = To Unsigned Word Integer(number=w2041) -> (unsigned 16bit integer=w2039:u16)
                          n559 = Build Array(w2035, w2039, w2036, w2035, w2038, w2037, w2035, w2031, w2034) -> (w2033:u16[])
                        }
                      }
                    }
                  }
                  n560 = RT FIFO Write(0:w1989, 1:w1988, 3:w1987) -> ()  [unwired: 2 in, 4 out]
                  n561 = call "BRig_RT_comm_tcp_write_RTwrite__RunState_Trial_selResult__v2.vi"("input_dataTrial"=w1994, "iReward_or_iError"=FALSE, "input_dataCurrent"=w1995) -> ("output_strCmd"=w1986:string)  [unwired: 8 in]
                }
                frame "SelectTimeout_pre" {
                  # "Dual Armed\nBandit?"
                  n562 = call "BRig_dataExp_I_anySelect.vi"() -> ("output_I_anySelect"=w2054:i32)  [unwired: 11 in]
                  n563 = Index Array(array=w2055, index=w2054) -> (element=w2056:u16)
                  n564 = call "BRig_RT__Case_Exp__State_WrongOrTimeout_Pre__v10.vi"("input_dataCurrent"=w2072, "input_WorTO"=TRUE, "input_dataBlock"=w2070, "input_dataTrial"=w2068, "input_dataExp"=w2055) -> ("output_T2R"=w2051:bool, "output_T2R_or_BTPR"=w2052:u16, "output_dataCurrent"=w2066:u16[], "output_dataBlock"=w2069:u16[][], "output_dataTrial"=w2065:u16[][], "output_BTPRavg"=w2061:dbl, "output_T2Ravg"=w2062:dbl, "output_R(F)_or_L(T)"=w2063:bool, "output_haveNewAvg"=w2064:bool)  [unwired: 1 in, 1 out]
                  n565 = Not Equal To 0?(x=w2056) -> (x != 0?=w2053:bool)
                  n566 = case shown="False" w2053 {
                    tunnel: w2064 -> [_ w2089]
                    tunnel: w2063 -> [_ w2088]
                    tunnel: w2062 -> [_ w2087]
                    tunnel: w2061 -> [_ w2086]
                    tunnel: [w2078 w2084] -> w2059
                    tunnel: w2052 -> [w2076 w2080]
                    tunnel: w2051 -> [_ w2082]
                    frame True {
                      n567 = call "BRig_dataRT_stats__DAB_nTimeout.vi"() -> ("output_DAB_nTimeout"=w2075:i32)  [unwired: 11 in]
                      n568 = To Unsigned Word Integer(number=w2075) -> (unsigned 16bit integer=w2077:u16)
                      n569 = Build Array(u16 3, w2077, w2076) -> (w2078:u16[])
                    }
                    frame False {
                      n570 = case shown="False" w2082 {
                        tunnel: w2080 -> [w2091 w2093]
                        tunnel: [w2090 w2092] -> w2083
                        frame False {
                          n571 = call "BRig_dataRT_stats__BTPR_cur.vi"() -> ("output_BTPR_cur"=w2090:i32)  [unwired: 11 in]
                          n572 = local write "BTPR_block"(w2091) -> ()
                        }
                        frame True {
                          n573 = call "BRig_dataRT_stats__T2R_cur.vi"() -> ("output_T2R_cur"=w2092:i32)  [unwired: 11 in]
                          n574 = local write "T2R_block"(w2093) -> ()
                        }
                      }
                      n575 = To Unsigned Word Integer(number=w2083) -> (unsigned 16bit integer=w2081:u16)
                      n576 = case shown="True" w2089 {
                        tunnel: w2088 -> [_ w2113]
                        tunnel: w2087 -> [_ w2103]
                        tunnel: w2086 -> [_ w2099]
                        tunnel: u16 3 -> [w2097 w2106]
                        tunnel: w2081 -> [w2096 w2102]
                        tunnel: w2080 -> [w2095 w2105]
                        tunnel: [w2094 w2104] -> w2084
                        frame False {
                          n577 = Build Array(w2097, w2096, w2095) -> (w2094:u16[])
                        }
                        frame True {
                          w2098 = 100.0 ("y")
                          n578 = case shown="False" w2113 {
                            tunnel: w2103 -> [w2116 w2121]
                            tunnel: w2099 -> [w2117 w2120]
                            tunnel: [w2114 w2119] -> w2112
                            tunnel: [w2115 w2118] -> w2111
                            frame False {
                              n579 = local write "BTPR_avg_R"(w2117) -> ()
                              n580 = call "BRig_dataRT_stats__BTPR_avg_R.vi"() -> ("output_BTPR_avg_R__x100"=w2115:i32)  [unwired: 11 in]
                              n581 = local write "T2R_avg_R"(w2116) -> ()
                              n582 = call "BRig_dataRT_stats__T2R_avg_R.vi"() -> ("output_T2R_avg_R__x100"=w2114:i32)  [unwired: 11 in]
                            }
                            frame True {
                              n583 = call "BRig_dataRT_stats__BTPR_avg_L.vi"() -> ("output_BTPR_avg_L__x100"=w2118:i32)  [unwired: 11 in]
                              n584 = local write "BTPR_avg_L"(w2120) -> ()
                              n585 = local write "T2R_avg_L"(w2121) -> ()
                              n586 = call "BRig_dataRT_stats__T2R_avg_L.vi"() -> ("output_T2R_avg_L__x100"=w2119:i32)  [unwired: 11 in]
                            }
                          }
                          n587 = Multiply(x=w2103, y=w2098) -> (x*y=w2100:dbl)
                          n588 = Multiply(x=w2099, y=w2098) -> (x*y=w2101:dbl)
                          n589 = To Unsigned Word Integer(number=w2100) -> (unsigned 16bit integer=w2107:u16)
                          n590 = To Unsigned Word Integer(number=w2101) -> (unsigned 16bit integer=w2108:u16)
                          n591 = To Unsigned Word Integer(number=w2111) -> (unsigned 16bit integer=w2109:u16)
                          n592 = To Unsigned Word Integer(number=w2112) -> (unsigned 16bit integer=w2110:u16)
                          n593 = Build Array(w2106, w2110, w2107, w2106, w2109, w2108, w2106, w2102, w2105) -> (w2104:u16[])
                        }
                      }
                    }
                  }
                  n594 = RT FIFO Write(0:w2060, 1:w2059, 3:w2058) -> ()  [unwired: 2 in, 4 out]
                  n595 = call "BRig_RT_comm_tcp_write_RTwrite__RunState_Trial_selResult__v2.vi"("input_dataTrial"=w2065, "iReward_or_iError"=FALSE, "input_dataCurrent"=w2066) -> ("output_strCmd"=w2057:string)  [unwired: 8 in]
                }
                frame "SelectWrong" {
                  n596 = call "BRig_RT__Case_Exp__generic__incrementCountTilThreshold.vi"("input_dataCurrent"=w2124) -> ("output_dataCurrent"=w2122:u16[], "output_underThreshold"=w2123:bool)  [unwired: 9 in]
                  n597 = Select(t=w2126, s=w2123, f=myRIO_BRig_RT__Case_Exp_stateList."endTrial1" ("Enum")) -> (s? t:f=w2125:T2)
                }
                frame "SelectTimeout" {
                  n598 = call "BRig_RT__Case_Exp__generic__incrementCountTilThreshold.vi"("input_dataCurrent"=w2134) -> ("output_dataCurrent"=w2133:u16[], "output_underThreshold"=w2132:bool)  [unwired: 9 in]
                  n599 = Select(t=w2136, s=w2132, f=myRIO_BRig_RT__Case_Exp_stateList."endTrial1" ("Enum")) -> (s? t:f=w2135:T2)
                }
                frame "endTrial1" {
                  n600 = call "BRig_RT_comm_tcp_write_RTwrite__RunState_Trial_end.vi"("input_dataCurrent"=w2150) -> ("output_strCmd"=w2149:string)  [unwired: 10 in]
                  n601 = call "BRig_RT__Case_Exp__State_endTrial__v10.vi"("input_dataBlock"=w2146, "input_timeStamp_start"=w2151, "input_dataTrial"=w2158, "input_dataCurrent"=w2150) -> ("output_BTPRavg"=w2143:dbl, "output_T2Ravg"=w2144:dbl, "output_dataTrial"=w2157:u16[][], "output_dataCurrent"=w2152:u16[], "output_R(F)_or_L(T)"=w2145:bool, "output_runTime"=→"T_ExpRun_min":dbl)  [unwired: 2 in]
                  n602 = xnode "Read/Write Control"("FPGA VI Reference In"=w2154, "error in"=w2153, "SelectionState"=FALSE) -> ("error out"=w2155:errorcluster)  [unwired: 1 out]
                  n603 = case shown="False" w2145 {
                    tunnel: w2144 -> [w2160 w2163]
                    tunnel: w2143 -> [w2161 w2162]
                    frame False {
                      n604 = local write "BTPR_avg_R"(w2161) -> ()
                      n605 = local write "T2R_avg_R"(w2160) -> ()
                    }
                    frame True {
                      n606 = local write "BTPR_avg_L"(w2162) -> ()
                      n607 = local write "T2R_avg_L"(w2163) -> ()
                    }
                  }
                  n608 = local write "error out"(w2155) -> ()
                }
                frame "endTrial2" {
                  n609 = case shown="True" w2173 {
                    tunnel: [w2181 _] -> w2174
                    tunnel: [w2180 w2183] -> w2169
                    tunnel: w2168 -> [w2178 w2191]
                    tunnel: w2167 -> [w2179 w2189]
                    tunnel: [w2179 w2188] -> w2166
                    tunnel: [w2178 w2190] -> w2165
                    tunnel: w2164 -> [_ w2182]
                    frame False {
                      # "Receive commands"
                      n610 = call "BRig_RT__Case_Exp__UploadClosedLoop__v3.vi"() -> ("all rows"=w2181:i64[][], "output_haveCmd"=w2180:bool)  [unwired: 10 in]
                    }
                    frame True {
                      # "Parse commands and update"
                      n611 = Array Size(array=w2182) -> (size(s)=w2187:i32[])
                      n612 = Index Array(array=w2187, index=0) -> (element=w2185:i32)
                      n613 = Not Equal To 0?(x=w2185) -> (x != 0?=w2184:bool)
                      n614 = case shown="False" w2184 {
                        selector: w2184 -> [w2195 w2197]
                        tunnel: w2191 -> [w2193 w2201]
                        tunnel: [w2193 w2200] -> w2190
                        tunnel: w2189 -> [w2192 w2199]
                        tunnel: [w2192 w2198] -> w2188
                        tunnel: [w2195 w2197] -> w2183
                        tunnel: w2182 -> [_ w2196]
                        frame False {
                          w2194 = TRUE ("input_setValues")
                          # "Update"
                          n615 = call "BRig_RT_panel_cue_v1,10.vi"("input_setValues"=w2194, "input_dataExp"=w2193) -> ()  [unwired: 9 in, 1 out]
                          n616 = call "BRig_RT_panel_ExpStruct_v1,13.vi"("input_setValues"=w2194, "input_dataExp"=w2193) -> ()  [unwired: 9 in, 1 out]
                          n617 = call "BRig_RT_panel_Laser1_v1,12.vi"("input_setValues"=w2194, "input_dataExp"=w2193, "input_dataLC"=w2192) -> ()  [unwired: 7 in, 2 out]
                          n618 = call "BRig_RT_panel_Laser2_v1,12.vi"("input_setValues"=w2194, "input_dataExp"=w2193, "input_dataLC"=w2192) -> ()  [unwired: 7 in, 2 out]
                        }
                        frame True {
                          # "Parse"
                          n619 = call "BRig_RT__Case_Exp__UploadClosedLoop__updateSettings.vi"("input_newSettings"=w2196, "input_dataLC"=w2199, "input_dataExp"=w2201) -> ("output_dataLC"=w2198:u16[], "output_dataExp"=w2200:u16[])  [unwired: 7 in]
                        }
                      }
                    }
                  }
                  n620 = Select(t=myRIO_BRig_RT__Case_Exp_stateList."endTrial2", s=w2169, f=myRIO_BRig_RT__Case_Exp_stateList."endTrial3" ("Enum")) -> (s? t:f=w2170:T2)
                }
                frame "endTrial3" {
                  n621 = call "BRig_RT__Case_Exp__endTrial_checkFreeReward__v10.vi"("input_dataBlock"=w2203, "input_dataExp"=w2212, "input_dataTrial"=w2213, "input_dataCurrent"=w2214) -> ("output_state"=w2204:T2, "output_endBlock"=w2202:bool)  [unwired: 6 in]
                  n622 = local read "STOP_endTrial"() -> (w2211:bool)
                  n623 = local read "STOP_abort"() -> (w2210:bool)
                  n624 = local read "START"() -> (w2208:bool)
                  n625 = Not(x=w2208) -> (.not. x?=w2209:bool)
                  n626 = Compound Arithmetic op=OR(w2211, w2209, w2210, w2202) -> (w2207:bool)
                  n627 = Select(t=myRIO_BRig_RT__Case_Exp_stateList."saveData_dataBlock" ("Enum"), s=w2207, f=w2204) -> (s? t:f=w2205:T2)
                }
                frame "endBlock" {
                  # "Get latest\nlaserSwitch"
                  n628 = call "BRig_dataExp_Loop_c_ExpStruct.vi"() -> ("output_Loop_c_ExpStruct"=w2223:i32)  [unwired: 11 in]
                  n629 = call "BRig_dataExp_LaserSwitch.vi"() -> ("output_LaserSwitch"=w2218:i32)  [unwired: 11 in]
                  n630 = local read "START"() -> (w2242:bool)
                  n631 = local read "STOP_endBlock"() -> (w2238:bool)
                  n632 = local read "STOP_endTrial"() -> (w2240:bool)
                  n633 = local read "STOP_abort"() -> (w2239:bool)
                  n634 = Replace Array Subset(array=w2216, new element=u16 2 ("new element/subarray"), index=w2223) -> (w2221:u16[])
                  n635 = call "BRig_RT_panel_ExpStruct_v1,13.vi"("input_setValues"=FALSE, "input_dataExp"=w2221) -> ("output_dataExp"=w2220:u16[])  [unwired: 9 in]
                  n636 = Index Array(array=w2220, index=w2218) -> (element=w2217:u16)
                  n637 = Not(x=w2242) -> (.not. x?=w2241:bool)
                  n638 = Select(t=myRIO_BRig_RT__Case_Exp_stateList."commUpload_dataTrial" ("Enum"), s=w2228, f=myRIO_BRig_RT__Case_Exp_stateList."initBlock" ("Enum")) -> (s? t:f=w2225:T2)
                  n639 = Replace Array Subset(array=w2216, new element=w2217, index=w2218) -> (w2219:u16[])
                  n640 = Compound Arithmetic op=OR(w2241, w2238, w2240, w2239) -> (w2232:bool)
                  n641 = Select(t=myRIO_BRig_RT__Case_Exp_stateList."endExp" ("Enum"), s=w2232, f=w2225) -> (s? t:f=w2243:T2)
                  n642 = Select(t="<S,E>" ("string"), s=w2232, f="") -> (s? t:f=w2229:string)
                }
                frame "endExp" {
                  n643 = xnode "Read/Write Control"("FPGA VI Reference In"=w2247, "error in"=w2246, "A6_Act"=FALSE) -> ("error out"=w2248:errorcluster)  [unwired: 1 out]
                  n644 = local write "error out"(w2248) -> ()
                }
                frame "commUpload_dataTrial" {
                }
                frame "saveData_dataBlock" {
                  n645 = Increment(x=w2277) -> (x+1=w2275:u16)
                  n646 = Replace Array Subset(array=w2269, new element=u16 2 ("new element/subarray"), index=0) -> (w2263:u16[])
                  n647 = Index Array(array=w2261, index (row)=0) -> (element=w2264:u16[])  [unwired: 1 in]
                  n648 = for {
                    tunnel: w2264 -> [w2287] mode=indexing
                    shift-right: [w2286] -> w2262
                    shift-left: w2263 -> [w2290]
                    i -> [w2289]
                    n649 = Increment(x=w2289) -> (x+1=w2288:i32)
                    n650 = Replace Array Subset(array=w2290, new element=w2287, index=w2288) -> (w2286:u16[])
                  }
                  n651 = RT FIFO Write(0:w2272, 1:w2262, 3:w2271) -> (11:w2274:errorcluster)  [unwired: 2 in, 3 out]
                  n652 = Unbundle By Name(w2274) -> ("code"=w2273:i32)
                  n653 = Greater?(x=w2275, y=u16 3) -> (0:w2283:bool)
                  n654 = Equal To 0?(x=w2273) -> (x = 0?=w2270:bool)
                  n655 = Or(x=w2283, y=w2270) -> (x .or. y?=w2282:bool)
                  n656 = Select(t=myRIO_BRig_RT__Case_Exp_stateList."endBlock" ("Enum"), s=w2282, f=w2278) -> (s? t:f=w2276:T2)
                }
                frame "saveData_dataTrial" {
                  n657 = Increment(x=w2308) -> (x+1=w2307:u16)
                  n658 = Replace Array Subset(array=w2293, new element=u16 1 ("new element/subarray"), index=0) -> (w2297:u16[])
                  n659 = Index Array(array=w2292, index (row)=0) -> (element=w2298:u16[])  [unwired: 1 in]
                  n660 = for {
                    tunnel: w2298 -> [w2317] mode=indexing
                    shift-right: [w2316] -> w2296
                    shift-left: w2297 -> [w2320]
                    i -> [w2319]
                    n661 = Increment(x=w2319) -> (x+1=w2318:i32)
                    n662 = Replace Array Subset(array=w2320, new element=w2317, index=w2318) -> (w2316:u16[])
                  }
                  n663 = RT FIFO Write(0:w2295, 1:w2296, 3:w2294) -> (11:w2303:errorcluster)  [unwired: 2 in, 3 out]
                  n664 = Unbundle By Name(w2303) -> ("code"=w2302:i32)
                  n665 = Equal To 0?(x=w2302) -> (x = 0?=w2291:bool)
                  n666 = Greater?(x=w2307, y=u16 3) -> (0:w2305:bool)
                  n667 = Or(x=w2305, y=w2291) -> (x .or. y?=w2304:bool)
                  n668 = Select(t=myRIO_BRig_RT__Case_Exp_stateList."endTrial2" ("Enum"), s=w2304, f=w2309) -> (s? t:f=w2310:T2)
                }
                frame "dummyState" {
                  n669 = call "BRig_dataCurrent_iTrial.vi"() -> ("output_iTrial"=w2327:i32)  [unwired: 11 in]
                  n670 = Index Array(array=w2328, index=w2327) -> (element=w2326:u16)
                  n671 = Equal?(x=w2326, y=u16 1) -> (x = y?=w2324:bool)
                  n672 = Equal To 0?(x=w2335) -> (x = 0?=w2336:bool)
                  n673 = Select(t=u16 13, s=w2324, f=u16 15) -> (s? t:f=w2321:u16)
                  n674 = Select(t=w2321, s=w2336, f=w2335) -> (s? t:f=w2334:u16)
                  n675 = Decrement(x=w2334) -> (x-1=w2333:u16)
                  n676 = Equal To 0?(x=w2333) -> (x = 0?=w2332:bool)
                  n677 = Select(t=myRIO_BRig_RT__Case_Exp_stateList."initTrial" ("Enum"), s=w2332, f=w2330) -> (s? t:f=w2329:T2)
                }
                frame "dummyState_endBlock" {
                  n678 = call "BRig_dataCurrent_iTrial.vi"() -> ("output_iTrial"=w2351:i32)  [unwired: 11 in]
                  n679 = Index Array(array=w2345, index=w2351) -> (element=w2341:u16)
                  n680 = Equal?(x=w2341, y=u16 1) -> (x = y?=w2349:bool)
                  n681 = Equal To 0?(x=w2342) -> (x = 0?=w2353:bool)
                  n682 = Select(t=u16 1, s=w2349, f=u16 3) -> (s? t:f=w2346:u16)
                  n683 = Select(t=w2346, s=w2353, f=w2342) -> (s? t:f=w2352:u16)
                  n684 = Decrement(x=w2352) -> (x-1=w2343:u16)
                  n685 = Equal To 0?(x=w2343) -> (x = 0?=w2344:bool)
                  n686 = Select(t=myRIO_BRig_RT__Case_Exp_stateList."initBlock" ("Enum"), s=w2344, f=w2355) -> (s? t:f=w2354:T2)
                }
                frame "FreeReward_pre" {
                  w2391 = u16 0 ("new element/subarray")
                  # "Duration = MTrig duration"
                  # "Duration = Reward Time"
                  n687 = call "BRig_dataCurrent_FreeReward_c.vi"() -> ("output_FreeReward_c"=w2392:i32)  [unwired: 11 in]
                  n688 = call "BRig_dataCurrent_iSpout.vi"() -> ("output_iSpout"=w2389:i32)  [unwired: 11 in]
                  n689 = call "BRig_dataCurrent_c_generic.vi"() -> ("output_count_generic"=w2398:i32)  [unwired: 11 in]
                  n690 = call "BRig_dataCurrent_T_generic.vi"() -> ("output_T_generic"=w2397:i32)  [unwired: 11 in]
                  n691 = Index Array(array=w2390, index=w2389) -> (element=w2388:u16)
                  n692 = call "BRig_dataMTrig_Solenoid_T_L.vi"() -> ("output_Solenoid_T_L"=w2387:i32)  [unwired: 11 in]
                  n693 = call "BRig_dataMTrig_Solenoid_T_R.vi"() -> ("output_Solenoid_T_R"=w2386:i32)  [unwired: 11 in]
                  n694 = local read "FPGA_count2ms"() -> (w2368:dbl)
                  n695 = call "BRig_dataTrial_T_Reward.vi"() -> ("output_T_Reward"=w2393:i32)  [unwired: 11 in]
                  n696 = Equal To 0?(x=w2388) -> (x = 0?=w2370:bool)
                  n697 = Select(t=w2387, s=w2370, f=w2386) -> (s? t:f=w2384:i32)
                  n698 = Index Array(array=w2394, index (row)=0 ("disabled index (row)"), index (col)=w2393) -> ()  [unwired: 1 out]
                  n699 = Index Array(array=w2385, index=w2384) -> (element=w2381:u16)
                  n700 = Replace Array Subset(array=w2390, new element #1=w2391, index #1=w2392, new element #2=w2391, index #2=w2398, new element #3=w2381, index #3=w2397) -> (w2396:u16[])
                  n701 = To Double Precision Float(number=w2381) -> (double precision float=w2369:dbl)
                  n702 = Multiply(x=w2369, y=w2368) -> (x*y=w2382:dbl)
                  n703 = call "BRig_dataExp_FreeReward_c_L.vi"() -> ("output_FreeReward_c_L"=w2375:i32)  [unwired: 11 in]
                  n704 = call "BRig_dataExp_FreeReward_c_R.vi"() -> ("output_FreeReward_c_R"=w2376:i32)  [unwired: 11 in]
                  n705 = Round Toward +Infinity(x=w2382) -> (ceil(x): smallest int >= x=w2383:dbl)
                  n706 = Select(t=w2375, s=w2370, f=w2376) -> (s? t:f=w2372:i32)
                  n707 = To Unsigned Long Integer(number=w2383) -> (unsigned 32bit integer=w2378:u32)
                  n708 = xnode "Read/Write Control"("FPGA VI Reference In"=w2380, "error in"=w2379, "Solenoid_nTotal_L"=w2378, "Solenoid_nTotal_R"=w2378) -> ()  [unwired: 2 out]
                  n709 = Index Array(array=w2373, index=w2372) -> (element=w2371:u16)
                  n710 = Increment(x=w2371) -> (x+1=w2361:u16)
                  n711 = case shown="True" w2370 {
                    tunnel: w2361 -> [w2402 w2404]
                    tunnel: [w2401 w2403] -> w2363
                    frame True {
                      n712 = local write "FreeReward_c_L"(w2402) -> ()
                      n713 = call "BRig_dataRT_stats__FreeReward_c_L.vi"() -> ("output_FreeReward_c_L"=w2401:i32)  [unwired: 11 in]
                    }
                    frame False {
                      n714 = local write "FreeReward_c_R"(w2404) -> ()
                      n715 = call "BRig_dataRT_stats__FreeReward_c_R.vi"() -> ("output_FreeReward_c_R"=w2403:i32)  [unwired: 11 in]
                    }
                  }
                  n716 = To Unsigned Word Integer(number=w2363) -> (unsigned 16bit integer=w2362:u16)
                  n717 = Build Array(u16 3, w2362, w2361) -> (w2367:u16[])
                  n718 = Replace Array Subset(array=w2373, new element=w2361, index=w2372) -> (w2374:u16[])
                  n719 = RT FIFO Write(0:w2365, 1:w2367, 3:w2364) -> ()  [unwired: 2 in, 4 out]
                }
                frame "FreeReward" {
                  n720 = call "BRig_dataCurrent_iSpout.vi"() -> ("output_iSpout"=w2415:i32)  [unwired: 11 in]
                  n721 = call "BRig_dataCurrent_c_generic.vi"() -> ("output_count_generic"=w2409:i32)  [unwired: 11 in]
                  n722 = Index Array(array=w2416, index #1=w2415, index #2=w2409) -> (element #1=w2414:u16, element #2=w2408:u16)
                  n723 = Equal To 0?(x=w2414) -> (x = 0?=w2412:bool)
                  n724 = Equal To 0?(x=w2408) -> (x = 0?=w2407:bool)
                  n725 = Not(x=w2412) -> (.not. x?=w2413:bool)
                  n726 = call "BRig_RT__Case_Exp__generic__incrementCountTilThreshold.vi"("input_dataCurrent"=w2416) -> ("output_dataCurrent"=w2417:u16[], "output_underThreshold"=w2406:bool)  [unwired: 9 in]
                  n727 = Select(t=w2420, s=w2406, f=myRIO_BRig_RT__Case_Exp_stateList."FreeRewardPost_pre" ("Enum")) -> (s? t:f=w2418:T2)
                  n728 = And(x=w2406, y=w2407) -> (x .and. y?=w2405:bool)
                  n729 = And(x=w2405, y=w2412) -> (x .and. y?=w2410:bool)
                  n730 = And(x=w2405, y=w2413) -> (x .and. y?=w2411:bool)
                }
                frame "FreeRewardPost" {
                  n731 = call "BRig_RT__Case_Exp__generic__incrementCountTilThreshold.vi"("input_dataCurrent"=w2427) -> ("output_dataCurrent"=w2426:u16[], "output_underThreshold"=w2425:bool)  [unwired: 9 in]
                  n732 = Select(t=w2430, s=w2425, f=myRIO_BRig_RT__Case_Exp_stateList."initTrial" ("Enum")) -> (s? t:f=w2428:T2)
                }
                frame "FreeRewardPost_pre" {
                  n733 = call "BRig_dataExp_T_RewardPost.vi"() -> ("output_T_RewardPost"=w2440:i32)  [unwired: 11 in]
                  n734 = call "BRig_dataCurrent_c_generic.vi"() -> ("output_count_generic"=w2443:i32)  [unwired: 11 in]
                  n735 = call "BRig_dataCurrent_T_generic.vi"() -> ("output_T_generic"=w2442:i32)  [unwired: 11 in]
                  n736 = Index Array(array=w2437, index=w2440) -> (element=w2439:u16)
                  n737 = Replace Array Subset(array=w2438, new element #1=u16 0 ("new element/subarray"), index #1=w2443, new element #2=w2439, index #2=w2442) -> (w2436:u16[])
                }
              }
              n738 = call "BRig_RT_panel_manualTriggering_v0,90.vi"("input_dataMTrig"=w1308) -> ("output_Solenoid_R"=w1319:bool, "output_Solenoid_L"=w1318:bool, "output_dataMTrig"=w1351:u16[], "output_Audio_L"=w1350:bool, "output_Audio_R"=w1349:bool, "output_CueLed"=w1347:bool, "output_Laser_l1"=w1323:bool, "output_Laser_l2"=w1343:bool)  [unwired: 11 in]
              n739 = call "BRig_RT__Case_Exp__comm_tcp__data_other.vi"("input_strState"=w1311, "input_strAccum"=w1312, "input_error"=w1313, "input_hTCP"=w1314, "input_I_connected_TCP"=w1315) -> ("output_strAccum"=w1294:string, "output_error"=w1293:errorcluster, "output_hTCP"=w1295:refnum<k5>, "output_I_connect_TCP"=w1296:bool)  [unwired: 3 in]
              n740 = Or(x="STOP_abort", y=w1335) -> (x .or. y?=w1297:bool)
              n741 = Or(x=w1348, y=w1347) -> (x .or. y?=w1326:bool)
              n742 = local read "Laser1_LED"() -> (w1284:bool)
              n743 = local read "Laser2_LED"() -> (w1283:bool)
              n744 = Or(x=w1350, y=w1365) -> (x .or. y?=w1325:bool)
              n745 = Or(x=w1364, y=w1349) -> (x .or. y?=w1324:bool)
              n746 = Or(x=w1322, y=w1323) -> (x .or. y?=w1342:bool)
              n747 = Or(x=w1346, y=w1343) -> (x .or. y?=w1344:bool)
              n748 = call "BRig_RT__Case_Exp__recordLick.vi"("input_dataLick"=w1334, "input_lick__R"=w1328, "input_lick__L"=w1329, "input_lick"=w1330, "intput_state__trialStart"=w1288, "intput_state__trialEnd"=w1333, "input_dataCurrent"=w1332) -> ("output_dataLick"=w1327:u16[][], "output_dataCurrent"=w1331:u16[])  [unwired: 7 in]
              n749 = xnode "Read/Write Control"("FPGA VI Reference In"=w1363, "error in"=w1362, "L1Led_ON"=w1284, "L2Led_ON"=w1283, "Solenoid_trig_L"=w1317, "Solenoid_trig_R"=w1316, "A3_SL"=w1318, "A1_SR"=w1319, "LC_Event_l1"=w1341, "LC_Laser_l1"=w1342, "LC_Event_l2"=w1345, "LC_Laser_l2"=w1344, "CueLed_Event"=w1326, "audioTrigger_L"=w1325, "audioTrigger_R"=w1324) -> ("FPGA VI Reference Out"=w1369:refnum<k20>, "error out"=w1368:errorcluster, "fpga_laser1"=w1282:bool, "fpga_laser2"=w1281:bool, "fpga_solenoid_L"=w1280:bool, "fpga_solenoid_R"=w1279:bool, "AnaIn_0"=w1309:i16, "AnaIn_1"=w1310:i16)
              n750 = local write "Laser1"(w1282) -> ()
              n751 = local write "Laser2"(w1281) -> ()
              n752 = local write "Solenoid L"(w1280) -> ()
              n753 = local write "Solenoid R"(w1279) -> ()
              n754 = call "BRig_RT__Case_Exp__recordAnalogInput__PortC__fifo__1value.vi"("input_iOccurence"=w1339, "resetOccurrence"=w1338, "input_dataCurrent"=w1332, "input_iState_start"=w1288, "rt fifo"=w1287, "input_iState_end"=w1333, "input_fifo_error"=w1286, "input_AI1"=w1310, "input_AI0"=w1309) -> ("output_fifo_error"=w1292:errorcluster, "output_iOccurrence"=w1340:u16)  [unwired: 8 in, 1 out]
              n755 = call "BRig_RT_timeLoop_Exp__noStateLimit.vi"("input_error"=w1292, "input_Threshold_reset"="input_Threshold_reset", "input_Threshold"=w1354, "input_timestamp"=w1355, "input_state"=w1288) -> ("output_Threshold"=w1352:bool, "output_duration"=→"tLoop":dbl)  [unwired: 4 in, 1 out]
              "Threshold" <- w1352
              n756 = node-c288() -> ()  [unwired: 1 in, 1 out]
            }
            "stop_TimedLoop" <- w893
            n757 = while {
              tunnel: w837 -> [w961]
              tunnel: w836 -> [w960]
              shift-right: [w955] -> _
              shift-left: 0 ("element") -> [w956]
              shift-right: [w951] -> _
              shift-left: w842 -> [w957]
              tunnel: [w954] -> w839
              tunnel: [w953] -> w838
              tunnel: w835 -> [w950]
              tunnel: w834 -> [w949]
              tunnel: [w948] -> w833
              tunnel: [w947] -> w832
              shift-right: [w945] -> _
              shift-left: FALSE -> [w946]
              stop <- w944 stop-if-true
              # "timed out?"
              n758 = RT FIFO Read(0:w961, 3:w960) -> (8:w954:refnum<k33>, 9:w958:u16, 10:w965:bool, 11:w962:errorcluster)  [unwired: 2 in, 1 out]
              n759 = Unbundle By Name(w962) -> ("code"=w966:i32)
              n760 = Not(x=w965) -> (.not. x?=w964:bool)
              n761 = Equal To 0?(x=w966) -> (x = 0?=w963:bool)
              n762 = And(x=w963, y=w964) -> (x .and. y?=w959:bool)
              n763 = Select(t=w962, s=w963, f=w960) -> (s? t:f=w953:errorcluster)
              n764 = case shown="True" w959 {
                tunnel: w958 -> [_ w997]
                tunnel: w957 -> [w989 w999]
                tunnel: w956 -> [w988 w996]
                tunnel: [w989 w998] -> w951
                tunnel: [w988 w992] -> w955
                tunnel: [_ w990] -> w952
                frame False {
                }
                frame True {
                  n765 = Replace Array Subset(array=w999, new element=w997, index=w996) -> (w998:u16[])
                  n766 = Increment(x=w996) -> (x+1=w994:i32)
                  n767 = Less?(x=w996, y=7 ("dimension size")) -> (x < y?=w991:bool)
                  n768 = Select(t=w994, s=w991, f=0) -> (s? t:f=w992:i32)
                  n769 = Not(x=w991) -> (.not. x?=w990:bool)
                }
              }
              n770 = case shown="True" w952 {
                tunnel: w951 -> [_ w978]
                tunnel: w950 -> [w969 w977]
                tunnel: w949 -> [w968 w976]
                tunnel: [w969 w974] -> w948
                tunnel: [w968 w973] -> w947
                tunnel: w946 -> [w967 w971]
                tunnel: [w967 w970] -> w945
                frame False {
                }
                frame True {
                  n771 = for {
                    N: 8 -> [_]
                    tunnel: w978 -> [w985] mode=indexing
                    tunnel: w977 -> [w987]
                    tunnel: w976 -> [w986]
                    shift-right: [w980] -> w972
                    shift-left: FALSE -> [w984]
                    tunnel: [w983] -> w974
                    tunnel: [w982] -> w973
                    n772 = shared-variable-write(w987, w986, w985) -> (w983:refnum<k21>, w982:errorcluster, w981:bool)  [unwired: 1 in]
                    n773 = Or(x=w984, y=w981) -> (x .or. y?=w980:bool)
                  }
                  n774 = Or(x=w971, y=w972) -> (x .or. y?=w970:bool)
                }
              }
              n775 = local read "stop_TimedLoop"() -> (w944:bool)
            }
            n776 = while {
              shift-right: [w1070] -> _
              shift-left: 0 -> [w1059]
              tunnel: w890 -> [w1077]
              tunnel: w882 -> [w1079]
              shift-right: [w1066] -> _
              shift-left: 0 -> [w1061]
              shift-right: [w1071] -> _
              shift-left: w829 -> [w1078]
              shift-right: [w1067] -> _
              shift-left: w857 -> [w1080]
              shift-right: [w1074] -> w879
              shift-left: w851 -> [w1087]
              shift-right: [w1075] -> w873
              shift-left: w850 -> [w1081]
              tunnel: w854 -> [w1064]
              tunnel: w858 -> [w1063]
              shift-right: [w1052] -> _
              shift-left: w824 -> [w1058]
              shift-right: [w1051] -> _
              shift-left: 0 -> [w1057]
              tunnel: w827 -> [w1055]
              tunnel: w826 -> [w1056]
              tunnel: [w1050] -> w821
              tunnel: [w1049] -> w820
              stop <- w1088 stop-if-true
              # "nColumns dataBlock"
              # "nColumns dataTrial"
              # "buffer_dataTrial"
              # "buffer_dataBlock"
              # "buffer_dataTrial"
              # "buffer_dataBlock"
              n777 = local read "stop_TimedLoop"() -> (w1088:bool)
              n778 = Not Equal To 0?(x=w1061) -> (x != 0?=w1062:bool)
              n779 = Not Equal To 0?(x=w1057) -> (x != 0?=w1048:bool)
              n780 = case shown="True" w1062 {
                tunnel: w1080 -> [w1240 w1243]
                tunnel: w1061 -> [w1241 w1245]
                tunnel: w1079 -> [_ w1254]
                tunnel: [w1241 w1242] -> w1068
                tunnel: [w1240 w1243] -> w1069
                frame False {
                }
                frame True {
                  n781 = Array Subset(array=w1243, length (row)=w1245) -> (w1256:u16[][])  [unwired: 3 in]
                  n782 = call "BRig_dataBlock_iBlock.vi"() -> ("output_iBlock"=w1251:i32)  [unwired: 11 in]
                  n783 = Index Array(array=w1243, index (row)=0, index (col)=w1251) -> (element=w1250:u16)
                  n784 = To Double Precision Float(number=w1256) -> (double precision float=w1255:dbl[][])
                  n785 = Not Equal?(x=u16 1, y=w1250) -> (x != y?=w1248:bool)
                  n786 = call-poly <vilib>:"Write To Spreadsheet File.vi"("delimiter (\\t)"="," ("delimiter (\\t)"), "append to file? (new file:F)"=w1248, "2D data"=w1255, "file path (dialog if empty)"=w1254) -> ("new file path (Not A Path if cancelled)"=w1247:path)  [unwired: 4 in]
                  n787 = call <vilib>:"Is Path and Not Empty.vi"("path"=w1247) -> ("Is Path and Not Empty?"=w1246:bool)  [unwired: 4 in]
                  n788 = Select(t=0, s=w1246, f=w1245) -> (s? t:f=w1242:i32)
                }
              }
              n789 = case shown="True" w1048 {
                tunnel: w1058 -> [w1092 w1101]
                tunnel: w1057 -> [w1091 w1094]
                tunnel: [w1091 w1100] -> w1053
                tunnel: [w1092 w1101] -> w1054
                tunnel: w1056 -> [w1090 w1109]
                tunnel: w1055 -> [w1089 w1108]
                tunnel: [w1090 w1099] -> w1050
                tunnel: [w1089 w1098] -> w1049
                frame False {
                }
                frame True {
                  n790 = Decrement(x=w1094) -> (x-1=w1093:i32)
                  n791 = Multiply(x=w1093, y=2 ("index")) -> (x*y=w1095:i32)
                  n792 = Increment(x=w1095) -> (x+1=w1096:i32)
                  n793 = Index Array(array=w1101, index #1=w1095, index #2=w1096) -> (element #1=w1107:u16, element #2=w1103:u16)
                  n794 = shared-variable-write(w1109, w1108, w1107) -> (w1104:refnum<k21>, w1105:errorcluster, w1106:bool)  [unwired: 1 in]
                  n795 = case shown="False" w1106 {
                    selector: w1106 -> [_ w1118]
                    tunnel: w1105 -> [w1115 w1116]
                    tunnel: w1104 -> [w1114 w1117]
                    tunnel: w1103 -> [w1113 _]
                    tunnel: [w1112 w1118] -> w1102
                    tunnel: [w1111 w1117] -> w1099
                    tunnel: [w1110 w1116] -> w1098
                    frame False {
                      n796 = shared-variable-write(w1114, w1115, w1113) -> (w1111:refnum<k21>, w1110:errorcluster, w1112:bool)  [unwired: 1 in]
                    }
                    frame True {
                    }
                  }
                  n797 = Select(t=w1094, s=w1102, f=w1093) -> (s? t:f=w1100:i32)
                }
              }
              n798 = RT FIFO Read(0:w1087, 3:w1081) -> (8:w1074:refnum<k33>, 9:w1065:u16[], 10:w1085:bool, 11:w1082:errorcluster)  [unwired: 2 in, 1 out]
              n799 = Unbundle By Name(w1082) -> ("code"=w1086:i32)
              n800 = Not(x=w1085) -> (.not. x?=w1084:bool)
              n801 = Equal To 0?(x=w1086) -> (x = 0?=w1083:bool)
              n802 = And(x=w1083, y=w1084) -> (x .and. y?=w1076:bool)
              n803 = Select(t=w1082, s=w1083, f=w1081) -> (s? t:f=w1075:errorcluster)
              n804 = Not Equal To 0?(x=w1059) -> (x != 0?=w1060:bool)
              n805 = case shown="True" w1060 {
                tunnel: w1078 -> [w1223 w1226]
                tunnel: w1059 -> [w1224 w1228]
                tunnel: w1077 -> [_ w1237]
                tunnel: [w1224 w1225] -> w1072
                tunnel: [w1223 w1226] -> w1073
                frame False {
                }
                frame True {
                  n806 = Array Subset(array=w1226, length (row)=w1228) -> (w1239:u16[][])  [unwired: 3 in]
                  n807 = call "BRig_dataTrial_nTrial.vi"() -> ("output_nTrial"=w1234:i32)  [unwired: 11 in]
                  n808 = Index Array(array=w1226, index (row)=0, index (col)=w1234) -> (element=w1233:u16)
                  n809 = To Double Precision Float(number=w1239) -> (double precision float=w1238:dbl[][])
                  n810 = Not Equal?(x=u16 1, y=w1233) -> (x != y?=w1231:bool)
                  n811 = call-poly <vilib>:"Write To Spreadsheet File.vi"("delimiter (\\t)"="," ("delimiter (\\t)"), "append to file? (new file:F)"=w1231, "2D data"=w1238, "file path (dialog if empty)"=w1237) -> ("new file path (Not A Path if cancelled)"=w1230:path)  [unwired: 4 in]
                  n812 = call <vilib>:"Is Path and Not Empty.vi"("path"=w1230) -> ("Is Path and Not Empty?"=w1229:bool)  [unwired: 4 in]
                  n813 = Select(t=0, s=w1229, f=w1228) -> (s? t:f=w1225:i32)
                }
              }
              n814 = case shown="True" w1076 {
                tunnel: w1073 -> [w1125 w1145]
                tunnel: w1072 -> [w1124 w1143]
                tunnel: [w1125 w1144] -> w1071
                tunnel: [w1124 w1142] -> w1070
                tunnel: w1069 -> [w1123 w1141]
                tunnel: w1068 -> [w1122 w1139]
                tunnel: [w1123 w1140] -> w1067
                tunnel: [w1122 w1138] -> w1066
                tunnel: w1065 -> [_ w1146]
                tunnel: w1064 -> [_ w1137]
                tunnel: w1063 -> [_ w1136]
                tunnel: w1054 -> [w1120 w1129]
                tunnel: w1053 -> [w1119 w1128]
                tunnel: [w1120 w1127] -> w1052
                tunnel: [w1119 w1126] -> w1051
                frame False {
                  n815 = Wait (ms)(milliseconds to wait=u32 10) -> ()  [unwired: 1 out]
                }
                frame True {
                  n816 = Index Array(array=w1146, index=0) -> (element=w1130:u16)
                  n817 = Equal?(x=w1130, y=u16 1) -> (x = y?=w1131:bool)
                  n818 = Equal?(x=w1130, y=u16 2) -> (x = y?=w1133:bool)
                  n819 = Or(x=w1131, y=w1133) -> (x .or. y?=w1132:bool)
                  n820 = case shown="False" w1132 {
                    tunnel: w1146 -> [w1154 w1202]
                    tunnel: w1145 -> [w1158 w1195]
                    tunnel: [w1158 w1194] -> w1144
                    tunnel: w1143 -> [w1157 w1193]
                    tunnel: [w1157 w1192] -> w1142
                    tunnel: w1141 -> [w1156 w1199]
                    tunnel: [w1156 w1197] -> w1140
                    tunnel: w1139 -> [w1155 w1198]
                    tunnel: [w1155 w1196] -> w1138
                    tunnel: w1137 -> [_ w1201]
                    tunnel: w1136 -> [_ w1200]
                    tunnel: w1131 -> [_ w1191]
                    tunnel: w1130 -> [w1159 _]
                    tunnel: w1129 -> [w1151 w1190]
                    tunnel: w1128 -> [w1152 w1189]
                    tunnel: [w1150 w1190] -> w1127
                    tunnel: [w1149 w1189] -> w1126
                    frame False {
                      n821 = Equal?(x=w1159, y=u16 3) -> (x = y?=w1148:bool)
                      n822 = case shown="True" w1148 {
                        tunnel: w1154 -> [_ w1166]
                        tunnel: w1152 -> [w1160 w1165]
                        tunnel: w1151 -> [w1161 w1164]
                        tunnel: [w1161 w1163] -> w1150
                        tunnel: [w1160 w1162] -> w1149
                        frame False {
                        }
                        frame True {
                          w1173 = 3 ("y")
                          n823 = Array Size(array=w1166) -> (size(s)=w1167:i32)
                          n824 = To Double Precision Float(number=w1167) -> (double precision float=w1168:dbl)
                          n825 = To Double Precision Float(number=w1173) -> (double precision float=w1172:dbl)
                          n826 = Divide(x=w1168, y=w1172) -> (x/y=w1169:dbl)
                          n827 = Round Toward -Infinity(1:w1169) -> (0:w1170:dbl)
                          n828 = To Long Integer(number=w1170) -> (32bit integer=w1171:i32)
                          n829 = for {
                            N: w1171 -> [_]
                            tunnel: w1173 -> [w1188]
                            tunnel: w1166 -> [w1185]
                            shift-right: [w1174] -> w1162
                            shift-left: w1165 -> [w1180]
                            shift-right: [w1175] -> w1163
                            shift-left: w1164 -> [w1182]
                            i -> [w1187]
                            n830 = Multiply(x=2 ("index"), y=w1180) -> (x*y=w1179:i32)
                            n831 = Multiply(x=w1187, y=w1188) -> (x*y=w1186:i32)
                            n832 = Increment(x=w1186) -> (x+1=w1184:i32)
                            n833 = Increment(x=w1184) -> (x+1=w1183:i32)
                            n834 = Increment(x=w1180) -> (x+1=w1174:i32)
                            n835 = Index Array(array=w1185, index #1=w1184, index #2=w1183) -> (element #1=w1177:u16, element #2=w1176:u16)
                            n836 = Increment(x=w1179) -> (x+1=w1178:i32)
                            n837 = Replace Array Subset(array=w1182, new element #1=w1177, index #1=w1179, new element #2=w1176, index #2=w1178) -> (w1175:u16[])
                          }
                        }
                      }
                    }
                    frame True {
                      n838 = case shown="True" w1191 {
                        tunnel: w1202 -> [w1210 w1222]
                        tunnel: w1201 -> [w1208 _]
                        tunnel: w1200 -> [_ w1217]
                        tunnel: w1199 -> [w1212 w1216]
                        tunnel: w1198 -> [w1211 w1218]
                        tunnel: [w1212 w1215] -> w1197
                        tunnel: [w1211 w1214] -> w1196
                        tunnel: w1195 -> [w1207 w1219]
                        tunnel: [w1205 w1219] -> w1194
                        tunnel: w1193 -> [w1204 w1213]
                        tunnel: [w1203 w1213] -> w1192
                        frame True {
                          n839 = Array Subset(array=w1210, index=1, length=w1208) -> (w1206:u16[])
                          n840 = Increment(x=w1204) -> (x+1=w1203:i32)
                          n841 = Replace Array Subset(array=w1207, new element=w1206, index (row)=w1204) -> (w1205:u16[][])  [unwired: 1 in]
                        }
                        frame False {
                          n842 = Array Subset(array=w1222, index=1, length=w1217) -> (w1220:u16[])
                          n843 = Increment(x=w1218) -> (x+1=w1214:i32)
                          n844 = Replace Array Subset(array=w1216, new element=w1220, index (row)=w1218) -> (w1215:u16[][])  [unwired: 1 in]
                        }
                      }
                    }
                  }
                }
              }
            }
            n845 = node-c288(w942) -> ()  [unwired: 1 out]
            n846 = RT FIFO Delete(0:w879, 2:TRUE ("force destroy? (F)"), 3:w873) -> ()  [unwired: 1 out]
            n847 = RT FIFO Delete(0:w839, 2:TRUE ("force destroy? (F)"), 3:w838) -> ()  [unwired: 1 out]
            n848 = flat-sequence {
              tunnel: w913 -> [w1258]
              tunnel: w912 -> [w1261]
              tunnel: w911 -> [w1260]
              tunnel: w910 -> [w1259]
              tunnel: w909 -> [w1263]
              tunnel: w907 -> [_]
              tunnel: w830 -> [w1265]
              tunnel: w877 -> [w1264]
              tunnel: [w1257] -> w888
              tunnel: w873 -> [_]
              tunnel: w906 -> [w1276]
              tunnel: w905 -> [w1275]
              tunnel: w904 -> [w1274]
              tunnel: [w1273] -> w903
              tunnel: [w1272] -> w902
              tunnel: [w1267] -> w898
              tunnel: w888 -> [w1266]
              frame #0 {
                # "Store"
                n849 = call "BRig_RT__Case_Exp__storeData__endExp__v5__p1.vi"("input_dataCurrent"=w1259, "input_dataLC"=w1264, "input_dataExp"=w1265, "input_dataExp_end"=w1260, "input_dataLC_end"=w1261) -> ("output_True"=w1262:bool)  [unwired: 10 in]
                n850 = call "BRig_RT__Case_Exp__storeData__endExp__v5__p2.vi"("input_dataCurrent"=w1259, "input_dataLick"=w1263, "input_True"=w1262, "input_dataMTrig"=w1258) -> ("output_True"=w1257:bool)  [unwired: 11 in]
              }
              frame #1 {
                # "Send"
                n851 = local read "Data Set Prefix"() -> (w1268:string)
                n852 = call "BRig_RT_comm_webdav_upload_all__v3.vi"("input_I_connected_webdav"=w1274, "input_fileName_prefix"=w1268, "input_hSession"=w1275, "input_error"=w1276, "input_True"=w1266) -> ("output_hSession"=w1272:T4, "error out"=w1273:errorcluster, "output_nFilenames"=w1269:i32, "output_arrFilenames"=w1270:string[], "output_uploaded"=w1271:bool[], "output_strCmd"=w1267:string)  [unwired: 5 in]
                n853 = call "BRig_RT_comm_webdav_upload_all_warnUser.vi"("input_n"=w1269, "input_arrFilenames"=w1270, "input_arrUploaded"=w1271) -> ()  [unwired: 9 in]
              }
            }
            n854 = flat-sequence {
              tunnel: w922 -> [w1277]
              tunnel: [w1277] -> w908
              frame #0 {
                w1278 = FALSE ("START")
                n855 = local write "START"(w1278) -> ()
                n856 = local write "STOP_endTrial"(w1278) -> ()
                n857 = local write "STOP_endBlock"(w1278) -> ()
              }
            }
            n858 = xnode "Read/Write Control"("FPGA VI Reference In"=w939, "error in"=w908, "Counts_Reset"=TRUE, "audioTrigger_L"=w925, "audioFreq_L_kHz"=w923, "audioAmp_L"=w924, "audioTrigger_R"=w925, "audioFreq_R_kHz"=w923, "audioAmp_R"=w924, "A3_SL"=w925, "A1_SR"=w925, "A6_Act"=w925) -> ("FPGA VI Reference Out"=w938:refnum<k20>, "error out"=w907:errorcluster)
            n859 = call "BRig_RT__Case_Exp__comm_tcp__data_other.vi"("input_strState"=w898, "input_strAccum"="" ("f"), "input_error"=w899, "input_hTCP"=w900, "input_I_connected_TCP"=w901) -> ("output_error"=w894:errorcluster, "output_hTCP"=w895:refnum<k5>, "output_I_connect_TCP"=w896:bool)  [unwired: 3 in, 1 out]
          }
        }
        n860 = local read "STOP_abort"() -> (w328:bool)
      }
    }
  }
  n861 = flat-sequence {
    tunnel: w96 -> [w2458]
    tunnel: w95 -> [w2460]
    tunnel: w89 -> [w2459]
    tunnel: [w2459] -> w101
    tunnel: [w2458] -> w100
    tunnel: [w2457] -> w99
    tunnel: w74 -> [w2456]
    tunnel: [w2456] -> w98
    tunnel: w75 -> [w2455]
    tunnel: [w2455] -> w97
    tunnel: w82 -> [w2453]
    tunnel: w81 -> [w2452]
    tunnel: w80 -> [w2451]
    tunnel: w76 -> [w2454]
    tunnel: [w2454] -> w94
    tunnel: w93 -> [_]
    tunnel: [w2453] -> w88
    tunnel: [w2452] -> w87
    tunnel: [w2451] -> w86
    tunnel: w101 -> [w2480]
    tunnel: w100 -> [w2479]
    tunnel: w99 -> [w2478]
    tunnel: [w2477] -> _
    tunnel: w98 -> [w2476]
    tunnel: w97 -> [w2475]
    tunnel: w94 -> [w2474]
    tunnel: w88 -> [w2473]
    tunnel: w87 -> [w2472]
    tunnel: w86 -> [w2471]
    frame #0 {
      # "Stop FPGA\nSend QUIT to Host"
      n862 = case shown="True" w2459 {
        tunnel: w2458 -> [_ w2469]
        tunnel: w2460 -> [w2466 w2468]
        tunnel: [w2466 w2467] -> w2457
        frame False {
        }
        frame True {
          n863 = xnode "Read/Write Control"("FPGA VI Reference In"=w2469, "error in"=w2468, "FPGA_Stop"=TRUE) -> ("error out"=w2467:errorcluster)  [unwired: 1 out]
        }
      }
      n864 = case shown="True" w2453 {
        tunnel: w2452 -> [_ w2465]
        tunnel: w2451 -> [_ w2464]
        frame False {
        }
        frame True {
          w2461 = "<S,Q><S,Q><S,Q><S,Q>" ("input_packet")
          n865 = call "BRig_RT_comm_tcp_write_RTwrite.vi"("input_error"=w2464, "input_packet"=w2461, "input_hTCP"=w2465) -> ("output_error"=w2463:errorcluster, "output_hTCP"=w2462:refnum<k5>)  [unwired: 5 in, 2 out]
          n866 = call "BRig_RT_comm_tcp_write_RTwrite.vi"("input_error"=w2463, "input_packet"=w2461, "input_hTCP"=w2462) -> ()  [unwired: 5 in, 4 out]
        }
      }
    }
    frame #1 {
      # "Disconnect FPGA\nDisconnect comm webdav"
      n867 = case shown="True" w2480 {
        tunnel: w2478 -> [w2485 w2488]
        tunnel: w2479 -> [_ w2487]
        tunnel: [w2485 w2486] -> w2477
        frame False {
        }
        frame True {
          n868 = xnode "Close FPGA VI Reference"("FPGA VI Reference In"=w2487, "error in"=w2488) -> ("error out"=w2489:errorcluster)
          n869 = call <vilib>:"Reset myRIO.vi"("error in (no error)"=w2489) -> ("error out"=w2486:errorcluster)  [unwired: 10 in]
        }
      }
      n870 = case shown="True" w2473 {
        tunnel: w2472 -> [_ w2482]
        tunnel: w2471 -> [_ w2481]
        frame False {
        }
        frame True {
          n871 = TCP Close Connection(connection ID=w2482, error in (no error)=w2481) -> ()  [unwired: 1 in, 2 out]
        }
      }
      n872 = case shown="True" w2476 {
        tunnel: w2475 -> [_ w2484]
        tunnel: w2474 -> [_ w2483]
        frame False {
        }
        frame True {
          n873 = call <vilib>:"Close Session.vi"("session handle"=w2484, "error in (no error)"=w2483) -> ()  [unwired: 13 in, 1 out]
        }
      }
    }
  }
  n874 = Flush Stream(8:w1, 11:w2) -> (0:w3:errorcluster, 3:w4:refnum<k21>)  [unwired: 2 in, 1 out]
  n875 = Flush Stream(8:w13, 11:w14) -> (0:w15:errorcluster, 3:w16:refnum<k21>)  [unwired: 2 in, 1 out]
  n876 = Destroy Stream Endpoint(8:w3, 11:w4) -> ()  [unwired: 1 out]
  n877 = Destroy Stream Endpoint(8:w15, 11:w16) -> ()  [unwired: 1 out]
